vi "WVDIAL+HSRL_v3.0.vi"() -> ()   [LabVIEW 2012]
uses:
  C:/Users/H2ODial/Desktop/Shared Telescope WV DIAL Code/Libraries and VIs/PowerMeterCommands.dll
  Shared Telescope WV DIAL Code/Libraries and VIs/PowerMeterCommands.dll
  <vilib>/DAQmx/write.llb/DAQmx Write (Digital 1D Bool NChan 1Samp 1Line).vi
  <vilib>/DAQmx/miscellaneous.llb/DAQmx Fill In Error Info.vi
  <vilib>/Analysis/baseanly.llb/Mean (DBL).vi
  NCAR_DIAL_Labview/AMCS_Data.vi
  Libraries and VIs/Scalar_Data.vi
  <vilib>/Analysis/NI_AALBase.lvlib
  Libraries and VIs/Scalar_Data_2.vi
  Libraries and VIs/Scalar_Data_4.vi
  Libraries and VIs/Scalar_Data_3.vi
  Shared Telescope WV DIAL Code/bristol/CLDevIFace.dll
panel:
  out "FileHour":i32=15
  out "L_Count":i32=27488
  out "background start":u32=534
  in  "Tab Control 2":enum32{"WV ND narrow", "WV ND wide"}(tab)
  out "CH3 RingBuffer long":dbl[][](array[numeric])
  out "CH3 RingBuffer short":dbl[][](array[numeric])
  in  "?":T1(tab)=enum."Raw Counts combined"
  out "NRB":dbl[][](graph) caption="Water Vapor Number Density"
  out "NRB 2":dbl[][](graph) caption="Water Vapor Number Density"
  out "CH 1 (WV off) counts display":dbl[][](graph) caption="Water Vapor Number Density"
  out "CH 3 (HSRL comb) counts display":dbl[][](graph)=[[164.8800000000001, 18.88000000000011, -33.11999999999989, 47.88000000000011, 38.88000000000011, 9.88000000000011, -16.11999999999989, 5.880000000000109, 22.88000000000011, 52.88000000000011, 66.88000000000011, -8.11999999999989, 61.88000000000011, 39.88000000000011, 9.88000000000011, 43.88000000000011, 140.8800000000001, 54.88000000000011, 74.88000000000011, 70.88000000000011, 124.88000000000011, 78.88000000000011, 153.8800000000001, 125.88000000000011, 85.88000000000011, 158.8800000000001, 111.88000000000011, 58.88000000000011, 147.8800000000001, 45.88000000000011, 165.8800000000001, 52.88000000000011, 53.88000000000011, 74.88000000000011, 82.88000000000011, 122.88000000000011, 140.8800000000001, 99.88000000000011, 56.88000000000011, 185.8800000000001, 145.8800000000001, 78.88000000000011, 202.8800000000001, 100.88000000000011, 82.88000000000011, 137.8800000000001, 111.88000000000011, 148.8800000000001, 115.88000000000011, 68.88000000000011, 97.88000000000011, 143.8800000000001, 78.88000000000011, 196.8800000000001, 128.8800000000001, 253.8800000000001, 223.8800000000001, 537.8800000000001, 1045.88, 1637.88, 2013.88, 2171.88, 2511.88, 3252.88, 4089.88, 4490.88, 4802.88, 5302.88, 6838.88, 8530.880000000001, 9591.880000000001, 9526.880000000001, 8480.880000000001, 7901.88, 7867.88, 8171.88, 7794.88, 6264.88, 4513.88, 3105.88, 2225.88, 1878.88, 1881.88, 2124.88, 3090.88, 6012.88, 9343.880000000001, 11636.880000000001, 12784.880000000001, 11600.880000000001, 9980.880000000001, 8400.880000000001, 7022.88, 5983.88, 4614.88, 3348.88, 2472.88, 1514.88, 1053.88, 613.8800000000001, 658.8800000000001, 640.8800000000001, 586.8800000000001, 476.8800000000001, 200.8800000000001, 138.8800000000001, 158.8800000000001, -26.11999999999989, 129.8800000000001, 51.88000000000011, -45.11999999999989, -3.119999999999891, -4.119999999999891, 18.88000000000011, 23.88000000000011, -48.11999999999989, -32.11999999999989, -37.11999999999989, -7.119999999999891, -42.11999999999989, 74.88000000000011, 24.88000000000011, -21.11999999999989, -24.11999999999989, -4.119999999999891, -10.11999999999989, -22.11999999999989, -51.11999999999989, 79.88000000000011, -10.11999999999989, -82.11999999999989, -30.11999999999989, -1.1199999999998909, -31.11999999999989, -17.11999999999989, -7.119999999999891, -33.11999999999989, -10.11999999999989, -11.11999999999989, -35.11999999999989, -5.119999999999891, 75.88000000000011, -21.11999999999989, 31.88000000000011, -31.11999999999989, -16.11999999999989, -7.119999999999891, 43.88000000000011, -49.11999999999989, -72.11999999999989, 30.88000000000011, -12.11999999999989, 8.88000000000011, -15.11999999999989, -35.11999999999989, 53.88000000000011, 10.88000000000011, -39.11999999999989, 5.880000000000109, 16.88000000000011, -30.11999999999989, 25.88000000000011, -57.11999999999989, -54.11999999999989, 16.88000000000011, -50.11999999999989, 1.8800000000001091, -20.11999999999989, 19.88000000000011, -79.11999999999989, 50.88000000000011, -84.11999999999989, 8.88000000000011, -31.11999999999989, -27.11999999999989, 57.88000000000011, -45.11999999999989, 65.88000000000011, -45.11999999999989, -100.11999999999989, -2.119999999999891, -23.11999999999989, 60.88000000000011, -19.11999999999989, 12.88000000000011, -66.11999999999989, -76.11999999999989, -29.11999999999989, -31.11999999999989, -67.11999999999989, -3.119999999999891, -28.11999999999989, -46.11999999999989, -18.11999999999989, -21.11999999999989, 4.880000000000109, 14.88000000000011, -29.11999999999989, 54.88000000000011, 12.88000000000011, -38.11999999999989, -62.11999999999989, -35.11999999999989, 28.88000000000011, 8.88000000000011, -28.11999999999989, -14.11999999999989, 7.880000000000109, 32.88000000000011, 7.880000000000109, 3.880000000000109, 6.880000000000109, -56.11999999999989, -59.11999999999989, -18.11999999999989, -35.11999999999989, 22.88000000000011, -25.11999999999989, -2.119999999999891, -27.11999999999989, -4.119999999999891, 8.88000000000011, -82.11999999999989, -19.11999999999989, -58.11999999999989, -2.119999999999891, 6.880000000000109, -28.11999999999989, 35.88000000000011, -7.119999999999891, -45.11999999999989, -44.11999999999989, 4.880000000000109, -100.11999999999989, 40.88000000000011, -42.11999999999989, -72.11999999999989, -63.11999999999989, 52.88000000000011, -73.11999999999989, -35.11999999999989, -102.11999999999989, -22.11999999999989, -74.11999999999989, 64.88000000000011, 6.880000000000109, -37.11999999999989, -56.11999999999989, 16.88000000000011, 48.88000000000011, -28.11999999999989, 38.88000000000011, 69.88000000000011, -15.11999999999989, -41.11999999999989, 10.88000000000011, 39.88000000000011, 64.88000000000011, -67.11999999999989, 35.88000000000011, -25.11999999999989, 16.88000000000011, -58.11999999999989, -24.11999999999989, -35.11999999999989, 22.88000000000011, -25.11999999999989, -60.11999999999989, 18.88000000000011, 27.88000000000011, -31.11999999999989, 0.8800000000001091, -11.11999999999989, 5.880000000000109, 35.88000000000011, -13.11999999999989, -115.11999999999989, 55.88000000000011, -63.11999999999989, 45.88000000000011, -25.11999999999989, -46.11999999999989, -14.11999999999989, 18.88000000000011, -37.11999999999989, 40.88000000000011, -56.11999999999989, 71.88000000000011, -34.11999999999989, -11.11999999999989, 2.880000000000109, -77.11999999999989, -44.11999999999989, -44.11999999999989, -26.11999999999989, -111.11999999999989, 41.88000000000011, -64.11999999999989, 41.88000000000011, 47.88000000000011, -21.11999999999989, 43.88000000000011, -0.11999999999989086, -140.1199999999999, -27.11999999999989, -16.11999999999989, -24.11999999999989, -15.11999999999989, 25.88000000000011, -36.11999999999989, -3.119999999999891, -47.11999999999989, -33.11999999999989, -5.119999999999891, 41.88000000000011, -27.11999999999989, 19.88000000000011, -82.11999999999989, -63.11999999999989, 15.88000000000011, 19.88000000000011, 80.88000000000011, -15.11999999999989, 25.88000000000011, -48.11999999999989, -100.11999999999989, 13.88000000000011, 69.88000000000011, -75.11999999999989, 48.88000000000011, 59.88000000000011, -42.11999999999989, -2.119999999999891, 21.88000000000011, 11.88000000000011, -29.11999999999989, -28.11999999999989, 43.88000000000011, -61.11999999999989, -23.11999999999989, -21.11999999999989, -21.11999999999989, -57.11999999999989, -61.11999999999989, 1.8800000000001091, -91.11999999999989, -22.11999999999989, -48.11999999999989, 3.880000000000109, -39.11999999999989, -52.11999999999989, 9.88000000000011, 62.88000000000011, 14.88000000000011, -57.11999999999989, 15.88000000000011, -7.119999999999891, -53.11999999999989, 14.88000000000011, -3.119999999999891, -61.11999999999989, 34.88000000000011, 3.880000000000109, -46.11999999999989, -21.11999999999989, 57.88000000000011, -51.11999999999989, 15.88000000000011, -71.11999999999989, -92.11999999999989, 15.88000000000011, -13.11999999999989, -30.11999999999989, -24.11999999999989, -6.119999999999891, 59.88000000000011, 12.88000000000011, -41.11999999999989, -5.119999999999891, 43.88000000000011, 32.88000000000011, -21.11999999999989, -65.11999999999989, -18.11999999999989, -27.11999999999989, 43.88000000000011, 14.88000000000011, -83.11999999999989, 11.88000000000011, -30.11999999999989, -34.11999999999989, -5.119999999999891, -30.11999999999989, -13.11999999999989, -15.11999999999989, -36.11999999999989, 23.88000000000011, 65.88000000000011, -37.11999999999989, -54.11999999999989, -31.11999999999989, -66.11999999999989, -96.11999999999989, -1.1199999999998909, -2.119999999999891, -7.119999999999891, -5.119999999999891, 46.88000000000011, -8.11999999999989, -23.11999999999989, 29.88000000000011, -14.11999999999989, 20.88000000000011, -14.11999999999989, 3.880000000000109, 13.88000000000011, 38.88000000000011, -45.11999999999989, -16.11999999999989, 8.88000000000011, 19.88000000000011, 27.88000000000011, -57.11999999999989, -9.11999999999989, 35.88000000000011, -37.11999999999989, -22.11999999999989, -12.11999999999989, -1.1199999999998909, -27.11999999999989, 74.88000000000011, 9.88000000000011, 30.88000000000011, -72.11999999999989, 36.88000000000011, 9.88000000000011, -43.11999999999989, -65.11999999999989, -78.11999999999989, -50.11999999999989, -29.11999999999989, -51.11999999999989, -43.11999999999989, -4.119999999999891, -42.11999999999989, 6.880000000000109, -26.11999999999989, -56.11999999999989, -4.119999999999891, 5.880000000000109, -58.11999999999989, 14.88000000000011, 65.88000000000011, 32.88000000000011, 13.88000000000011, 7.880000000000109, 4.880000000000109, 85.88000000000011, 16.88000000000011, -23.11999999999989, -71.11999999999989, -98.11999999999989, -26.11999999999989, -25.11999999999989, 34.88000000000011, 80.88000000000011, 49.88000000000011, -32.11999999999989, -17.11999999999989, -15.11999999999989, -9.11999999999989, -53.11999999999989, 36.88000000000011, 13.88000000000011, -31.11999999999989, 26.88000000000011, 2.880000000000109, 14.88000000000011, -12.11999999999989, 14.88000000000011, -28.11999999999989, -35.11999999999989, 25.88000000000011, 33.88000000000011, -47.11999999999989, -32.11999999999989, -45.11999999999989, 66.88000000000011, -43.11999999999989, 58.88000000000011, -68.11999999999989, -39.11999999999989, -20.11999999999989, 64.88000000000011, 54.88000000000011, 35.88000000000011, -53.11999999999989, -29.11999999999989, -53.11999999999989, 43.88000000000011, 24.88000000000011, -3.119999999999891, 6.880000000000109, 17.88000000000011, 25.88000000000011, -79.11999999999989, 8.88000000000011, -16.11999999999989, -47.11999999999989, -15.11999999999989, 23.88000000000011, -21.11999999999989, -26.11999999999989, -59.11999999999989, -15.11999999999989, 3.880000000000109, -11.11999999999989, -26.11999999999989, -30.11999999999989, -44.11999999999989, 80.88000000000011, -18.11999999999989, -5.119999999999891, 89.88000000000011, -36.11999999999989, -31.11999999999989, -30.11999999999989, 64.88000000000011, -26.11999999999989, -60.11999999999989, -55.11999999999989, -18.11999999999989, -49.11999999999989, -16.11999999999989, 20.88000000000011, -40.11999999999989, 13.88000000000011, -25.11999999999989, -34.11999999999989, -56.11999999999989, 67.88000000000011, 92.88000000000011, 18.88000000000011, 40.88000000000011, 25.88000000000011, -7.119999999999891, -38.11999999999989, 15.88000000000011, -5.119999999999891, -12.11999999999989, -11.11999999999989, 9.88000000000011, -31.11999999999989, 14.88000000000011, -20.11999999999989, 12.88000000000011, -45.11999999999989, 1.8800000000001091, -11.11999999999989, 0.0]] caption="Water Vapor Number Density"
  out "CH3 (HSRL combined) smooth S":dbl[](array[numeric])=[62.141379310344824, 31.529310344827586, 26.45172413793103, 26.020689655172408, 24.39999999999999, 25.809482758620682, 28.13275862068965, 30.72327586206896, 35.654310344827586, 40.106896551724134, 42.68448275862069, 45.83965517241379, 50.41293103448277, 53.92155172413794, 58.7448275862069, 63.206034482758625, 64.82672413793105, 70.36551724137932, 75.06810344827588, 79.69310344827588, 90.12844827586208, 89.98189655172415, 95.59396551724139, 98.72758620689656, 96.86982758620692, 104.16293103448277, 104.7189655172414, 108.15862068965518, 110.34827586206896, 110.03793103448278, 112.66293103448277, 113.2448275862069, 118.46465517241379, 120.49913793103448, 121.40431034482759, 122.76206896551723, 118.72327586206896, 119.26206896551724, 118.48620689655172, 115.50344827586207, 113.28362068965518, 109.46034482758621, 107.28793103448277, 108.00775862068966, 109.01206896551724, 110.56379310344826, 112.92586206896551, 111.15431034482758, 112.26206896551724, 110.39137931034482, 108.54655172413794, 107.52068965517242, 107.51206896551724, 108.56379310344828, 113.12844827586206, 132.2232758620689, 168.06379310344818, 227.73189655172405, 313.503448275862, 420.3051724137932, 557.5077586206897, 733.4172413793104, 957.8784482758622, 1222.7706896551722, 1531.6155172413792, 1906.124137931034, 2328.4689655172415, 2784.990517241379, 3250.253448275862, 3651.374137931034, 3951.3525862068964, 4160.1586206896545, 4293.706034482759, 4410.766379310345, 4497.8396551724145, 4535.326724137931, 4491.2146551724145, 4321.055172413793, 4089.9905172413796, 3843.3568965517243, 3603.6499999999996, 3435.6844827586206, 3356.533620689655, 3340.813793103448, 3401.6025862068964, 3410.710344827586, 3283.3913793103447, 3033.921551724138, 2651.697413793103, 2298.0767241379303, 2079.374137931034, 2052.356896551724, 2349.675862068965, 3259.007758620689, 4998.356896551724, 7120.921551724138, 9052.218965517242, 9987.766379310346, 9388.059482758621, 7746.292241379311, 5710.9043103448275, 3920.503448275862, 2805.1025862068964, 2455.3439655172415, 2695.826724137931, 3198.8396551724136, 3763.0379310344824, 4047.585344827586, 3857.25775862069, 3344.3525862068964, 2535.1844827586206, 1635.1758620689657, 914.5422413793103, 406.45603448275864, 132.35689655172413, 36.546551724137935, 10.374137931034486, -1.1129310344827599, -2.367241379310346, -4.225000000000001, -5.255172413793105, -4.341379310344829, -6.931896551724138, -8.68189655172414, -7.582758620689656, -9.660344827586208, -8.634482758620692, -7.255172413793105, -7.281034482758622, -5.319827586206898, -4.880172413793105, -4.02241379310345, -7.750862068965519, -10.212068965517242, -9.966379310344829, -9.518103448275863, -6.77241379310345, -2.466379310344829, -1.5698275862068978, -3.6689655172413804, -4.341379310344829, -4.056896551724138, -6.505172413793105, -6.3931034482758635, -6.522413793103449, -10.569827586206898, -7.444827586206897, -5.548275862068968, -6.229310344827588, -1.8543103448275875, -2.8284482758620704, -4.031034482758622, -1.6431034482758633, -6.837068965517242, -3.630172413793104, 0.6801724137931027, 3.1974137931034474, 8.839655172413792, 6.753448275862067, 5.003448275862068, 2.3439655172413785, 0.2405172413793091, -0.06982758620689772, -0.535344827586208, -0.0568965517241391, -1.699137931034484, -3.4362068965517256, -3.2767241379310357, -4.255172413793105, -3.656034482758622, -2.1301724137931046, -3.4620689655172425, -4.492241379310346, -2.7853448275862083, -2.8198275862068978, -1.2465517241379322, 0.7534482758620678, -0.2939655172413805, -0.8198275862068978, -1.1215517241379322, -2.7767241379310357, -0.7896551724137941, 0.964655172413792, 3.7706896551724127, 4.550862068965516, 2.503448275862068, 1.0206896551724127, -2.1732758620689667, -3.3672413793103457, -5.160344827586208, -6.591379310344829, -7.074137931034484, -5.410344827586208, -5.095689655172416, -4.457758620689656, -2.565517241379312, -2.4706896551724147, -1.4189655172413804, -1.031034482758622, -3.3112068965517256, -3.6387931034482768, -4.64741379310345, -2.983620689655173, -2.5482758620689667, -4.802586206896553, -2.9060344827586215, -4.410344827586208, -5.156034482758622, -3.7681034482758635, -4.156034482758622, -4.186206896551726, -2.134482758620691, -2.781034482758622, -2.4362068965517256, -2.89741379310345, -5.160344827586208, -5.54396551724138, -5.048275862068967, -9.156034482758622, -8.436206896551726, -6.975000000000001, -8.065517241379311, -3.276724137931036, -4.1991379310344845, -5.660344827586208, -6.703448275862071, -6.651724137931036, -5.949137931034484, -6.138793103448277, -6.686206896551726, -9.289655172413795, -10.57844827586207, -9.018103448275863, -8.48793103448276, -7.358620689655174, -5.64741379310345, -5.427586206896553, -3.3974137931034494, -1.8284482758620701, -2.7336206896551736, -1.9879310344827597, -4.0310344827586215, -3.3198275862068978, -3.7939655172413804, -5.319827586206898, -3.367241379310346, -3.6258620689655183, -2.970689655172415, -3.513793103448277, -5.009482758620691, -5.660344827586208, -6.151724137931035, -7.5181034482758635, -7.776724137931036, -8.186206896551726, -6.802586206896554, -3.9577586206896562, -2.8974137931034494, -1.1129310344827599, -1.552586206896553, -3.0181034482758635, -4.160344827586209, -4.888793103448277, -3.867241379310346, -2.3974137931034494, -1.2681034482758633, -1.927586206896553, -3.3198275862068978, -5.138793103448277, -5.4620689655172425, -5.108620689655174, -3.018103448275863, -3.0051724137931046, -3.996551724137932, -5.285344827586209, -8.457758620689656, -7.975000000000001, -7.1991379310344845, -5.177586206896553, -3.3112068965517256, -2.841379310344829, -3.466379310344829, -5.64741379310345, -6.742241379310347, -6.854310344827588, -5.483620689655174, -2.427586206896553, -0.25948275862069076, 0.18017241379310245, -1.1043103448275873, -4.9060344827586215, -6.121551724137932, -7.621551724137932, -5.660344827586208, -5.005172413793105, -5.561206896551725, -2.6991379310344836, -5.54396551724138, -4.048275862068967, -3.7379310344827594, -4.699137931034484, -2.4017241379310357, -2.6603448275862083, -4.246551724137932, -4.742241379310346, -4.272413793103449, -2.8241379310344836, 0.007758620689653939, -0.6301724137931046, -1.7250000000000012, -3.4491379310344836, -4.138793103448277, -1.6603448275862078, -4.035344827586208, -4.608620689655174, -6.125862068965518, -9.811206896551726, -8.93189655172414, -8.457758620689656, -6.845689655172415, -3.720689655172415, -1.4405172413793117, -1.3586206896551736, -1.7637931034482772, -3.565517241379312, -4.479310344827588, -1.6732758620689665, -0.3025862068965528, 2.6931034482758607, 4.83103448275862, 2.5982758620689648, 3.5120689655172397, 1.0379310344827573, 0.45603448275861946, 1.4344827586206885, -2.3974137931034494, -4.574137931034484, -4.686206896551725, -5.617241379310345, -4.000862068965518, -3.302586206896553, -3.86293103448276, -4.888793103448277, -7.207758620689656, -6.190517241379311, -6.00948275862069, -3.45344827586207, -1.8758620689655183, -2.720689655172415, -0.6474137931034494, -0.9620689655172425, -1.7551724137931046, 0.9215517241379299, -2.61293103448276, -3.9405172413793115, -2.45344827586207, -4.910344827586208, -4.160344827586208, -4.513793103448276, -4.479310344827587, -0.5008620689655185, -1.3241379310344839, -0.13017241379310468, -1.3025862068965528, -3.9706896551724147, -1.7724137931034492, -2.3801724137931046, -1.8758620689655183, -0.7508620689655184, -3.013793103448277, -2.5439655172413804, -1.2336206896551736, -1.0612068965517254, -2.539655172413794, -1.3974137931034498, -1.901724137931036, -2.2465517241379325, 0.9344827586206884, -1.746551724137932, -2.1948275862068973, -2.2939655172413804, -5.018103448275863, -4.888793103448277, -4.789655172413794, -5.388793103448277, -2.393103448275863, -0.7551724137931046, 2.1284482758620675, 1.6887931034482746, 0.30086206896551615, 0.8870689655172401, -0.4577586206896561, -1.3370689655172425, -0.1775862068965529, 0.701724137931033, -1.5956896551724151, -0.7206896551724149, 1.0551724137931022, -2.3068965517241393, -0.28534482758620805, -1.4793103448275875, -4.595689655172415, -3.970689655172415, -4.77241379310345, -3.5827586206896562, -4.341379310344829, -2.8068965517241393, -4.746551724137932, -3.2336206896551736, -1.4232758620689667, -1.0698275862068976, 0.3051724137931022, 0.19741379310344698, -0.6000000000000012, -4.074137931034484, -5.2120689655172425, -3.565517241379311, -3.341379310344829, -2.789655172413794, -1.720689655172415, -4.9060344827586215, -3.3801724137931046, -0.7508620689655183, -0.6344827586206908, -0.7508620689655184, -1.7637931034482772, -3.345689655172415, -1.20344827586207, 0.257758620689654, -2.1732758620689667, -3.7422413793103457, -3.7594827586206905, -4.518103448275863, -1.8801724137931046, -0.263793103448277, -2.32844827586207, -2.281034482758622, -1.6431034482758633, -0.6948275862068977, 0.24482758620689538, 1.4517241379310333, -1.4060344827586218, -3.8586206896551736, -5.66896551724138, -9.436206896551726, -8.535344827586208, -8.143103448275864, -5.957758620689656, -3.7336206896551736, -2.5310344827586215, -2.0267241379310357, -3.8758620689655183, -4.341379310344829, -4.664655172413794, -2.2939655172413804, -0.7551724137931045, -1.5482758620689665, -0.9362068965517253, -3.871551724137932, -3.2724137931034494, -4.54396551724138, -4.160344827586208, -2.6215517241379316, -4.005172413793105, -4.841379310344829, -5.638793103448277, -4.880172413793105, -5.052586206896553, -1.6991379310344839, -2.931896551724139, -0.9146551724137946, -1.6732758620689667, 0.17586206896551593, 1.9043103448275849, -2.0224137931034494, -1.9275862068965528, -3.281034482758622, -2.6948275862068973, -1.4663793103448288, -1.931896551724139, -2.8112068965517256, -2.5655172413793115, -2.95344827586207, -2.39741379310345, -1.3284482758620701, -3.6129310344827603, -1.9577586206896562, -1.406034482758622, 0.6499999999999986, 1.8913793103448264, 1.5077586206896538, 2.6887931034482744, 1.3913793103448264, -0.6862068965517252, -1.0353448275862078, -1.5913793103448286, -3.2551724137931046, -0.867241379310346, -3.466379310344829, -3.4017241379310352, -2.6387931034482768, -3.41896551724138, 0.22327586206896433, 0.024999999999998856, 0.6112068965517229, 1.1198275862068952, -0.01810344827586323, 0.23620689655172294, -0.5396551724137942, -0.3844827586206908, -1.5008620689655183, -2.268103448275863, -1.470689655172415, -0.5051724137931046, -3.2982758620689667, -3.89741379310345, -5.207758620689657, -5.64741379310345, -4.216379310344829, -2.664655172413794, -1.8974137931034494, -3.733620689655173, 0.3008620689655159, 0.447413793103447, -0.4706896551724151, -0.3974137931034496, -1.5741379310344839, -1.462068965517243, -1.7034482758620704, -0.5784482758620703, -2.1732758620689667, -2.7508620689655188, -1.216379310344829, -1.6215517241379325, 0.14568965517241256, -2.4146551724137946, -3.2724137931034494, -4.574137931034484, -5.039655172413794, -1.7637931034482768, -1.302586206896553, -0.22931034482758744, 0.016379310344826425, 2.1413793103448264, 3.2879310344827575, 7.0379310344827575, 7.378448275862068, 4.124137931034483, 4.352586206896551, -1.9448275862068978, -2.621551724137932, -0.9836206896551738, -3.315517241379312, 0.3094827586206884, -0.13448275862069092]
  out "CH3 (HSRL combined) smooth L":dbl[](array[numeric])=[58.96740223463691, 30.528854748603358, 26.30259776536313, 25.398966480446923, 26.19924581005587, 28.14128491620113, 31.917821229050297, 35.773966480446944, 38.952039106145264, 43.03164804469274, 45.771871508379874, 49.793519553072606, 54.13290502793292, 58.55399441340778, 63.422011173184316, 66.78723463687146, 70.81656424581001, 75.89198324022342, 81.08751396648043, 87.51000000000002, 94.17550279329615, 96.72298882681572, 99.86963687150848, 102.128715083799, 102.95483240223473, 106.73346368715093, 109.06516759776547, 111.84729050279341, 113.71740223463698, 115.26628491620124, 116.84729050279341, 117.8682402234638, 120.69924581005597, 122.06446927374313, 121.85287709497219, 121.37173184357553, 120.16642458100571, 119.63569832402247, 120.57424581005598, 119.83053072625712, 118.6706145251398, 118.24393854748615, 117.05608938547499, 117.50441340782133, 117.44715083798894, 116.36614525139676, 115.9241061452515, 114.49114525139677, 113.32564245810067, 112.08891061452525, 110.22438547486043, 109.14268156424592, 108.67899441340792, 107.6636312849163, 107.48067039106155, 108.75092178770961, 113.20553072625711, 123.05748603351967, 138.2481284916202, 161.0498044692738, 195.15874301675976, 242.8947765363128, 307.6021787709496, 393.1147486033518, 510.0721508379887, 670.1713128491618, 886.0833240223462, 1157.165027932961, 1461.3277374301679, 1772.6559497206706, 2047.1084636871512, 2275.5742458100563, 2487.52466480447, 2717.0079050279337, 3005.227178770951, 3358.319357541901, 3782.7187988826836, 4288.426899441343, 4938.4653072625715, 5706.315167597768, 6396.585418994415, 6793.38150837989, 6685.923407821231, 6074.914329608941, 5150.7425418994435, 4146.376620111734, 3238.7278770949733, 2492.519078212291, 1941.3745251396651, 1591.3130726256984, 1403.3235474860332, 1331.2341620111729, 1334.692262569832, 1419.8410055865918, 1635.531648044692, 1933.3437988826804, 2246.5602793296075, 2466.9115363128476, 2500.166424581004, 2396.391983240222, 2204.0302513966467, 1983.4534357541888, 1790.1503631284907, 1649.0770391061444, 1564.5679608938538, 1492.7187988826809, 1414.2362569832394, 1292.0016201117312, 1113.9541340782118, 916.6587430167594, 700.9548324022344, 490.7655865921786, 310.70553072625694, 167.7208938547486, 75.49324022346364, 28.379413407821218, 9.123826815642452, 3.8605586592178742, 2.8221508379888243, 2.2250837988826784, 2.0972905027932933, 1.8787150837988795, 1.530949720670388, 0.16921787709497016, 0.8849999999999977, 0.4164245810055844, 0.5686592178770926, 1.1622346368715053, 0.6126536312849132, 0.7327653631284886, 0.559581005586589, 0.660837988826812, -0.4823184357541942, -0.9529888268156467, -1.351033519553077, -1.135949720670395, -0.23022346368715413, -0.09893854748603678, -0.01793296089385804, -0.4348324022346404, -0.7085754189944173, -0.33986033519553455, -0.1380446927374338, -0.7316201117318467, -0.1820391061452541, 0.5211731843575392, 1.4464525139664774, 4.6922625698323985, 8.21670391061452, 18.669217877094965, 40.91432960893853, 83.42829608938547, 154.14128491620113, 247.91363128491622, 355.9764804469274, 453.57005586592174, 521.1405865921787, 554.2865363128491, 557.3158659217877, 547.9485474860335, 538.4045530726257, 532.9282960893854, 531.5623743016758, 527.4764804469273, 519.1238268156424, 503.9632122905028, 478.56097765363126, 444.4164245810056, 403.6559497206704, 358.57354748603353, 310.4268994413408, 261.56377094972066, 212.2697765363129, 165.0700558659218, 121.86963687150842, 87.4946368715084, 61.542122905027924, 43.46391061452513, 34.2118156424581, 29.90175977653631, 27.326340782122905, 28.481368715083804, 34.119636871508376, 42.34798882681564, 51.39058659217876, 56.27885474860333, 54.19226256983239, 44.528156424581, 33.469497206703906, 21.27885474860335, 11.035139664804463, 4.852178770949717, 0.5030167597765325, -0.8838547486033554, -1.637346368715087, -1.8894413407821258, -2.0402793296089414, -1.2141620111731872, -2.103128491620116, -2.4941899441340825, -2.941117318435759, -4.0004748603352, -3.514441340782127, -3.8007541899441377, -3.942513966480451, -3.430642458100563, -3.0263128491620144, -2.916675977653635, -2.645027932960897, -3.1925139664804503, -3.1869273743016793, -2.8901396648044724, -3.1268715083798915, -3.0933519553072655, -3.1869273743016784, -3.2979608938547513, -4.374776536312853, -3.97533519553073, -3.894329608938551, -3.704385474860339, -2.1359497206703946, -2.020027932960897, -2.683435754189948, -2.6841340782122938, -2.5786871508379923, -3.0291061452514003, -2.5535474860335228, -2.59055865921788, -2.7679329608938574, -3.5703072625698358, -2.288184357541903, -2.0563407821229083, -1.3342737430167633, -1.1876256983240254, -2.2874860335195564, -1.8566201117318466, -2.2749162011173216, -1.4893016759776563, -0.9285474860335223, -1.6904189944134107, -0.9920949720670421, -1.1024301675977681, -1.1045251396648073, -0.4341340782122932, -2.0053631284916236, -2.0668156424581037, -2.637346368715087, -4.333575418994419, -4.084972067039112, -4.163184357541905, -4.462765363128497, -3.8000558659217916, -3.6478212290502827, -4.200195530726261, -4.091955307262574, -3.3217039106145294, -3.767234636871513, -3.218351955307266, -2.142932960893858, -1.722541899441344, -1.1408379888268183, -0.5926536312849189, -1.0367877094972096, -1.8461452513966505, -1.5954469273743042, -1.7916759776536337, -1.3538268156424607, -0.8761731843575447, -1.640139664804472, -1.8559217877095, -2.1939106145251426, -2.7483798882681594, -1.8698882681564275, -1.5067597765363157, -2.573798882681568, -1.8014525139664836, -1.9432122905027964, -2.209273743016763, -1.0884636871508406, -1.302849162011176, -1.2141620111731872, -1.6813407821229078, -1.876871508379891, -1.2846927374301702, -1.7036871508379916, -1.0172346368715113, -1.237905027932964, -1.4564804469273773, -0.7232402234636901, -0.6156983240223493, -0.5011731843575447, -0.5123463687150864, -0.29446927374301946, -0.462067039106148, -0.5409776536312876, -0.6031284916201144, -1.4913966480446954, -2.301452513966484, -2.2406983240223495, -2.5242178770949755, -2.45019553072626, -1.2351117318435783, -0.9020111731843603, -1.1506145251396676, -1.026312849162014, -1.2881843575419023, -1.5682122905027962, -1.5235195530726284, -0.6771508379888296, -0.6408379888268183, -0.6254748603351983, -0.6687709497206733, -0.5675139664804496, -1.0758938547486059, -1.1436312849162036, -0.8964245810055891, -2.6869273743016784, -3.1401396648044724, -3.064720670391065, -2.3098324022346404, -1.7958659217877129, -0.9879050279329638, -0.8021508379888297, -1.5912569832402264, -1.7616480446927407, -1.9858100558659249, -2.3314804469273778, -2.448100558659221, -0.8712849162011199, -0.2979608938547512, -0.15829608938547757, -0.39293296089385726, -0.9739385474860361, -1.3559217877094998, -1.0465642458100584, -0.5221229050279357, -1.4446089385474892, -0.8929329608938581, -0.9557821229050311, -1.601033519553076, -1.7448882681564277, -2.132458100558662, -2.536089385474863, -1.708575418994416, -0.7525698324022374, -1.3698882681564273, -0.9886033519553099, -0.99628491620112, -1.4536871508379914, -1.658994413407824, -1.7770111731843605, -1.6003351955307292, -1.1687709497206733, -0.20229050279329883, -0.6624860335195558, -0.29516759776536583, -0.46206703910614794, -0.3307821229050306, -0.34055865921788, -1.1764525139664834, -1.1450279329608968, -1.3705865921787737, -0.29796089385475133, 0.30329608938547215, 0.8102793296089359, 0.9457541899441313, 0.8570670391061425, -0.031201117318438443, -0.4669553072625725, -0.8489385474860361, -0.8936312849162038, -0.9257541899441368, -0.8971229050279358, -1.0877653631284945, -1.1254748603351983, -0.6883240223463716, -0.5416759776536341, 0.0037150837988799527, -0.9055027932960922, -1.0772905027932989, -1.2008938547486059, -1.626871508379891, -0.9138826815642486, -1.4278491620111762, -1.1771508379888296, -1.6136033519553103, -1.5423743016759806, -0.6841340782122936, -1.21555865921788, -1.3985195530726289, -1.7686312849162045, -1.5905586592178804, -1.6701675977653663, -0.6359497206703938, 0.07843575418994136, -0.6548044692737458, -0.4208659217877122, -0.3943296089385502, -0.9257541899441368, -0.462067039106148, -0.8643016759776563, -1.4292458100558685, -1.5835754189944158, -2.0996368715083826, -2.240698324022349, -2.198798882681567, -2.2490782122905055, -2.397821229050282, -1.3161173184357569, -0.6513128491620137, -0.7274301675977679, 0.18737430167597494, 0.21810055865921515, 0.6294134078212263, 0.4953351955307237, -0.4669553072625734, 0.155251396648041, -0.7406983240223501, -1.0249162011173223, -0.48511173184357875, -0.932737430167601, -0.05703910614525454, 0.31307262569832106, -0.23860335195531002, -1.0228212290502823, -1.5263128491620142, -0.8279888268156453, -0.12826815642458378, 1.060977653631282, -0.045167597765366274, -1.0339944134078247, -0.9976815642458136, -2.492793296089389, -1.8887430167597796, -1.3314804469273769, -1.626871508379891, -0.7358100558659244, -0.33287709497206974, -0.0039664804469300985, 0.26279329608938273, -0.12058659217877371, 0.33192737430167324, -0.4390223463687179, -0.9166759776536342, -1.388044692737433, -2.557737430167601, -3.277011173184361, -2.368491620111735, -2.0982402234636903, -1.675055865921791, -0.41877094972067314, -1.2895810055865948, -1.7204469273743044, -1.1464245810055893, -1.6638826815642487, -0.6841340782122931, -0.34125698324022613, -0.9201675977653657, -0.7574581005586618, -0.6541061452513992, -1.3810614525139697, 0.003715083798879082, -0.011648044692741, -0.6855307262569867, 0.038631284916197994, -1.23860335195531, -0.4969832402234664, 0.25441340782122623, 0.44156424581005305, 0.17340782122904752, 0.6992458100558631, 0.6189385474860307, 1.0630726256983212, 1.7900279329608912, 1.5651675977653605, 0.9443575418994384, 1.6768994413407792, 2.4792737430167566, 2.402458100558656, 1.0351396648044655, -0.02910614525140011, -0.9222625698324055, -1.5402793296089416, -0.2427932960893882, 0.023268156424578273, -0.16737430167598039, -0.06122905027933234, 0.3843016759776509, -0.08706703910614796, 0.3214525139664777, 0.45483240223463417, 0.5937988826815616, 1.5016201117318408, 0.5058100558659189, 0.9338826815642429, 0.6671229050279301, -0.26094972067039396, 0.31377094972066766, -0.028407821229053054, -0.2504748603351983, 0.7648882681564216, 2.146871508379885, 2.530949720670388, 3.4660055865921757, 2.765586592178768, 1.6901675977653603, 1.3766201117318406, 0.6035754189944106, -0.19879888268156753, -0.3985195530726289, -0.8133240223463719, -1.5109497206703946, -1.3566201117318468, -1.4006145251396678, -2.1939106145251435, -1.5968435754189976, -0.8950279329608972, -0.1694692737430209, 0.7998044692737394, 1.4192178770949686, 1.0218715083798846, 0.2243854748603325, 1.0861173184357515, 0.7111173184357517, 1.0728491620111706, 1.2579050279329582, 0.571452513966478, 0.3514804469273715, 0.7704748603351927, 0.74603351955307, 0.1824860335195504, -0.4425139664804497, -1.0367877094972096, -1.0968435754189971, -0.869189944134081, -0.9851117318435784, -0.7777094972067068, -1.4697486033519582, -1.1694692737430197, -0.7832960893854776, -0.5675139664804496, 0.46391061452513693, -0.031201117318438498, 0.7732681564245782, 1.4171229050279304, 1.4513407821229025, 2.463212290502791, 1.8319273743016735, 1.0574860335195506, 0.5518994413407796, 0.16502793296089113, 0.5044134078212263, -0.34614525139665087, -0.08357541899441631, -0.5032681564245839]
  out "CH3 Bin Readings":dbl[](array[numeric])=[2030.0, 1884.0, 1832.0, 1913.0, 1904.0, 1875.0, 1849.0, 1871.0, 1888.0, 1918.0, 1932.0, 1857.0, 1927.0, 1905.0, 1875.0, 1909.0, 2006.0, 1920.0, 1940.0, 1936.0, 1990.0, 1944.0, 2019.0, 1991.0, 1951.0, 2024.0, 1977.0, 1924.0, 2013.0, 1911.0, 2031.0, 1918.0, 1919.0, 1940.0, 1948.0, 1988.0, 2006.0, 1965.0, 1922.0, 2051.0, 2011.0, 1944.0, 2068.0, 1966.0, 1948.0, 2003.0, 1977.0, 2014.0, 1981.0, 1934.0, 1963.0, 2009.0, 1944.0, 2062.0, 1994.0, 2119.0, 2089.0, 2403.0, 2911.0, 3503.0, 3879.0, 4037.0, 4377.0, 5118.0, 5955.0, 6356.0, 6668.0, 7168.0, 8704.0, 10396.0, 11457.0, 11392.0, 10346.0, 9767.0, 9733.0, 10037.0, 9660.0, 8130.0, 6379.0, 4971.0, 4091.0, 3744.0, 3747.0, 3990.0, 4956.0, 7878.0, 11209.0, 13502.0, 14650.0, 13466.0, 11846.0, 10266.0, 8888.0, 7849.0, 6480.0, 5214.0, 4338.0, 3380.0, 2919.0, 2479.0, 2524.0, 2506.0, 2452.0, 2342.0, 2066.0, 2004.0, 2024.0, 1839.0, 1995.0, 1917.0, 1820.0, 1862.0, 1861.0, 1884.0, 1889.0, 1817.0, 1833.0, 1828.0, 1858.0, 1823.0, 1940.0, 1890.0, 1844.0, 1841.0, 1861.0, 1855.0, 1843.0, 1814.0, 1945.0, 1855.0, 1783.0, 1835.0, 1864.0, 1834.0, 1848.0, 1858.0, 1832.0, 1855.0, 1854.0, 1830.0, 1860.0, 1941.0, 1844.0, 1897.0, 1834.0, 1849.0, 1858.0, 1909.0, 1816.0, 1793.0, 1896.0, 1853.0, 1874.0, 1850.0, 1830.0, 1919.0, 1876.0, 1826.0, 1871.0, 1882.0, 1835.0, 1891.0, 1808.0, 1811.0, 1882.0, 1815.0, 1867.0, 1845.0, 1885.0, 1786.0, 1916.0, 1781.0, 1874.0, 1834.0, 1838.0, 1923.0, 1820.0, 1931.0, 1820.0, 1765.0, 1863.0, 1842.0, 1926.0, 1846.0, 1878.0, 1799.0, 1789.0, 1836.0, 1834.0, 1798.0, 1862.0, 1837.0, 1819.0, 1847.0, 1844.0, 1870.0, 1880.0, 1836.0, 1920.0, 1878.0, 1827.0, 1803.0, 1830.0, 1894.0, 1874.0, 1837.0, 1851.0, 1873.0, 1898.0, 1873.0, 1869.0, 1872.0, 1809.0, 1806.0, 1847.0, 1830.0, 1888.0, 1840.0, 1863.0, 1838.0, 1861.0, 1874.0, 1783.0, 1846.0, 1807.0, 1863.0, 1872.0, 1837.0, 1901.0, 1858.0, 1820.0, 1821.0, 1870.0, 1765.0, 1906.0, 1823.0, 1793.0, 1802.0, 1918.0, 1792.0, 1830.0, 1763.0, 1843.0, 1791.0, 1930.0, 1872.0, 1828.0, 1809.0, 1882.0, 1914.0, 1837.0, 1904.0, 1935.0, 1850.0, 1824.0, 1876.0, 1905.0, 1930.0, 1798.0, 1901.0, 1840.0, 1882.0, 1807.0, 1841.0, 1830.0, 1888.0, 1840.0, 1805.0, 1884.0, 1893.0, 1834.0, 1866.0, 1854.0, 1871.0, 1901.0, 1852.0, 1750.0, 1921.0, 1802.0, 1911.0, 1840.0, 1819.0, 1851.0, 1884.0, 1828.0, 1906.0, 1809.0, 1937.0, 1831.0, 1854.0, 1868.0, 1788.0, 1821.0, 1821.0, 1839.0, 1754.0, 1907.0, 1801.0, 1907.0, 1913.0, 1844.0, 1909.0, 1865.0, 1725.0, 1838.0, 1849.0, 1841.0, 1850.0, 1891.0, 1829.0, 1862.0, 1818.0, 1832.0, 1860.0, 1907.0, 1838.0, 1885.0, 1783.0, 1802.0, 1881.0, 1885.0, 1946.0, 1850.0, 1891.0, 1817.0, 1765.0, 1879.0, 1935.0, 1790.0, 1914.0, 1925.0, 1823.0, 1863.0, 1887.0, 1877.0, 1836.0, 1837.0, 1909.0, 1804.0, 1842.0, 1844.0, 1844.0, 1808.0, 1804.0, 1867.0, 1774.0, 1843.0, 1817.0, 1869.0, 1826.0, 1813.0, 1875.0, 1928.0, 1880.0, 1808.0, 1881.0, 1858.0, 1812.0, 1880.0, 1862.0, 1804.0, 1900.0, 1869.0, 1819.0, 1844.0, 1923.0, 1814.0, 1881.0, 1794.0, 1773.0, 1881.0, 1852.0, 1835.0, 1841.0, 1859.0, 1925.0, 1878.0, 1824.0, 1860.0, 1909.0, 1898.0, 1844.0, 1800.0, 1847.0, 1838.0, 1909.0, 1880.0, 1782.0, 1877.0, 1835.0, 1831.0, 1860.0, 1835.0, 1852.0, 1850.0, 1829.0, 1889.0, 1931.0, 1828.0, 1811.0, 1834.0, 1799.0, 1769.0, 1864.0, 1863.0, 1858.0, 1860.0, 1912.0, 1857.0, 1842.0, 1895.0, 1851.0, 1886.0, 1851.0, 1869.0, 1879.0, 1904.0, 1820.0, 1849.0, 1874.0, 1885.0, 1893.0, 1808.0, 1856.0, 1901.0, 1828.0, 1843.0, 1853.0, 1864.0, 1838.0, 1940.0, 1875.0, 1896.0, 1793.0, 1902.0, 1875.0, 1822.0, 1800.0, 1787.0, 1815.0, 1836.0, 1814.0, 1822.0, 1861.0, 1823.0, 1872.0, 1839.0, 1809.0, 1861.0, 1871.0, 1807.0, 1880.0, 1931.0, 1898.0, 1879.0, 1873.0, 1870.0, 1951.0, 1882.0, 1842.0, 1794.0, 1767.0, 1839.0, 1840.0, 1900.0, 1946.0, 1915.0, 1833.0, 1848.0, 1850.0, 1856.0, 1812.0, 1902.0, 1879.0, 1834.0, 1892.0, 1868.0, 1880.0, 1853.0, 1880.0, 1837.0, 1830.0, 1891.0, 1899.0, 1818.0, 1833.0, 1820.0, 1932.0, 1822.0, 1924.0, 1797.0, 1826.0, 1845.0, 1930.0, 1920.0, 1901.0, 1812.0, 1836.0, 1812.0, 1909.0, 1890.0, 1862.0, 1872.0, 1883.0, 1891.0, 1786.0, 1874.0, 1849.0, 1818.0, 1850.0, 1889.0, 1844.0, 1839.0, 1806.0, 1850.0, 1869.0, 1854.0, 1839.0, 1835.0, 1821.0, 1946.0, 1847.0, 1860.0, 1955.0, 1829.0, 1834.0, 1835.0, 1930.0, 1839.0, 1805.0, 1810.0, 1847.0, 1816.0, 1849.0, 1886.0, 1825.0, 1879.0, 1840.0, 1831.0, 1809.0, 1933.0, 1958.0, 1884.0, 1906.0, 1891.0, 1858.0, 1827.0, 1881.0, 1860.0, 1853.0, 1854.0, 1875.0, 1834.0, 1880.0, 1845.0, 1878.0, 1820.0, 1867.0, 1854.0]
  out "CH2 (molecular) smoothed":dbl[](array[numeric])=[7.959767441860434, -0.34643410852716383, 1.2349612403100454, 2.0004651162790377, -2.3193023255814276, -0.15844961240313304, -0.36387596899228014, -0.43170542635662146, 4.03534883720927, 4.942325581395316, 7.733023255813921, 6.4830232558139205, 7.05472868217051, 8.40550387596896, 9.287286821705393, 13.316356589147254, 15.479147286821672, 21.091550387596868, 24.225271317829428, 28.459767441860436, 34.8841860465116, 37.20589147286819, 42.33767441860463, 49.87449612403099, 54.79891472868216, 58.36480620155038, 57.944263565891475, 57.00046511627907, 55.21170542635659, 54.924883720930225, 58.93457364341084, 57.61868217054263, 59.86286821705426, 62.04310077519379, 59.6884496124031, 63.67682170542634, 61.143875968992226, 63.508217054263525, 63.37449612403097, 61.40162790697672, 61.277596899224775, 58.775658914728666, 59.65937984496123, 58.11480620155037, 60.07217054263565, 60.26790697674417, 58.67488372093021, 59.19813953488371, 58.19813953488371, 55.494651162790696, 55.37255813953488, 56.771782945736426, 55.47914728682169, 54.24852713178293, 53.63806201550386, 51.012093023255794, 50.7950387596899, 49.03728682170541, 51.88031007751937, 54.56441860465115, 60.58767441860464, 72.16713178294572, 79.50046511627903, 92.11674418604646, 108.56829457364333, 130.47139534883715, 162.59155038759684, 202.34155038759678, 250.81829457364336, 300.453953488372, 345.1128682170542, 383.97720930232555, 408.5896124031008, 426.54310077519375, 449.8105426356589, 473.3609302325582, 504.32798449612403, 553.2272093023255, 626.2117054263565, 733.031472868217, 844.4055038759691, 908.4849612403102, 882.6806976744186, 760.9074418604652, 592.5004651162791, 442.92100775193796, 340.59542635658914, 286.4927131782946, 262.71558139534875, 245.7872868217053, 239.9268217054262, 237.23108527131768, 231.15937984496108, 213.61093023255796, 189.3221705426355, 161.92875968992234, 134.20395348837195, 107.43651162790687, 77.39387596899216, 46.87062015503871, 23.037286821705404, 7.008217054263534, -2.1080620155039083, -1.4220155038760016, -4.222403100775226, -1.8464341085271636, -2.5634883720930555, -6.7010852713178615, -5.662325581395382, -4.303798449612435, -1.4472093023256134, 0.5818604651162469, -0.673953488372125, -5.377441860465149, -7.865813953488405, -8.96465116279073, -8.94139534883724, -9.610000000000031, -10.42589147286825, -9.228217054263597, -7.5925581395349155, -3.5344186046511945, -3.95496124031011, -3.97434108527135, -4.910387596899257, -8.332868217054296, -7.080930232558172, -10.288294573643444, -10.338682170542668, -8.203023255813985, -5.976279069767474, -4.098372093023288, -4.786356589147319, -6.230155038759722, -8.803798449612435, -7.852248062015535, -6.722403100775225, -6.735968992248094, -6.011162790697706, -7.555736434108559, -8.695271317829489, -7.024728682170574, -8.047984496124062, -6.2592248062015825, -5.538294573643443, -4.7592248062015825, -4.187519379844993, -6.03248062015507, -6.538294573643443, -6.261162790697707, -4.3464341085271645, -3.931705426356621, -5.547984496124063, -5.960775193798482, -5.040232558139568, -4.201085271317862, 1.0566666666666347, 0.7775968992247739, -2.2689147286822022, -1.5867441860465434, -6.098372093023288, -5.0596124031008065, -4.848372093023288, -5.282480620155072, -3.807674418604683, -4.850310077519412, -2.980155038759722, -3.288294573643443, -1.2107751937984816, -1.3793798449612724, -4.639069767441892, -4.354186046511661, -5.906511627907009, -7.036356589147319, -5.590620155038792, -4.394883720930265, -4.666201550387629, -3.8134883720930555, -3.9568992248062336, -5.697209302325613, -4.834806201550419, -4.48403100775197, -6.168139534883753, -4.371627906976776, -5.222403100775226, -6.807674418604684, -5.282480620155071, -9.042170542635692, -11.315426356589178, -9.827054263565923, -9.770852713178327, -8.571240310077552, -8.020852713178327, -10.25341085271321, -9.232093023255846, -8.33480620155042, -5.68558139534887, -4.183643410852745, -4.995658914728715, -2.8503100775194117, -4.346434108527164, -1.162325581395381, -0.4103875968992571, -2.1720155038760014, 0.9113178294573323, -2.338682170542668, -3.920077519379877, -6.1758914728682495, -7.598372093023287, -6.03248062015507, -5.588682170542668, -3.1061240310077842, -4.367751937984528, -5.937519379844993, -4.499534883720962, -4.0925581395349155, -4.414263565891505, -3.117751937984528, -1.658449612403133, -2.534418604651195, -1.6410077519380168, -3.4685271317829782, -5.24372093023259, -4.313488372093056, -6.100310077519412, -2.6603875968992567, -1.3037984496124353, -2.185581395348869, 0.6787596899224484, -1.6758914728682495, -2.900697674418637, -3.679767441860497, -4.274728682170575, -5.406511627907008, -4.456899224806233, -3.982093023255846, -3.416201550387629, -0.4975968992248383, -2.2766666666666993, -1.3134883720930557, -3.0460465116279396, -3.078992248062048, -0.9258914728682491, -2.0092248062015825, -3.9375193798449937, -7.8173643410853035, -7.999534883720962, -8.520852713178327, -6.3425581395349155, -4.191395348837242, -4.7340310077519705, -0.20689922480623357, 0.7543410852712856, 0.9113178294573321, -0.08286821705429581, -5.057674418604684, -8.385193798449645, -9.098372093023288, -6.077054263565923, -2.2224031007752254, 0.35317829457361116, 0.9539534883720608, -1.284418604651195, -3.7669767441860786, -2.5111627906977065, -0.23209302325584624, -2.402635658914761, -2.710775193798482, -4.055736434108559, -4.52279069767445, -0.8696899224806521, -0.10806201550390804, 2.2834108527131463, 1.207829457364309, 0.3725581395348516, 1.6710077519379523, -0.3037984496124353, -1.1371317829457686, 0.07410852713175076, 0.07798449612399888, -0.282480620155071, -1.3774418604651486, -2.72434108527135, -1.338682170542668, -1.4607751937984819, 0.6729457364340764, 0.7233333333333014, -3.1332558139535207, -2.5751162790697997, -4.2882945736434435, -2.3251162790698006, -0.220465116279102, 0.6438759689922159, 2.2427131782945415, -0.43170542635662124, -2.1448837209302645, -2.598372093023288, -3.8386821705426684, -3.350310077519412, -1.1584496124031332, -1.6061240310077842, -1.3289922480620477, 0.008217054263533807, -1.5712403100775514, 0.023720930232526083, 0.8512403100774873, 0.22914728682167337, -2.9665891472868537, -3.466589147286854, -3.1506976744186366, -2.9413953488372417, 0.025658914728649895, 1.267906976744154, 1.459767441860433, 1.632248062015472, 3.6710077519379523, 0.23883720930229324, -1.0828682170542958, -1.3755038759690246, -2.84449612403104, -3.9258914728682495, -3.3173643410853035, -4.697209302325613, -5.747596899224838, -3.1100000000000323, -4.947209302325614, -5.158449612403133, -3.904573643410885, -3.9937209302325902, -3.2921705426356906, -2.2824806201550714, -0.5460465116279392, 1.8551162790697353, 2.8008527131782626, 3.3144186046511304, -0.5441085271318151, -4.947209302325613, -4.827054263565923, -5.055736434108558, -1.3289922480620477, -0.4006976744186368, 0.05860465116275851, 2.2892248062015184, -1.9762790697674741, -3.237906976744218, -5.3716279069767765, -6.985968992248094, -4.032480620155071, -1.476279069767474, 0.13224806201547173, -0.49178294573646625, -2.5499224806201872, -2.08480620155042, -4.009224806201583, -6.125503875969025, -6.538294573643443, -6.896821705426389, -6.6235658914729, -4.778604651162823, -1.782480620155071, -0.6313178294573967, 0.31248062015500655, 0.43651162790694464, -1.6196899224806522, -4.4762790697674735, -3.4762790697674744, -5.20496124031011, -4.654573643410885, -2.6855813953488696, -4.265038759689954, -0.8638759689922804, 0.03534883720927029, -1.340620155038792, 0.6613178294573321, -2.5693023255814276, -1.2689147286822027, 1.6962015503875647, 0.6729457364340763, 0.589612403100743, -1.4162015503876288, -4.111937984496157, -4.2049612403101095, -1.0014728682170866, 0.5566666666666344, 1.6089922480619834, 1.085736434108495, -2.0576744186046834, -1.9297674418604973, -1.561550387596931, -0.18945736434111754, 0.6690697674418283, 0.7601550387596578, -1.4123255813953808, -0.06155038759693121, -4.780542635658946, -3.598372093023287, 0.7097674418604338, -0.11968992248065169, 6.5741085271317505, 4.203953488372061, 1.878372093023224, 0.8977519379844642, 0.9132558139534561, 1.2950387596898902, 1.5159689922480297, 1.6303100775193475, 0.36286821705423145, -1.8851937984496447, -1.6158139534884044, -0.8328682170542958, -1.7669767441860789, 0.9151937984495802, -3.21465116279073, -6.131317829457396, -5.850310077519412, -6.885193798449644, -5.046046511627939, -5.8251162790698, -5.466589147286854, -3.644883720930265, -3.7844186046511945, -3.6623255813953812, -3.947209302325614, -4.598372093023288, -4.423953488372126, -2.6119379844961563, -0.3890697674418928, -0.04604651162793927, 0.008217054263533585, -0.22046511627910204, -2.852248062015536, -3.476279069767474, -2.0131007751938306, -1.805736434108559, 0.9035658914728362, -1.1448837209302645, -1.1642635658915048, 1.3744961240309757, -3.2960465116279387, -2.179767441860497, -3.36387596899228, -4.931705426356621, -2.1390697674418924, -0.12356589147290031, 2.9849612403100454, 2.9500775193798123, 3.3493023255813634, 1.8919379844960915, -2.040232558139567, -1.8348062015504198, 0.48883720930229346, 0.7465891472867897, 3.7058914728681853, 3.0334108527131463, 0.20782945736430886, -0.8968217054263887, -4.673953488372126, -4.772790697674451, -5.3968217054263885, -5.945271317829489, -3.226279069767474, -2.524728682170575, -3.487906976744218, -4.4510852713178615, -4.115813953488404, -4.5964341085271645, -3.3212403100775516, -0.5266666666666988, -2.3832558139535207, -2.034418604651195, 0.5469767441860145, 0.4171317829457044, 1.576046511627875, 1.566356589147255, 1.5043410852712857, -1.1933333333333658, -3.1836434108527456, -2.5499224806201872, -6.443333333333365, -4.555736434108559, -3.0227906976744503, -1.3037984496124349, -0.9917829457364662, -1.0964341085271636, -0.25147286821708636, -3.1468217054263885, -2.790232558139567, -2.1177519379845284, -2.1642635658915053, -3.040232558139567, -2.5615503875969314, 0.4655813953488046, -0.9840310077519705, 0.20007751937981255, 0.5760465116278746, -3.206899224806234, -0.6836434108527454, -0.6526356589147609, -1.4937209302325902, -0.4394573643411175, -0.9530232558139858, -1.6235658914729005, 0.17294573643407635, -1.912325581395381, -4.927829457364373, -3.7204651162791023, -7.092558139534916, -5.974341085271351, -4.080930232558172, -3.817364341085304, -0.2824806201550709, -3.710775193798482, -3.0441085271318156, -1.761162790697707, -3.2320930232558465, 1.967519379844929, 1.3124806201550065, -0.10418604651166005, 2.2562790697674098, 0.6283720930232237, 4.03534883720927, 1.159379844961208, 0.4365116279069442, -0.2282170542635984, -3.809612403100808, 1.1748837209302, 0.36286821705423106, -1.2049612403101102, -0.15457364341088498, -4.137131782945769, -3.1623255813953812, -1.6972093023256138, -1.4975968992248387, 2.8163565891472544, -1.036356589147319, 0.6380620155038437, 0.058604651162758564, -0.5014728682170864, 0.36674418604647974, 1.5508527131782626, 1.4888372093022935, -0.8910077519380166, 1.8899999999999677, 0.6128682170542313, 2.583798449612371, 2.409379844961208, 2.1438759689922158, 0.056666666666634447, -1.3580620155039083, -0.17007751937987714, -2.526666666666699, -0.8890697674418926, -0.3716279069767763, -1.4975968992248385, -0.06542635658917956]
  out "CH 2 Bin Readings":dbl[](array[numeric])=[4534.0, 4468.0, 4463.0, 4418.0, 4437.0, 4640.0, 4605.0, 4432.0, 4509.0, 4491.0, 4549.0, 4583.0, 4499.0, 4529.0, 4444.0, 4490.0, 4495.0, 4551.0, 4556.0, 4422.0, 4457.0, 4536.0, 4508.0, 4472.0, 4722.0, 4501.0, 4568.0, 4488.0, 4527.0, 4643.0, 4539.0, 4545.0, 4488.0, 4571.0, 4640.0, 4556.0, 4523.0, 4591.0, 4509.0, 4558.0, 4495.0, 4531.0, 4614.0, 4493.0, 4569.0, 4603.0, 4572.0, 4515.0, 4552.0, 4469.0, 4601.0, 4547.0, 4618.0, 4527.0, 4517.0, 4610.0, 4580.0, 4555.0, 4588.0, 4632.0, 4658.0, 4661.0, 4718.0, 4829.0, 4668.0, 4785.0, 4866.0, 4888.0, 5018.0, 4908.0, 5068.0, 5223.0, 5077.0, 4999.0, 4907.0, 5061.0, 5025.0, 4982.0, 4677.0, 4738.0, 4653.0, 4599.0, 4576.0, 4615.0, 4616.0, 4776.0, 4933.0, 5167.0, 5263.0, 5323.0, 5030.0, 5019.0, 4996.0, 4959.0, 4849.0, 4699.0, 4628.0, 4655.0, 4547.0, 4473.0, 4488.0, 4559.0, 4621.0, 4423.0, 4421.0, 4442.0, 4466.0, 4520.0, 4399.0, 4378.0, 4592.0, 4525.0, 4547.0, 4476.0, 4519.0, 4411.0, 4502.0, 4536.0, 4527.0, 4464.0, 4493.0, 4402.0, 4598.0, 4538.0, 4490.0, 4449.0, 4371.0, 4479.0, 4471.0, 4443.0, 4615.0, 4578.0, 4545.0, 4461.0, 4371.0, 4481.0, 4487.0, 4476.0, 4525.0, 4582.0, 4463.0, 4599.0, 4458.0, 4641.0, 4444.0, 4613.0, 4469.0, 4545.0, 4386.0, 4430.0, 4359.0, 4551.0, 4559.0, 4415.0, 4520.0, 4467.0, 4417.0, 4452.0, 4546.0, 4531.0, 4559.0, 4378.0, 4528.0, 4457.0, 4584.0, 4538.0, 4445.0, 4464.0, 4441.0, 4401.0, 4519.0, 4567.0, 4570.0, 4497.0, 4448.0, 4537.0, 4341.0, 4542.0, 4469.0, 4549.0, 4386.0, 4552.0, 4507.0, 4489.0, 4490.0, 4478.0, 4442.0, 4400.0, 4622.0, 4461.0, 4530.0, 4437.0, 4452.0, 4473.0, 4502.0, 4614.0, 4606.0, 4493.0, 4528.0, 4538.0, 4560.0, 4399.0, 4434.0, 4527.0, 4458.0, 4410.0, 4384.0, 4524.0, 4350.0, 4645.0, 4487.0, 4492.0, 4439.0, 4471.0, 4598.0, 4587.0, 4622.0, 4459.0, 4528.0, 4465.0, 4448.0, 4447.0, 4450.0, 4401.0, 4449.0, 4522.0, 4380.0, 4541.0, 4515.0, 4479.0, 4509.0, 4531.0, 4468.0, 4459.0, 4464.0, 4574.0, 4548.0, 4584.0, 4504.0, 4454.0, 4465.0, 4486.0, 4448.0, 4457.0, 4539.0, 4416.0, 4533.0, 4496.0, 4527.0, 4457.0, 4543.0, 4469.0, 4560.0, 4525.0, 4509.0, 4495.0, 4525.0, 4384.0, 4470.0, 4560.0, 4504.0, 4461.0, 4608.0, 4464.0, 4486.0, 4539.0, 4519.0, 4400.0, 4434.0, 4429.0, 4656.0, 4434.0, 4481.0, 4515.0, 4577.0, 4450.0, 4470.0, 4355.0, 4453.0, 4361.0, 4434.0, 4517.0, 4566.0, 4395.0, 4572.0, 4556.0, 4418.0, 4426.0, 4487.0, 4476.0, 4412.0, 4588.0, 4334.0, 4421.0, 4492.0, 4609.0, 4520.0, 4400.0, 4489.0, 4478.0, 4432.0, 4407.0, 4381.0, 4528.0, 4564.0, 4416.0, 4438.0, 4481.0, 4436.0, 4381.0, 4361.0, 4411.0, 4492.0, 4473.0, 4535.0, 4411.0, 4516.0, 4505.0, 4433.0, 4483.0, 4436.0, 4494.0, 4442.0, 4496.0, 4432.0, 4417.0, 4420.0, 4459.0, 4423.0, 4574.0, 4498.0, 4502.0, 4379.0, 4514.0, 4597.0, 4447.0, 4411.0, 4538.0, 4545.0, 4528.0, 4513.0, 4434.0, 4559.0, 4513.0, 4389.0, 4527.0, 4496.0, 4410.0, 4513.0, 4532.0, 4405.0, 4466.0, 4439.0, 4349.0, 4528.0, 4463.0, 4454.0, 4401.0, 4523.0, 4612.0, 4488.0, 4468.0, 4612.0, 4537.0, 4427.0, 4518.0, 4496.0, 4376.0, 4481.0, 4546.0, 4373.0, 4362.0, 4474.0, 4451.0, 4429.0, 4452.0, 4591.0, 4510.0, 4526.0, 4471.0, 4513.0, 4489.0, 4450.0, 4424.0, 4513.0, 4523.0, 4372.0, 4550.0, 4528.0, 4562.0, 4480.0, 4382.0, 4523.0, 4542.0, 4553.0, 4515.0, 4521.0, 4625.0, 4517.0, 4462.0, 4623.0, 4514.0, 4597.0, 4464.0, 4493.0, 4431.0, 4529.0, 4447.0, 4437.0, 4661.0, 4493.0, 4497.0, 4521.0, 4456.0, 4500.0, 4398.0, 4566.0, 4396.0, 4488.0, 4528.0, 4575.0, 4560.0, 4434.0, 4398.0, 4522.0, 4453.0, 4519.0, 4427.0, 4447.0, 4542.0, 4528.0, 4423.0, 4557.0, 4535.0, 4560.0, 4497.0, 4441.0, 4454.0, 4526.0, 4482.0, 4454.0, 4438.0, 4537.0, 4532.0, 4497.0, 4508.0, 4552.0, 4560.0, 4591.0, 4351.0, 4491.0, 4477.0, 4567.0, 4464.0, 4478.0, 4473.0, 4480.0, 4462.0, 4524.0, 4556.0, 4431.0, 4532.0, 4361.0, 4494.0, 4535.0, 4388.0, 4531.0, 4445.0, 4381.0, 4544.0, 4475.0, 4663.0, 4497.0, 4502.0, 4472.0, 4528.0, 4569.0, 4575.0, 4519.0, 4443.0, 4531.0, 4615.0, 4434.0, 4479.0, 4556.0, 4436.0, 4536.0, 4541.0, 4552.0, 4351.0, 4600.0, 4539.0, 4483.0, 4632.0, 4519.0, 4559.0, 4372.0, 4519.0, 4465.0, 4534.0, 4478.0, 4467.0, 4394.0, 4453.0, 4488.0, 4569.0, 4482.0, 4478.0, 4580.0, 4484.0, 4473.0, 4381.0, 4439.0, 4444.0, 4437.0, 4485.0, 4471.0, 4473.0, 4456.0, 4628.0, 4449.0, 4400.0, 4437.0, 4519.0, 4489.0, 4606.0, 4396.0, 4596.0, 4500.0, 4518.0, 4472.0, 4571.0, 4569.0, 4391.0, 4549.0, 4353.0, 4490.0, 4520.0, 4569.0, 4495.0, 4547.0, 4533.0, 4514.0, 4557.0, 4482.0, 4533.0, 4421.0, 4478.0, 4610.0, 4430.0, 4522.0, 4415.0, 4474.0, 4396.0, 4366.0, 4578.0, 4494.0, 4463.0, 4519.0]
  in  "stop":bool
  in  "Reset Average":bool=TRUE
  in  "Save Data?":bool=TRUE
  in  "Collect Data?":bool=TRUE
  in  "ILX Address":i32=6 min=0 step=1
  in  "Lambda On DBR Current":dbl=171.13999999999868
  in  "Lambda Off DBR Current":dbl=172.9499999999997
  in  "Tab Control":T2(tab)=enum."NRB"
  out "NRB plot":cluster{"Y":dbl[], "Y":dbl[]}[](graph)=[{"Y"=[], "Y"=[0.0375, 0.075, 0.11249999999999999, 0.15, 0.1875, 0.225, 0.26249999999999996, 0.3, 0.33749999999999997, 0.37499999999999994, 0.4125, 0.44999999999999996, 0.48749999999999993, 0.525, 0.5625, 0.6, 0.6375, 0.6749999999999999, 0.7124999999999999, 0.75, 0.7875, 0.825, 0.8624999999999999, 0.8999999999999999, 0.9374999999999999, 0.975, 1.0125, 1.05, 1.0875000000000001, 1.125, 1.1625, 1.2, 1.2375, 1.2750000000000001, 1.3125, 1.35, 1.3875, 1.425, 1.4625000000000001, 1.5, 1.5375, 1.575, 1.6125, 1.6500000000000001, 1.6875, 1.725, 1.7625, 1.8, 1.8375, 1.875, 1.9125, 1.95, 1.9875, 2.025, 2.0625, 2.1, 2.1375, 2.175, 2.2125, 2.25, 2.2875, 2.325, 2.3625, 2.4, 2.4375, 2.475, 2.5125, 2.55, 2.5875, 2.625, 2.6625, 2.7, 2.7375, 2.775, 2.8125, 2.85, 2.8875, 2.925, 2.9625, 3.0, 3.0375, 3.075, 3.1125, 3.15, 3.1875, 3.225, 3.2625, 3.3, 3.3375, 3.375, 3.4125, 3.45, 3.4875, 3.525, 3.5625, 3.6, 3.6374999999999997, 3.675, 3.7125, 3.75, 3.7875, 3.8249999999999997, 3.8625, 3.9, 3.9375, 3.975, 4.012499999999999, 4.05, 4.0874999999999995, 4.124999999999999, 4.1625, 4.199999999999999, 4.2375, 4.2749999999999995, 4.312499999999999, 4.35, 4.387499999999999, 4.425, 4.4624999999999995, 4.499999999999999, 4.5375, 4.574999999999999, 4.6125, 4.6499999999999995, 4.687499999999999, 4.725, 4.762499999999999, 4.8, 4.8374999999999995, 4.874999999999999, 4.9125, 4.949999999999999, 4.9875, 5.0249999999999995, 5.062499999999999, 5.1, 5.137499999999999, 5.175, 5.2124999999999995, 5.249999999999999, 5.2875, 5.324999999999999, 5.3625, 5.3999999999999995, 5.437499999999999, 5.475, 5.512499999999999, 5.55, 5.5874999999999995, 5.624999999999999, 5.6625, 5.699999999999999, 5.7375, 5.7749999999999995, 5.812499999999999, 5.85, 5.887499999999999, 5.925, 5.9624999999999995, 5.999999999999999, 6.0375, 6.074999999999999, 6.1125, 6.1499999999999995, 6.187499999999999, 6.225, 6.262499999999999, 6.3, 6.3374999999999995, 6.374999999999999, 6.4125, 6.449999999999999, 6.4875, 6.5249999999999995, 6.562499999999999, 6.6, 6.637499999999999, 6.675, 6.7124999999999995, 6.749999999999999, 6.7875, 6.824999999999999, 6.8625, 6.8999999999999995, 6.937499999999999, 6.975, 7.012499999999999, 7.05, 7.0874999999999995, 7.124999999999999, 7.1625, 7.199999999999999, 7.237499999999999, 7.2749999999999995, 7.312499999999999, 7.35, 7.387499999999999, 7.424999999999999, 7.4624999999999995, 7.499999999999999, 7.5375, 7.574999999999999, 7.612499999999999, 7.6499999999999995, 7.687499999999999, 7.725, 7.762499999999999, 7.799999999999999, 7.8374999999999995, 7.874999999999999, 7.9125, 7.949999999999999, 7.987499999999999, 8.025, 8.0625, 8.1, 8.1375, 8.174999999999999, 8.212499999999999, 8.25, 8.2875, 8.325, 8.362499999999999, 8.399999999999999, 8.4375, 8.475, 8.5125, 8.549999999999999, 8.587499999999999, 8.625, 8.6625, 8.7, 8.737499999999999, 8.774999999999999, 8.8125, 8.85, 8.8875, 8.924999999999999, 8.962499999999999, 9.0, 9.0375, 9.075, 9.112499999999999, 9.149999999999999, 9.1875, 9.225, 9.2625, 9.299999999999999, 9.337499999999999, 9.375, 9.4125, 9.45, 9.487499999999999, 9.524999999999999, 9.5625, 9.6, 9.6375, 9.674999999999999, 9.712499999999999, 9.75, 9.7875, 9.825, 9.862499999999999, 9.899999999999999, 9.9375, 9.975, 10.0125, 10.049999999999999, 10.087499999999999, 10.125, 10.1625, 10.2, 10.237499999999999, 10.274999999999999, 10.3125, 10.35, 10.3875, 10.424999999999999, 10.462499999999999, 10.5, 10.5375, 10.575, 10.612499999999999, 10.649999999999999, 10.6875, 10.725, 10.7625, 10.799999999999999, 10.837499999999999, 10.875, 10.9125, 10.95, 10.987499999999999, 11.024999999999999, 11.0625, 11.1, 11.1375, 11.174999999999999, 11.212499999999999, 11.25, 11.2875, 11.325, 11.362499999999999, 11.399999999999999, 11.4375, 11.475, 11.5125, 11.549999999999999, 11.587499999999999, 11.625, 11.6625, 11.7, 11.737499999999999, 11.774999999999999, 11.8125, 11.85, 11.8875, 11.924999999999999, 11.962499999999999, 12.0, 12.0375, 12.075, 12.112499999999999, 12.149999999999999, 12.1875, 12.225, 12.2625, 12.299999999999999, 12.337499999999999, 12.375, 12.4125, 12.45, 12.487499999999999, 12.524999999999999, 12.5625, 12.6, 12.6375, 12.674999999999999, 12.712499999999999, 12.75, 12.7875, 12.825, 12.862499999999999, 12.899999999999999, 12.9375, 12.975, 13.0125, 13.049999999999999, 13.087499999999999, 13.125, 13.1625, 13.2, 13.237499999999999, 13.274999999999999, 13.3125, 13.35, 13.3875, 13.424999999999999, 13.462499999999999, 13.5, 13.5375, 13.575, 13.612499999999999, 13.649999999999999, 13.6875, 13.725, 13.7625, 13.799999999999999, 13.837499999999999, 13.875, 13.9125, 13.95, 13.987499999999999, 14.024999999999999, 14.0625, 14.1, 14.1375, 14.174999999999999, 14.212499999999999, 14.25, 14.2875, 14.325, 14.362499999999999, 14.399999999999999, 14.437499999999998, 14.475, 14.5125, 14.549999999999999, 14.587499999999999, 14.624999999999998, 14.6625, 14.7, 14.737499999999999, 14.774999999999999, 14.812499999999998, 14.85, 14.8875, 14.924999999999999, 14.962499999999999, 14.999999999999998, 15.0375, 15.075, 15.112499999999999, 15.149999999999999, 15.187499999999998, 15.225, 15.2625, 15.299999999999999, 15.337499999999999, 15.374999999999998, 15.4125, 15.45, 15.487499999999999, 15.524999999999999, 15.562499999999998, 15.6, 15.6375, 15.674999999999999, 15.712499999999999, 15.749999999999998, 15.7875, 15.825, 15.862499999999999, 15.899999999999999, 15.937499999999998, 15.975, 16.0125, 16.05, 16.087500000000002, 16.125, 16.1625, 16.2, 16.2375, 16.275000000000002, 16.3125, 16.35, 16.3875, 16.425, 16.462500000000002, 16.5, 16.5375, 16.575, 16.6125, 16.650000000000002, 16.6875, 16.725, 16.7625, 16.8, 16.837500000000002, 16.875, 16.9125, 16.95, 16.9875, 17.025000000000002, 17.0625, 17.1, 17.1375, 17.175, 17.212500000000002, 17.25, 17.2875, 17.325, 17.3625, 17.400000000000002, 17.4375, 17.475, 17.5125, 17.55, 17.587500000000002, 17.625, 17.6625, 17.7, 17.7375, 17.775000000000002, 17.8125, 17.85, 17.8875, 17.925, 17.962500000000002, 18.0, 18.0375, 18.075, 18.1125, 18.150000000000002, 18.1875, 18.225, 18.2625, 18.3, 18.337500000000002, 18.375, 18.4125, 18.45, 18.4875, 18.525000000000002, 18.5625, 18.6, 18.6375, 18.675, 18.712500000000002, 18.75, 18.7875, 18.825, 18.8625, 18.900000000000002, 18.9375, 18.975, 19.0125, 19.05, 19.087500000000002, 19.125, 19.1625, 19.2, 19.2375, 19.275000000000002, 19.3125, 19.35, 19.3875, 19.425, 19.462500000000002, 19.5, 19.5375, 19.575, 19.6125, 19.650000000000002, 19.6875, 19.725, 19.7625, 19.8, 19.837500000000002, 19.875, 19.9125, 19.95, 19.9875, 20.025000000000002, 20.0625, 20.1, 20.1375, 20.175, 20.212500000000002, 20.25, 20.2875, 20.325, 20.3625, 20.400000000000002, 20.4375, 20.475, 20.5125, 20.55, 20.587500000000002, 20.625, 20.6625, 20.7, 20.7375, 20.775000000000002, 20.8125, 20.85, 20.8875, 20.925, 20.962500000000002, 21.0]}, ...(2 in all)]
  in  "background length":i32=25
  out "Correction":cluster{"Y":dbl[], "Y":dbl[]}[](graph)=[{"Y"=[], "Y"=[0.0375, 0.075, 0.11249999999999999, 0.15, 0.1875, 0.225, 0.26249999999999996, 0.3, 0.33749999999999997, 0.37499999999999994, 0.4125, 0.44999999999999996, 0.48749999999999993, 0.525, 0.5625, 0.6, 0.6375, 0.6749999999999999, 0.7124999999999999, 0.75, 0.7875, 0.825, 0.8624999999999999, 0.8999999999999999, 0.9374999999999999, 0.975, 1.0125, 1.05, 1.0875000000000001, 1.125, 1.1625, 1.2, 1.2375, 1.2750000000000001, 1.3125, 1.35, 1.3875, 1.425, 1.4625000000000001, 1.5, 1.5375, 1.575, 1.6125, 1.6500000000000001, 1.6875, 1.725, 1.7625, 1.8, 1.8375, 1.875, 1.9125, 1.95, 1.9875, 2.025, 2.0625, 2.1, 2.1375, 2.175, 2.2125, 2.25, 2.2875, 2.325, 2.3625, 2.4, 2.4375, 2.475, 2.5125, 2.55, 2.5875, 2.625, 2.6625, 2.7, 2.7375, 2.775, 2.8125, 2.85, 2.8875, 2.925, 2.9625, 3.0, 3.0375, 3.075, 3.1125, 3.15, 3.1875, 3.225, 3.2625, 3.3, 3.3375, 3.375, 3.4125, 3.45, 3.4875, 3.525, 3.5625, 3.6, 3.6374999999999997, 3.675, 3.7125, 3.75, 3.7875, 3.8249999999999997, 3.8625, 3.9, 3.9375, 3.975, 4.012499999999999, 4.05, 4.0874999999999995, 4.124999999999999, 4.1625, 4.199999999999999, 4.2375, 4.2749999999999995, 4.312499999999999, 4.35, 4.387499999999999, 4.425, 4.4624999999999995, 4.499999999999999, 4.5375, 4.574999999999999, 4.6125, 4.6499999999999995, 4.687499999999999, 4.725, 4.762499999999999, 4.8, 4.8374999999999995, 4.874999999999999, 4.9125, 4.949999999999999, 4.9875, 5.0249999999999995, 5.062499999999999, 5.1, 5.137499999999999, 5.175, 5.2124999999999995, 5.249999999999999, 5.2875, 5.324999999999999, 5.3625, 5.3999999999999995, 5.437499999999999, 5.475, 5.512499999999999, 5.55, 5.5874999999999995, 5.624999999999999, 5.6625, 5.699999999999999, 5.7375, 5.7749999999999995, 5.812499999999999, 5.85, 5.887499999999999, 5.925, 5.9624999999999995, 5.999999999999999, 6.0375, 6.074999999999999, 6.1125, 6.1499999999999995, 6.187499999999999, 6.225, 6.262499999999999, 6.3, 6.3374999999999995, 6.374999999999999, 6.4125, 6.449999999999999, 6.4875, 6.5249999999999995, 6.562499999999999, 6.6, 6.637499999999999, 6.675, 6.7124999999999995, 6.749999999999999, 6.7875, 6.824999999999999, 6.8625, 6.8999999999999995, 6.937499999999999, 6.975, 7.012499999999999, 7.05, 7.0874999999999995, 7.124999999999999, 7.1625, 7.199999999999999, 7.237499999999999, 7.2749999999999995, 7.312499999999999, 7.35, 7.387499999999999, 7.424999999999999, 7.4624999999999995, 7.499999999999999, 7.5375, 7.574999999999999, 7.612499999999999, 7.6499999999999995, 7.687499999999999, 7.725, 7.762499999999999, 7.799999999999999, 7.8374999999999995, 7.874999999999999, 7.9125, 7.949999999999999, 7.987499999999999, 8.025, 8.0625, 8.1, 8.1375, 8.174999999999999, 8.212499999999999, 8.25, 8.2875, 8.325, 8.362499999999999, 8.399999999999999, 8.4375, 8.475, 8.5125, 8.549999999999999, 8.587499999999999, 8.625, 8.6625, 8.7, 8.737499999999999, 8.774999999999999, 8.8125, 8.85, 8.8875, 8.924999999999999, 8.962499999999999, 9.0, 9.0375, 9.075, 9.112499999999999, 9.149999999999999, 9.1875, 9.225, 9.2625, 9.299999999999999, 9.337499999999999, 9.375, 9.4125, 9.45, 9.487499999999999, 9.524999999999999, 9.5625, 9.6, 9.6375, 9.674999999999999, 9.712499999999999, 9.75, 9.7875, 9.825, 9.862499999999999, 9.899999999999999, 9.9375, 9.975, 10.0125, 10.049999999999999, 10.087499999999999, 10.125, 10.1625, 10.2, 10.237499999999999, 10.274999999999999, 10.3125, 10.35, 10.3875, 10.424999999999999, 10.462499999999999, 10.5, 10.5375, 10.575, 10.612499999999999, 10.649999999999999, 10.6875, 10.725, 10.7625, 10.799999999999999, 10.837499999999999, 10.875, 10.9125, 10.95, 10.987499999999999, 11.024999999999999, 11.0625, 11.1, 11.1375, 11.174999999999999, 11.212499999999999, 11.25, 11.2875, 11.325, 11.362499999999999, 11.399999999999999, 11.4375, 11.475, 11.5125, 11.549999999999999, 11.587499999999999, 11.625, 11.6625, 11.7, 11.737499999999999, 11.774999999999999, 11.8125, 11.85, 11.8875, 11.924999999999999, 11.962499999999999, 12.0, 12.0375, 12.075, 12.112499999999999, 12.149999999999999, 12.1875, 12.225, 12.2625, 12.299999999999999, 12.337499999999999, 12.375, 12.4125, 12.45, 12.487499999999999, 12.524999999999999, 12.5625, 12.6, 12.6375, 12.674999999999999, 12.712499999999999, 12.75, 12.7875, 12.825, 12.862499999999999, 12.899999999999999, 12.9375, 12.975, 13.0125, 13.049999999999999, 13.087499999999999, 13.125, 13.1625, 13.2, 13.237499999999999, 13.274999999999999, 13.3125, 13.35, 13.3875, 13.424999999999999, 13.462499999999999, 13.5, 13.5375, 13.575, 13.612499999999999, 13.649999999999999, 13.6875, 13.725, 13.7625, 13.799999999999999, 13.837499999999999, 13.875, 13.9125, 13.95, 13.987499999999999, 14.024999999999999, 14.0625, 14.1, 14.1375, 14.174999999999999, 14.212499999999999, 14.25, 14.2875, 14.325, 14.362499999999999, 14.399999999999999, 14.437499999999998, 14.475, 14.5125, 14.549999999999999, 14.587499999999999, 14.624999999999998, 14.6625, 14.7, 14.737499999999999, 14.774999999999999, 14.812499999999998, 14.85, 14.8875, 14.924999999999999, 14.962499999999999, 14.999999999999998, 15.0375, 15.075, 15.112499999999999, 15.149999999999999, 15.187499999999998, 15.225, 15.2625, 15.299999999999999, 15.337499999999999, 15.374999999999998, 15.4125, 15.45, 15.487499999999999, 15.524999999999999, 15.562499999999998, 15.6, 15.6375, 15.674999999999999, 15.712499999999999, 15.749999999999998, 15.7875, 15.825, 15.862499999999999, 15.899999999999999, 15.937499999999998, 15.975, 16.0125, 16.05, 16.087500000000002, 16.125, 16.1625, 16.2, 16.2375, 16.275000000000002, 16.3125, 16.35, 16.3875, 16.425, 16.462500000000002, 16.5, 16.5375, 16.575, 16.6125, 16.650000000000002, 16.6875, 16.725, 16.7625, 16.8, 16.837500000000002, 16.875, 16.9125, 16.95, 16.9875, 17.025000000000002, 17.0625, 17.1, 17.1375, 17.175, 17.212500000000002, 17.25, 17.2875, 17.325, 17.3625, 17.400000000000002, 17.4375, 17.475, 17.5125, 17.55, 17.587500000000002, 17.625, 17.6625, 17.7, 17.7375, 17.775000000000002, 17.8125, 17.85, 17.8875, 17.925, 17.962500000000002, 18.0, 18.0375, 18.075, 18.1125, 18.150000000000002, 18.1875, 18.225, 18.2625, 18.3, 18.337500000000002, 18.375, 18.4125, 18.45, 18.4875, 18.525000000000002, 18.5625, 18.6, 18.6375, 18.675, 18.712500000000002, 18.75, 18.7875, 18.825, 18.8625, 18.900000000000002, 18.9375, 18.975, 19.0125, 19.05, 19.087500000000002, 19.125, 19.1625, 19.2, 19.2375, 19.275000000000002, 19.3125, 19.35, 19.3875, 19.425, 19.462500000000002, 19.5, 19.5375, 19.575, 19.6125, 19.650000000000002, 19.6875, 19.725, 19.7625, 19.8, 19.837500000000002, 19.875, 19.9125, 19.95, 19.9875, 20.025000000000002, 20.0625, 20.1, 20.1375, 20.175, 20.212500000000002, 20.25, 20.2875, 20.325, 20.3625, 20.400000000000002, 20.4375, 20.475, 20.5125, 20.55, 20.587500000000002, 20.625, 20.6625, 20.7, 20.7375, 20.775000000000002, 20.8125, 20.85, 20.8875, 20.925, 20.962500000000002, 21.0]}, ...(2 in all)]
  in  "dead time":dbl=3.7e-08
  out "CH1 RingBuffer long":dbl[][](array[numeric])
  out "CH1 RingBuffer short":dbl[][](array[numeric])
  in  "Weather":T3(tab)=enum."Background (Mc/s)"
  out "Temperature (C)":dbl(graph)=7.387362637362642
  out "Pressure (mb)":dbl(graph)=842.0054945054944
  out "Relative Humdity (%)":dbl(graph)=61.460622710622715
  out "Pulse Energy (Micro Joule)":T4(graph)
  out "?":cluster{"mean":dbl, "mean":dbl}(graph)={"mean"=0.0, "mean"=522259.7129856493}
  out "Index":i32=27489
  out "CH1 (WV off) smooth L":dbl[](array[numeric])
  out "CH1  Bin Readings":dbl[](array[numeric])
  out "CH1 (WV off) smooth S":dbl[](array[numeric])
  out "CH0 (WV on) smoothed":dbl[](array[numeric])
  out "CH 0 Bin Readings":dbl[](array[numeric])
  out "Range Corrected Altitude Array":dbl[](array[numeric])=[1406.25, 5625.0, 12656.25, 22500.0, 35156.25, 50625.0, 68906.25, 90000.0, 113906.25, 140625.0, 170156.25, 202500.0, 237656.25, 275625.0, 316406.25, 360000.0, 406406.25, 455625.0, 507656.25, 562500.0, 620156.25, 680625.0, 743906.25, 810000.0, 878906.25, 950625.0, 1025156.25, 1102500.0, 1182656.25, 1265625.0, 1351406.25, 1440000.0, 1531406.25, 1625625.0, 1722656.25, 1822500.0, 1925156.25, 2030625.0, 2138906.25, 2250000.0, 2363906.25, 2480625.0, 2600156.25, 2722500.0, 2847656.25, 2975625.0, 3106406.25, 3240000.0, 3376406.25, 3515625.0, 3657656.25, 3802500.0, 3950156.25, 4100625.0, 4253906.25, 4410000.0, 4568906.25, 4730625.0, 4895156.25, 5062500.0, 5232656.25, 5405625.0, 5581406.25, 5760000.0, 5941406.25, 6125625.0, 6312656.25, 6502500.0, 6695156.25, 6890625.0, 7088906.25, 7290000.0, 7493906.25, 7700625.0, 7910156.25, 8122500.0, 8337656.25, 8555625.0, 8776406.25, 9000000.0, 9226406.25, 9455625.0, 9687656.25, 9922500.0, 10160156.25, 10400625.0, 10643906.25, 10890000.0, 11138906.25, 11390625.0, 11645156.25, 11902500.0, 12162656.25, 12425625.0, 12691406.25, 12960000.0, 13231406.25, 13505625.0, 13782656.25, 14062500.0, 14345156.25, 14630625.0, 14918906.25, 15210000.0, 15503906.25, 15800625.0, 16100156.25, 16402500.0, 16707656.25, 17015625.0, 17326406.25, 17640000.0, 17956406.25, 18275625.0, 18597656.25, 18922500.0, 19250156.25, 19580625.0, 19913906.25, 20250000.0, 20588906.25, 20930625.0, 21275156.25, 21622500.0, 21972656.25, 22325625.0, 22681406.25, 23040000.0, 23401406.25, 23765625.0, 24132656.25, 24502500.0, 24875156.25, 25250625.0, 25628906.25, 26010000.0, 26393906.25, 26780625.0, 27170156.25, 27562500.0, 27957656.25, 28355625.0, 28756406.25, 29160000.0, 29566406.25, 29975625.0, 30387656.25, 30802500.0, 31220156.25, 31640625.0, 32063906.25, 32490000.0, 32918906.25, 33350625.0, 33785156.25, 34222500.0, 34662656.25, 35105625.0, 35551406.25, 36000000.0, 36451406.25, 36905625.0, 37362656.25, 37822500.0, 38285156.25, 38750625.0, 39218906.25, 39690000.0, 40163906.25, 40640625.0, 41120156.25, 41602500.0, 42087656.25, 42575625.0, 43066406.25, 43560000.0, 44056406.25, 44555625.0, 45057656.25, 45562500.0, 46070156.25, 46580625.0, 47093906.25, 47610000.0, 48128906.25, 48650625.0, 49175156.25, 49702500.0, 50232656.25, 50765625.0, 51301406.25, 51840000.0, 52381406.25, 52925625.0, 53472656.25, 54022500.0, 54575156.25, 55130625.0, 55688906.25, 56250000.0, 56813906.25, 57380625.0, 57950156.25, 58522500.0, 59097656.25, 59675625.0, 60256406.25, 60840000.0, 61426406.25, 62015625.0, 62607656.25, 63202500.0, 63800156.25, 64400625.0, 65003906.25, 65610000.0, 66218906.25, 66830625.0, 67445156.25, 68062500.0, 68682656.25, 69305625.0, 69931406.25, 70560000.0, 71191406.25, 71825625.0, 72462656.25, 73102500.0, 73745156.25, 74390625.0, 75038906.25, 75690000.0, 76343906.25, 77000625.0, 77660156.25, 78322500.0, 78987656.25, 79655625.0, 80326406.25, 81000000.0, 81676406.25, 82355625.0, 83037656.25, 83722500.0, 84410156.25, 85100625.0, 85793906.25, 86490000.0, 87188906.25, 87890625.0, 88595156.25, 89302500.0, 90012656.25, 90725625.0, 91441406.25, 92160000.0, 92881406.25, 93605625.0, 94332656.25, 95062500.0, 95795156.25, 96530625.0, 97268906.25, 98010000.0, 98753906.25, 99500625.0, 100250156.25, 101002500.0, 101757656.25, 102515625.0, 103276406.25, 104040000.0, 104806406.25, 105575625.0, 106347656.25, 107122500.0, 107900156.25, 108680625.0, 109463906.25, 110250000.0, 111038906.25, 111830625.0, 112625156.25, 113422500.0, 114222656.25, 115025625.0, 115831406.25, 116640000.0, 117451406.25, 118265625.0, 119082656.25, 119902500.0, 120725156.25, 121550625.0, 122378906.25, 123210000.0, 124043906.25, 124880625.0, 125720156.25, 126562500.0, 127407656.25, 128255625.0, 129106406.25, 129960000.0, 130816406.25, 131675625.0, 132537656.25, 133402500.0, 134270156.25, 135140625.0, 136013906.25, 136890000.0, 137768906.25, 138650625.0, 139535156.25, 140422500.0, 141312656.25, 142205625.0, 143101406.25, 144000000.0, 144901406.25, 145805625.0, 146712656.25, 147622500.0, 148535156.25, 149450625.0, 150368906.25, 151290000.0, 152213906.25, 153140625.0, 154070156.25, 155002500.0, 155937656.25, 156875625.0, 157816406.25, 158760000.0, 159706406.25, 160655625.0, 161607656.25, 162562500.0, 163520156.25, 164480625.0, 165443906.25, 166410000.0, 167378906.25, 168350625.0, 169325156.25, 170302500.0, 171282656.25, 172265625.0, 173251406.25, 174240000.0, 175231406.25, 176225625.0, 177222656.25, 178222500.0, 179225156.25, 180230625.0, 181238906.25, 182250000.0, 183263906.25, 184280625.0, 185300156.25, 186322500.0, 187347656.25, 188375625.0, 189406406.25, 190440000.0, 191476406.25, 192515625.0, 193557656.25, 194602500.0, 195650156.25, 196700625.0, 197753906.25, 198810000.0, 199868906.25, 200930625.0, 201995156.25, 203062500.0, 204132656.25, 205205625.0, 206281406.25, 207360000.0, 208441406.25, 209525625.0, 210612656.25, 211702500.0, 212795156.25, 213890625.0, 214988906.25, 216090000.0, 217193906.25, 218300625.0, 219410156.25, 220522500.0, 221637656.25, 222755625.0, 223876406.25, 225000000.0, 226126406.25, 227255625.0, 228387656.25, 229522500.0, 230660156.25, 231800625.0, 232943906.25, 234090000.0, 235238906.25, 236390625.0, 237545156.25, 238702500.0, 239862656.25, 241025625.0, 242191406.25, 243360000.0, 244531406.25, 245705625.0, 246882656.25, 248062500.0, 249245156.25, 250430625.0, 251618906.25, 252810000.0, 254003906.25, 255200625.0, 256400156.25, 257602500.0, 258807656.25, 260015625.0, 261226406.25, 262440000.0, 263656406.25, 264875625.0, 266097656.25, 267322500.0, 268550156.25, 269780625.0, 271013906.25, 272250000.0, 273488906.25, 274730625.0, 275975156.25, 277222500.0, 278472656.25, 279725625.0, 280981406.25, 282240000.0, 283501406.25, 284765625.0, 286032656.25, 287302500.0, 288575156.25, 289850625.0, 291128906.25, 292410000.0, 293693906.25, 294980625.0, 296270156.25, 297562500.0, 298857656.25, 300155625.0, 301456406.25, 302760000.0, 304066406.25, 305375625.0, 306687656.25, 308002500.0, 309320156.25, 310640625.0, 311963906.25, 313290000.0, 314618906.25, 315950625.0, 317285156.25, 318622500.0, 319962656.25, 321305625.0, 322651406.25, 324000000.0, 325351406.25, 326705625.0, 328062656.25, 329422500.0, 330785156.25, 332150625.0, 333518906.25, 334890000.0, 336263906.25, 337640625.0, 339020156.25, 340402500.0, 341787656.25, 343175625.0, 344566406.25, 345960000.0, 347356406.25, 348755625.0, 350157656.25, 351562500.0, 352970156.25, 354380625.0, 355793906.25, 357210000.0, 358628906.25, 360050625.0, 361475156.25, 362902500.0, 364332656.25, 365765625.0, 367201406.25, 368640000.0, 370081406.25, 371525625.0, 372972656.25, 374422500.0, 375875156.25, 377330625.0, 378788906.25, 380250000.0, 381713906.25, 383180625.0, 384650156.25, 386122500.0, 387597656.25, 389075625.0, 390556406.25, 392040000.0, 393526406.25, 395015625.0, 396507656.25, 398002500.0, 399500156.25, 401000625.0, 402503906.25, 404010000.0, 405518906.25, 407030625.0, 408545156.25, 410062500.0, 411582656.25, 413105625.0, 414631406.25, 416160000.0, 417691406.25, 419225625.0, 420762656.25, 422302500.0, 423845156.25, 425390625.0, 426938906.25, 428490000.0, 430043906.25, 431600625.0, 433160156.25, 434722500.0, 436287656.25, 437855625.0, 439426406.25, 441000000.0]
  out "Altitude Array (km)":dbl[](array[numeric])=[0.0375, 0.075, 0.11249999999999999, 0.15, 0.1875, 0.225, 0.26249999999999996, 0.3, 0.33749999999999997, 0.37499999999999994, 0.4125, 0.44999999999999996, 0.48749999999999993, 0.525, 0.5625, 0.6, 0.6375, 0.6749999999999999, 0.7124999999999999, 0.75, 0.7875, 0.825, 0.8624999999999999, 0.8999999999999999, 0.9374999999999999, 0.975, 1.0125, 1.05, 1.0875000000000001, 1.125, 1.1625, 1.2, 1.2375, 1.2750000000000001, 1.3125, 1.35, 1.3875, 1.425, 1.4625000000000001, 1.5, 1.5375, 1.575, 1.6125, 1.6500000000000001, 1.6875, 1.725, 1.7625, 1.8, 1.8375, 1.875, 1.9125, 1.95, 1.9875, 2.025, 2.0625, 2.1, 2.1375, 2.175, 2.2125, 2.25, 2.2875, 2.325, 2.3625, 2.4, 2.4375, 2.475, 2.5125, 2.55, 2.5875, 2.625, 2.6625, 2.7, 2.7375, 2.775, 2.8125, 2.85, 2.8875, 2.925, 2.9625, 3.0, 3.0375, 3.075, 3.1125, 3.15, 3.1875, 3.225, 3.2625, 3.3, 3.3375, 3.375, 3.4125, 3.45, 3.4875, 3.525, 3.5625, 3.6, 3.6374999999999997, 3.675, 3.7125, 3.75, 3.7875, 3.8249999999999997, 3.8625, 3.9, 3.9375, 3.975, 4.012499999999999, 4.05, 4.0874999999999995, 4.124999999999999, 4.1625, 4.199999999999999, 4.2375, 4.2749999999999995, 4.312499999999999, 4.35, 4.387499999999999, 4.425, 4.4624999999999995, 4.499999999999999, 4.5375, 4.574999999999999, 4.6125, 4.6499999999999995, 4.687499999999999, 4.725, 4.762499999999999, 4.8, 4.8374999999999995, 4.874999999999999, 4.9125, 4.949999999999999, 4.9875, 5.0249999999999995, 5.062499999999999, 5.1, 5.137499999999999, 5.175, 5.2124999999999995, 5.249999999999999, 5.2875, 5.324999999999999, 5.3625, 5.3999999999999995, 5.437499999999999, 5.475, 5.512499999999999, 5.55, 5.5874999999999995, 5.624999999999999, 5.6625, 5.699999999999999, 5.7375, 5.7749999999999995, 5.812499999999999, 5.85, 5.887499999999999, 5.925, 5.9624999999999995, 5.999999999999999, 6.0375, 6.074999999999999, 6.1125, 6.1499999999999995, 6.187499999999999, 6.225, 6.262499999999999, 6.3, 6.3374999999999995, 6.374999999999999, 6.4125, 6.449999999999999, 6.4875, 6.5249999999999995, 6.562499999999999, 6.6, 6.637499999999999, 6.675, 6.7124999999999995, 6.749999999999999, 6.7875, 6.824999999999999, 6.8625, 6.8999999999999995, 6.937499999999999, 6.975, 7.012499999999999, 7.05, 7.0874999999999995, 7.124999999999999, 7.1625, 7.199999999999999, 7.237499999999999, 7.2749999999999995, 7.312499999999999, 7.35, 7.387499999999999, 7.424999999999999, 7.4624999999999995, 7.499999999999999, 7.5375, 7.574999999999999, 7.612499999999999, 7.6499999999999995, 7.687499999999999, 7.725, 7.762499999999999, 7.799999999999999, 7.8374999999999995, 7.874999999999999, 7.9125, 7.949999999999999, 7.987499999999999, 8.025, 8.0625, 8.1, 8.1375, 8.174999999999999, 8.212499999999999, 8.25, 8.2875, 8.325, 8.362499999999999, 8.399999999999999, 8.4375, 8.475, 8.5125, 8.549999999999999, 8.587499999999999, 8.625, 8.6625, 8.7, 8.737499999999999, 8.774999999999999, 8.8125, 8.85, 8.8875, 8.924999999999999, 8.962499999999999, 9.0, 9.0375, 9.075, 9.112499999999999, 9.149999999999999, 9.1875, 9.225, 9.2625, 9.299999999999999, 9.337499999999999, 9.375, 9.4125, 9.45, 9.487499999999999, 9.524999999999999, 9.5625, 9.6, 9.6375, 9.674999999999999, 9.712499999999999, 9.75, 9.7875, 9.825, 9.862499999999999, 9.899999999999999, 9.9375, 9.975, 10.0125, 10.049999999999999, 10.087499999999999, 10.125, 10.1625, 10.2, 10.237499999999999, 10.274999999999999, 10.3125, 10.35, 10.3875, 10.424999999999999, 10.462499999999999, 10.5, 10.5375, 10.575, 10.612499999999999, 10.649999999999999, 10.6875, 10.725, 10.7625, 10.799999999999999, 10.837499999999999, 10.875, 10.9125, 10.95, 10.987499999999999, 11.024999999999999, 11.0625, 11.1, 11.1375, 11.174999999999999, 11.212499999999999, 11.25, 11.2875, 11.325, 11.362499999999999, 11.399999999999999, 11.4375, 11.475, 11.5125, 11.549999999999999, 11.587499999999999, 11.625, 11.6625, 11.7, 11.737499999999999, 11.774999999999999, 11.8125, 11.85, 11.8875, 11.924999999999999, 11.962499999999999, 12.0, 12.0375, 12.075, 12.112499999999999, 12.149999999999999, 12.1875, 12.225, 12.2625, 12.299999999999999, 12.337499999999999, 12.375, 12.4125, 12.45, 12.487499999999999, 12.524999999999999, 12.5625, 12.6, 12.6375, 12.674999999999999, 12.712499999999999, 12.75, 12.7875, 12.825, 12.862499999999999, 12.899999999999999, 12.9375, 12.975, 13.0125, 13.049999999999999, 13.087499999999999, 13.125, 13.1625, 13.2, 13.237499999999999, 13.274999999999999, 13.3125, 13.35, 13.3875, 13.424999999999999, 13.462499999999999, 13.5, 13.5375, 13.575, 13.612499999999999, 13.649999999999999, 13.6875, 13.725, 13.7625, 13.799999999999999, 13.837499999999999, 13.875, 13.9125, 13.95, 13.987499999999999, 14.024999999999999, 14.0625, 14.1, 14.1375, 14.174999999999999, 14.212499999999999, 14.25, 14.2875, 14.325, 14.362499999999999, 14.399999999999999, 14.437499999999998, 14.475, 14.5125, 14.549999999999999, 14.587499999999999, 14.624999999999998, 14.6625, 14.7, 14.737499999999999, 14.774999999999999, 14.812499999999998, 14.85, 14.8875, 14.924999999999999, 14.962499999999999, 14.999999999999998, 15.0375, 15.075, 15.112499999999999, 15.149999999999999, 15.187499999999998, 15.225, 15.2625, 15.299999999999999, 15.337499999999999, 15.374999999999998, 15.4125, 15.45, 15.487499999999999, 15.524999999999999, 15.562499999999998, 15.6, 15.6375, 15.674999999999999, 15.712499999999999, 15.749999999999998, 15.7875, 15.825, 15.862499999999999, 15.899999999999999, 15.937499999999998, 15.975, 16.0125, 16.05, 16.087500000000002, 16.125, 16.1625, 16.2, 16.2375, 16.275000000000002, 16.3125, 16.35, 16.3875, 16.425, 16.462500000000002, 16.5, 16.5375, 16.575, 16.6125, 16.650000000000002, 16.6875, 16.725, 16.7625, 16.8, 16.837500000000002, 16.875, 16.9125, 16.95, 16.9875, 17.025000000000002, 17.0625, 17.1, 17.1375, 17.175, 17.212500000000002, 17.25, 17.2875, 17.325, 17.3625, 17.400000000000002, 17.4375, 17.475, 17.5125, 17.55, 17.587500000000002, 17.625, 17.6625, 17.7, 17.7375, 17.775000000000002, 17.8125, 17.85, 17.8875, 17.925, 17.962500000000002, 18.0, 18.0375, 18.075, 18.1125, 18.150000000000002, 18.1875, 18.225, 18.2625, 18.3, 18.337500000000002, 18.375, 18.4125, 18.45, 18.4875, 18.525000000000002, 18.5625, 18.6, 18.6375, 18.675, 18.712500000000002, 18.75, 18.7875, 18.825, 18.8625, 18.900000000000002, 18.9375, 18.975, 19.0125, 19.05, 19.087500000000002, 19.125, 19.1625, 19.2, 19.2375, 19.275000000000002, 19.3125, 19.35, 19.3875, 19.425, 19.462500000000002, 19.5, 19.5375, 19.575, 19.6125, 19.650000000000002, 19.6875, 19.725, 19.7625, 19.8, 19.837500000000002, 19.875, 19.9125, 19.95, 19.9875, 20.025000000000002, 20.0625, 20.1, 20.1375, 20.175, 20.212500000000002, 20.25, 20.2875, 20.325, 20.3625, 20.400000000000002, 20.4375, 20.475, 20.5125, 20.55, 20.587500000000002, 20.625, 20.6625, 20.7, 20.7375, 20.775000000000002, 20.8125, 20.85, 20.8875, 20.925, 20.962500000000002, 21.0]
  out "Offline Pulse Energy":dbl
  out "Online Pulse Energy":dbl
  in  "Instrument Control":T5(tab)
  in  "Device In":refnum<visa-resource-name>="Pro8000"
  in  "Settings":T6={"Module"=enum."HSRL TEC", "WV Online TEC"=23.280249999999846, "WV Online LD"=0.17, "WV Offline TEC"=29.638450000000176, "WV Offline LD"=0.17, "WV Etalon TEC"=25.95, "HSRL Etalon TEC"=18.9999638, "HSRL TEC"=14.216749999999896, "HSRL LD"=0.16} {"HSRL LD" min=0.0 max=0.18 step=0.001 format="%.3p"; "HSRL TEC" min=14.0 max=28.0 step=0.1 format="%.3g"; "WV Offline LD" min=0.0 max=0.18 step=0.001 format="%.3p"; "WV Online LD" min=0.0 max=0.18 step=0.001 format="%.3p"; "HSRL Etalon TEC" format="%.2g"; "WV Etalon TEC" format="%.2g"; "WV Offline TEC" min=16.0 max=30.0 step=0.1 format="%.3g"; "WV Online TEC" min=14.0 max=28.0 step=0.1 format="%.3g"}
  out "Readings":T7={"Pro8000"=TRUE, "WV OnLine TEC"=23.2860966, "WV Online TEC"=TRUE, "WV Online LD"=0.17006056, "WV Online LD"=TRUE, "WV Offline TEC"=29.6523991, "WV Offline TEC"=TRUE, "WV Offline LD"=0.170357436, "WV Offline LD"=TRUE, "WV EtalonTEC"=25.9764748, "WV Etalon TEC"=TRUE, "HSRL Etalon TEC"=9.51464272, "HSRL Etalon TEC"=FALSE, "HSRL TEC"=14.2263737, "HSRL TEC "=TRUE, "HSRL LD"=0.1602754, "HSRL LD"=TRUE} {"HSRL LD" format="%.3p"; "HSRL TEC" format="%.3g"; "WV Offline LD" format="%.3p"; "WV Online LD" format="%.3p"; "HSRL Etalon TEC" format="%.3g"; "WV EtalonTEC" format="%.3g"; "WV Offline TEC" format="%.3g"; "WV OnLine TEC" format="%.3g"}
  in  "Pulse B Polarity":enum32{"Low", "High"}(ring)=enum."High"
  in  "Pulse A Delay(ns)":u32=1040 min=80 max=327600
  in  "Pulse B Delay(ns)":u32=170000 min=80 max=327600 step=1
  in  "Accumulation Delay(ns)":u32=10 min=10 max=1270 step=1
  in  "Sync Pulse Polarity":enum32{"Low", "High"}(ring)=enum."High"
  in  "Pulse A Polarity":enum32{"Low", "High"}(ring)=enum."High"
  in  "Number of Bins":u32=560 min=2 max=4095 step=1
  in  "Number of Accumulates":u32=14285 min=1 max=32767 step=1
  in  "Time Resolution Per Bin(ns)":u32=250 min=5 max=1063 step=1
  out "AMCS_Profile":i32=29429
  in  "WV Online Set (nm)":dbl=828.197 format="%.5f"
  out "WV Online Read (nm)":dbl=828.1970083204906 format="%.5f"
  out "WV Offline Read (nm)":dbl=828.2964850723449 format="%.5f"
  in  "WV Offline Set (nm)":dbl=828.29645 format="%.5f"
  in  "Bristol In":i32=5
  out "Bristol Out":i32
  out "Online_Diff":dbl=8.32049056498363e-06 format="%#_3e"
  out "Oflline_Diff":dbl=3.507234487187816e-05 format="%#_3e"
  out "WV Online Locked":bool=TRUE
  out "WV Oflline Locked":bool=TRUE
  in  "calculate absorption cross sections":bool
  in  "Online_Tol":dbl=5e-05 format="%#_15g"
  in  "Cancel online":bool
  in  "Offline_Tol":dbl=0.001 format="%#_15g"
  in  "Cancel Offline":bool
  in  "temp step size":dbl=0.00025 format="%#_6p"
  in  "HSRL_Tol":dbl=0.001 format="%#_15g"
  out "HSRL_Diff":dbl=-6.908048760578822e-05 format="%#_3e"
  in  "Cancel HSRL":bool
  out "HSRL Locked":bool=TRUE
  out "HSRL Read (nm)":dbl=780.2460509195124 format="%.5f"
  in  "HSRL Set (nm)":dbl=780.24612 format="%#.5f"
  in  "Smoothing Range":dbl=150.0
  in  "Total DIAL Integration Time (Minutes)":i32=3
  in  "Data Reads (number of loops)":i32=1
  in  "Total Aerosol Integration Time (Minutes)":dbl=0.5
  in  "Scalar Wait Time":u32
  out "Smoothed Bins":dbl=4.0
  in  "NewportIn":string
  in  "logging":bool
  out "Newport Device Key":string
  in  "SampleSize":i32=2
  out "NewportRef":refnum<k24>
  in  "Switch Comm Port":refnum<visa-resource-name>="COM3"
  out "FF_On_Ref":refnum<file>
  out "FF_On_Ptr":i64=4835904 format="%.2p"
  out "FF_Off_Ref":refnum<file>
  out "FF_Off_Ptr":i64=4835904 format="%.2p"
  out "NF_On_Ref":refnum<file>
  out "NF_On_Ptr":i64=4835904 format="%.2p"
  out "NF_Off_Ref":refnum<file>
  out "NF_Off_Ptr":i64=4835904 format="%.2p"
  out "DataOpen":bool=TRUE
  out "File Path_Far Field (out)":string="C:\\Users\\H2ODial\\Desktop\\SharedTeleWVData\\170321FF\\15"
  out "File Path_Near Field (out)":string="C:\\Users\\H2ODial\\Desktop\\SharedTeleWVData\\170321NF\\15"
  in  "Data File DIR (in)":string="C:\\Users\\H2ODial\\Desktop\\SharedTeleWVData\\"
  out "TRHP":T8={"Temp C"=7.387362637362642, "RelH %"=61.460622710622715, "Press hPa"=842.0054945054944, "AbH g/m^3"=4.63980463980464}
  in  "WS visa":refnum<visa-resource-name>="LuftWS"
  in  "WS_On/Off":bool=TRUE
  in  "bins":u32=560 min=2 max=4095 step=1
  out "y offset":u32=10
  in  "ns scale":u32=250
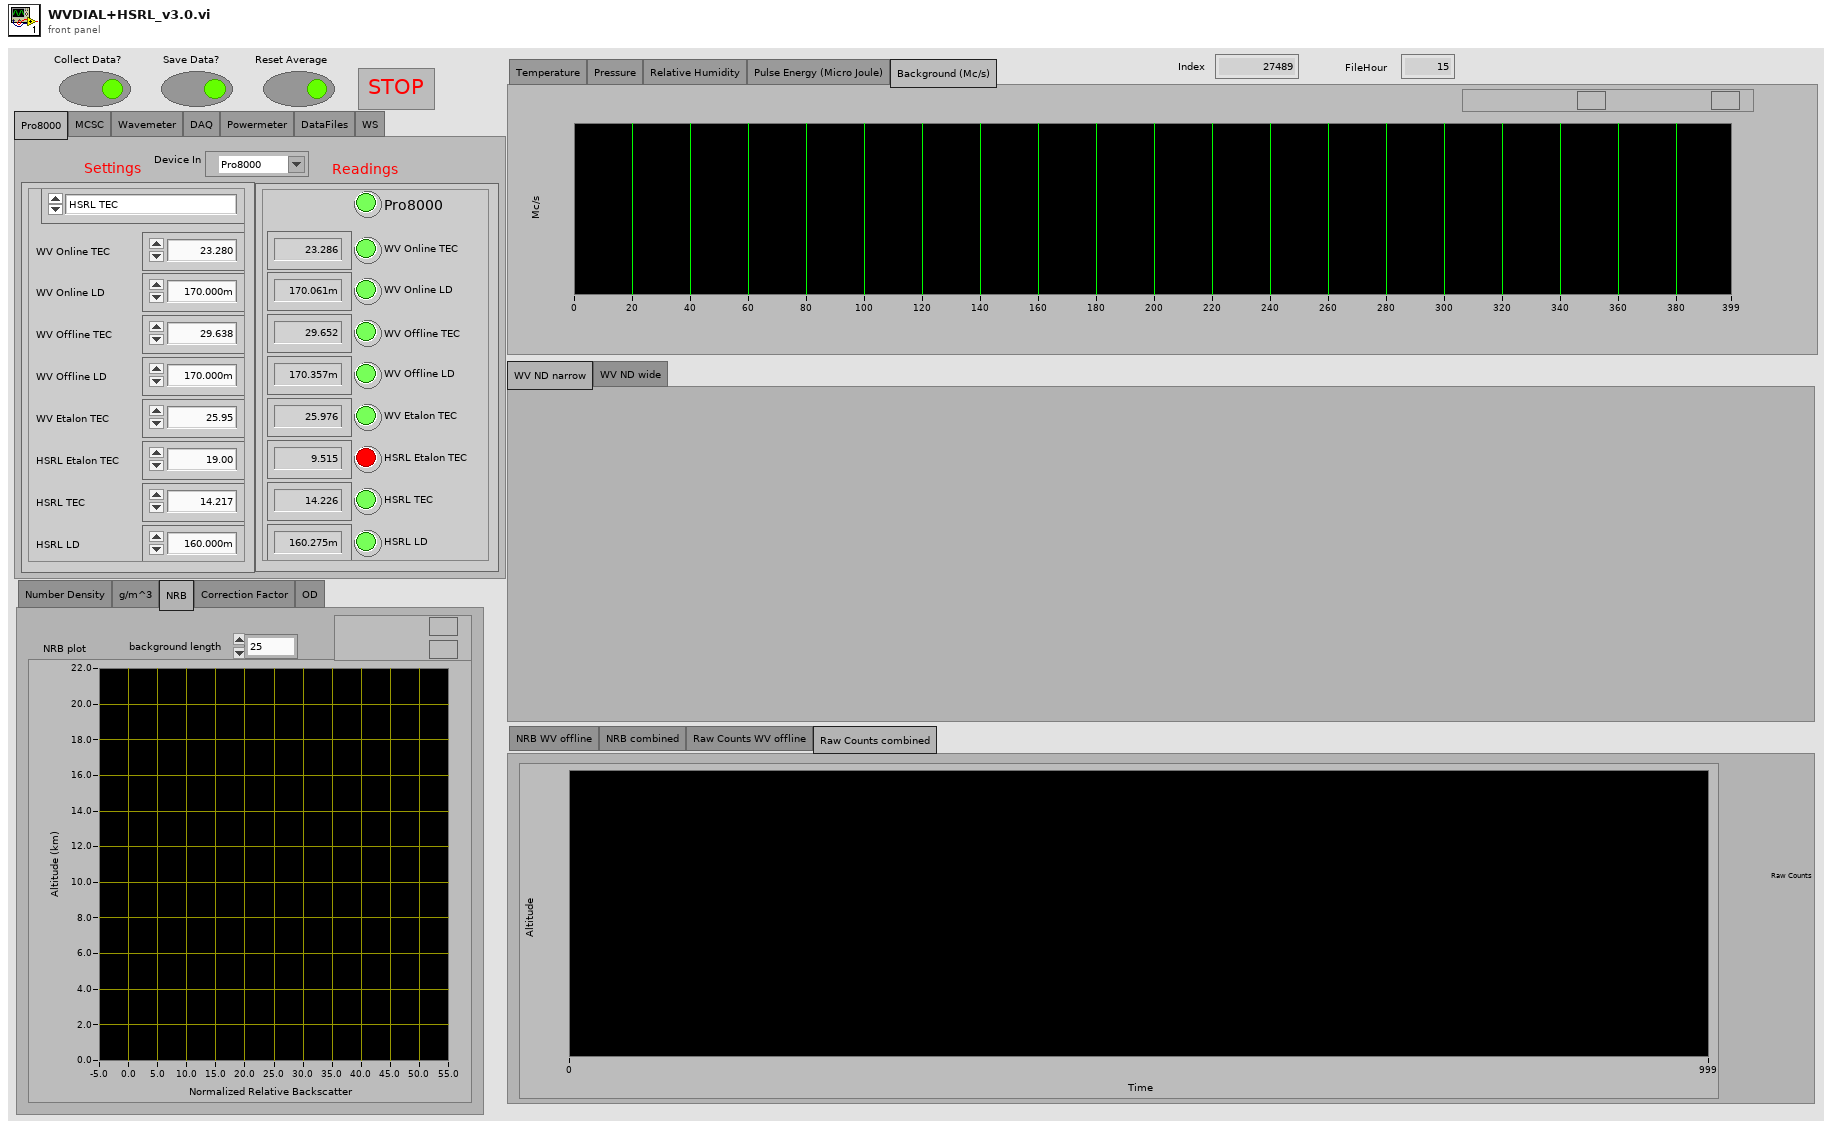
[diagram p1: front panel]
types:
  T1 = enum32{"NRB WV offline", "NRB combined", "Raw Counts WV offline", "Raw Counts combined"}
  T2 = enum32{"Number Density", "g/m^3", "NRB", "Correction Factor", "OD"}
  T3 = enum32{"Temperature", "Pressure", "Relative Humidity", "Pulse Energy (Micro Joule)", "Background (Mc/s)"}
  T4 = cluster{"Online Pulse Energy":dbl, "Pulse Energy Offline":dbl}
  T5 = enum32{"Pro8000", "MCSC", "Wavemeter", "DAQ", "Powermeter", "DataFiles", "WS"}
  T6 = cluster{"Module":enum16{"WV Online TEC", "WV Online LD", "WV Offline TEC", "WV Offline LD", "WV Etalon TEC", "HSRL Etalon TEC", "HSRL TEC", "HSRL LD"}, "WV Online TEC":dbl, "WV Online LD":dbl, "WV Offline TEC":dbl, "WV Offline LD":dbl, "WV Etalon TEC":dbl, "HSRL Etalon TEC":dbl, "HSRL TEC":dbl, "HSRL LD":dbl}
  T7 = cluster{"Pro8000":bool, "WV OnLine TEC":dbl, "WV Online TEC":bool, "WV Online LD":dbl, "WV Online LD":bool, "WV Offline TEC":dbl, "WV Offline TEC":bool, "WV Offline LD":dbl, "WV Offline LD":bool, "WV EtalonTEC":dbl, "WV Etalon TEC":bool, "HSRL Etalon TEC":dbl, "HSRL Etalon TEC":bool, "HSRL TEC":dbl, "HSRL TEC ":bool, "HSRL LD":dbl, "HSRL LD":bool}
  T8 = cluster{"Temp C":dbl, "RelH %":dbl, "Press hPa":dbl, "AbH g/m^3":dbl}
  T9 = enum16{"Open_TL", "Close_TL", "Verify_ID", "TEC_Sensor", "SET", "READ", "ON", "OFF", "Set_Limits", "Read_Limits", "Enable_Status", "Read_Status"}
  T10 = enum16{"Initialize ILX", "Set ON T", "Set Off T", "Set ON I", "Set Off I", "Set On Lim", "Set Off Lim", "Read ILX", "TEC ON/OFF", "LASER ON/OFF", "Status?", "ILX OFF"}
  T11 = enum16{"open", "replace", "create", "open or create", "replace or create", "replace or create with confirmation"}
  T12 = enum16{"WV Online TEC", "WV Online LD", "WV Offline TEC", "WV Offline LD", "WV Etalon TEC", "HSRL Etalon TEC", "HSRL TEC", "HSRL LD"}
  T13 = cluster{"Temp":dbl, "RelH":dbl, "Press":dbl, "AbH":dbl}
  T14 = typedef "LVDateTimeRec.ctl" = cluster{"fractional second":dbl, "second":i32, "minute":i32, "hour":i32, "day of month":i32, "month":i32, "year":i32, "day of week":i32, "day of year":i32, "DST":i32}
  T15 = cluster{"Online Pulse Energy":dbl, "Offline Pulse Energy":dbl}
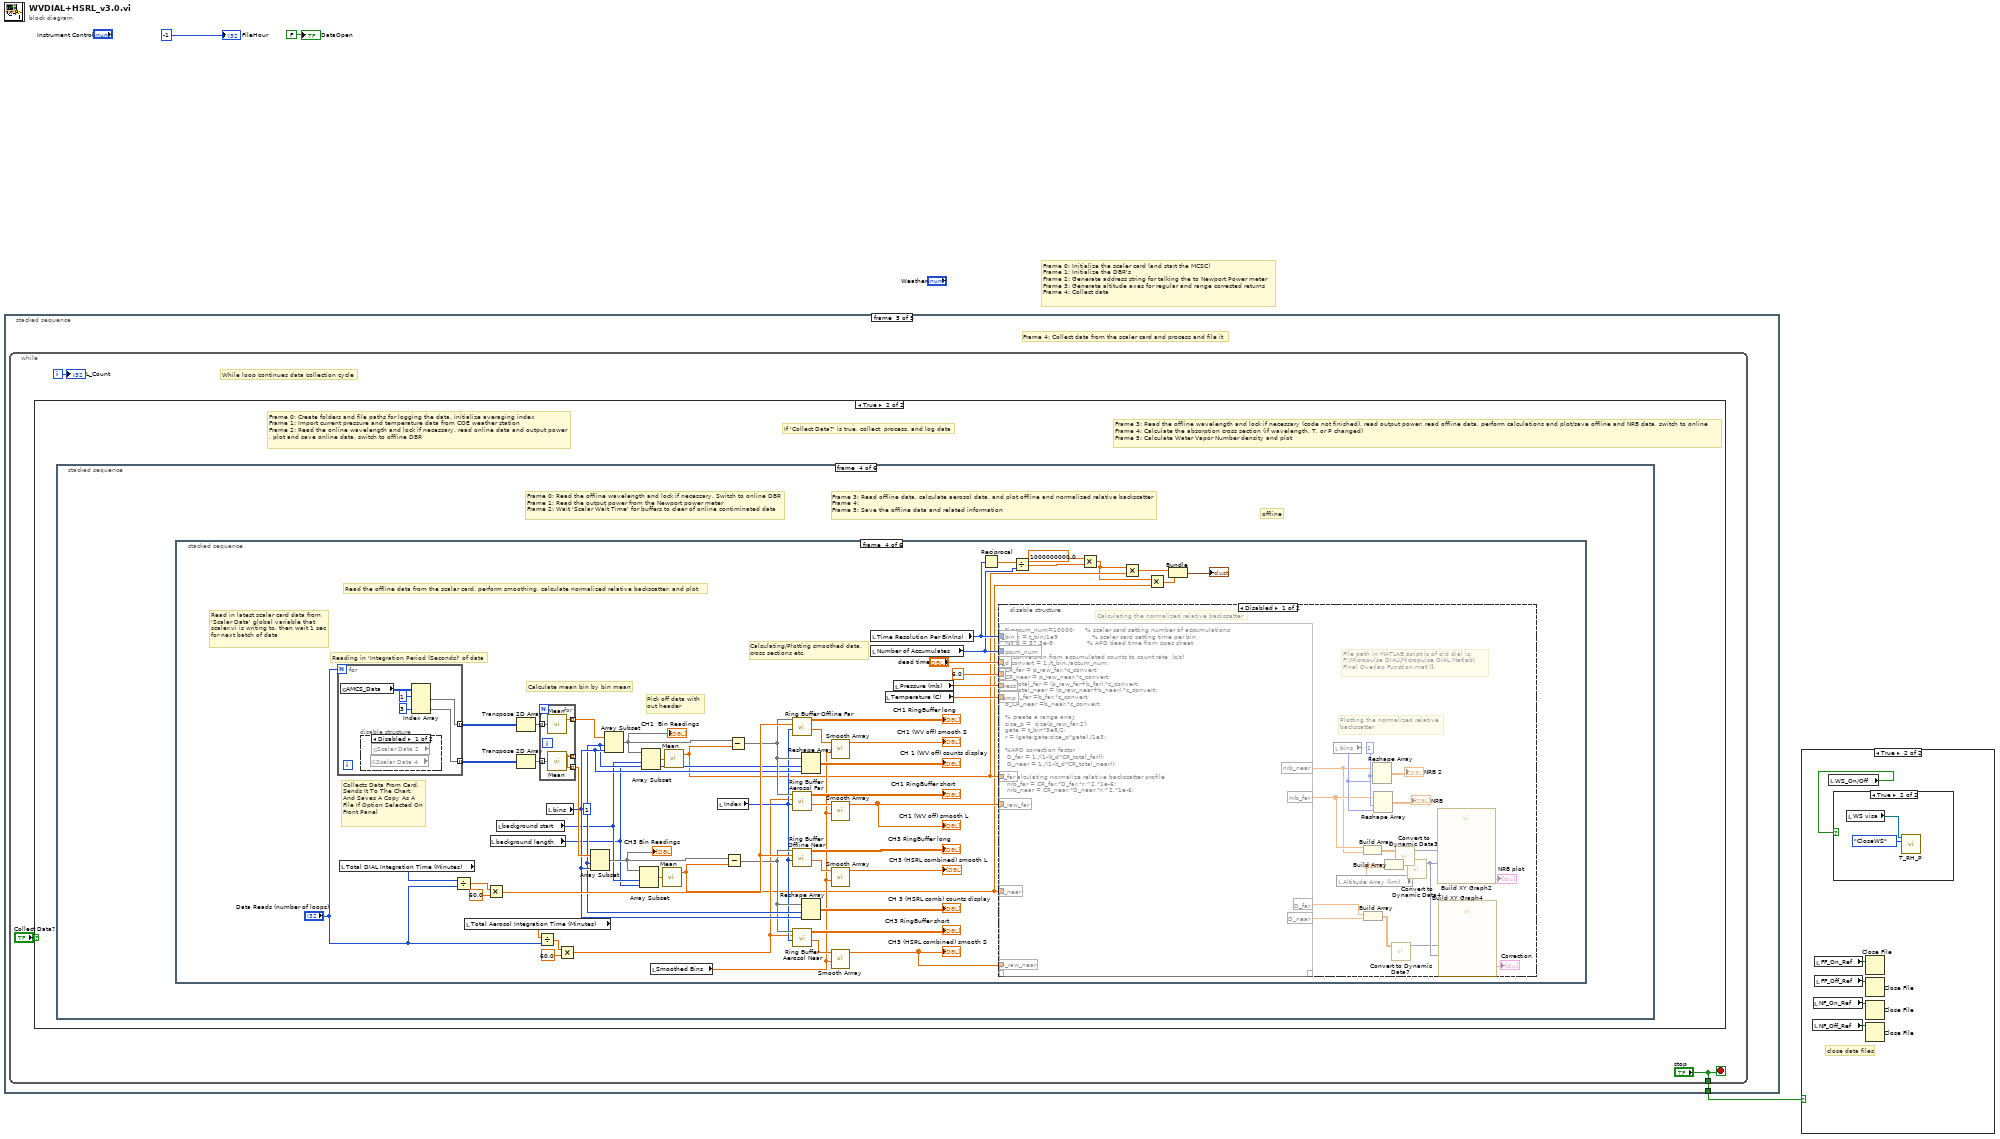
[diagram p0: block diagram]
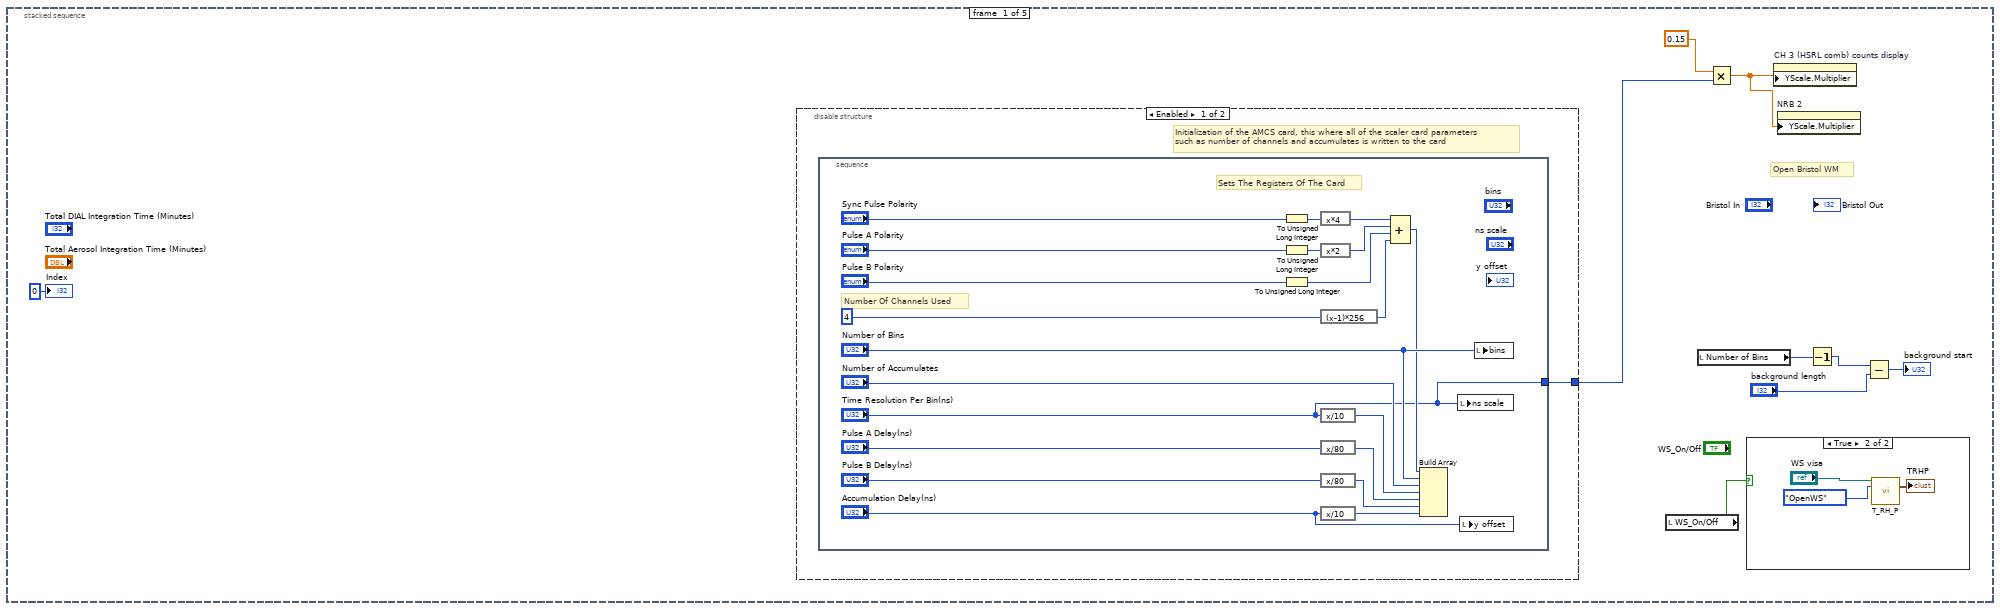
[diagram p4: hidden frame]
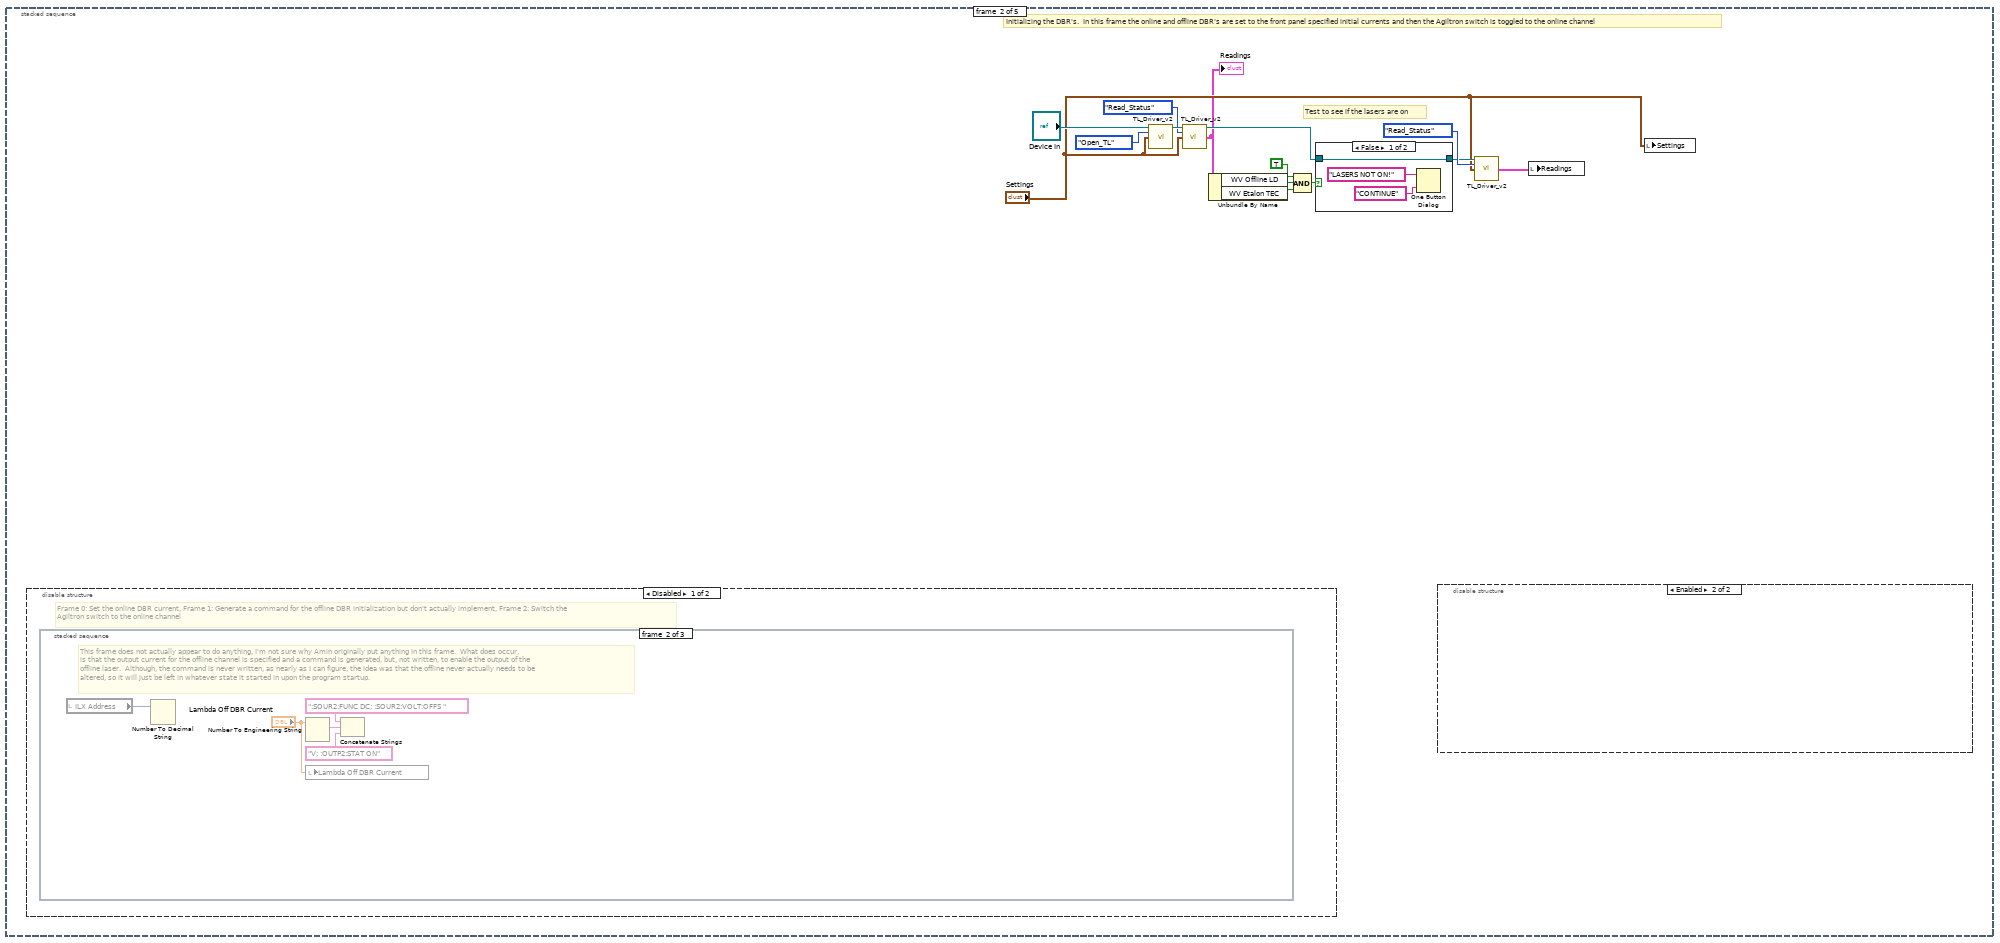
[diagram p7: hidden frame]
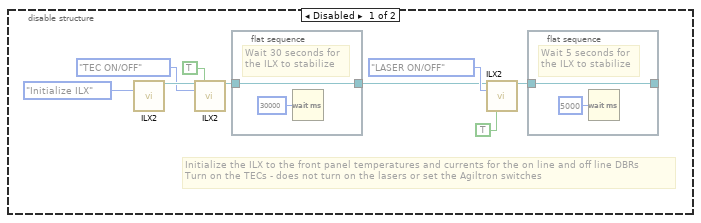
[diagram p9: hidden frame]
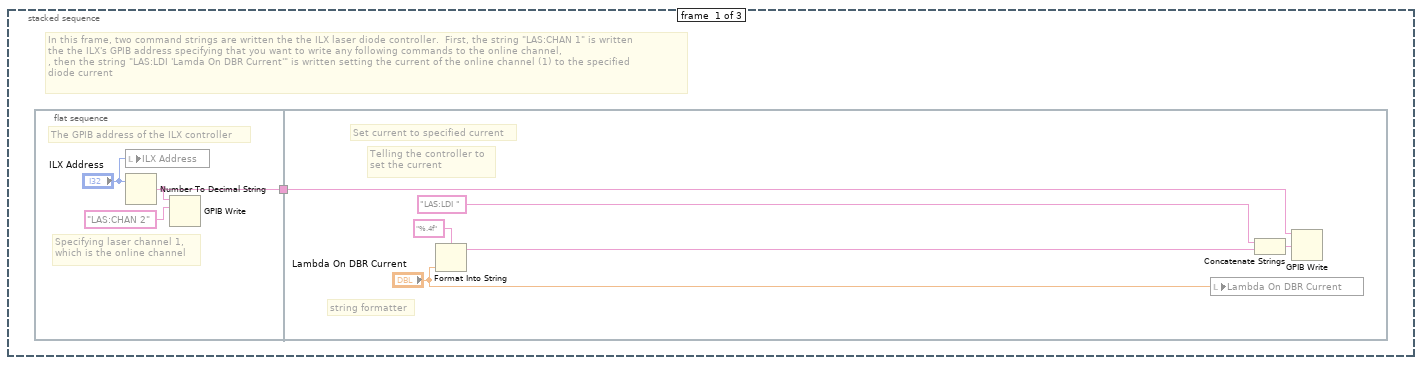
[diagram p10: hidden frame]
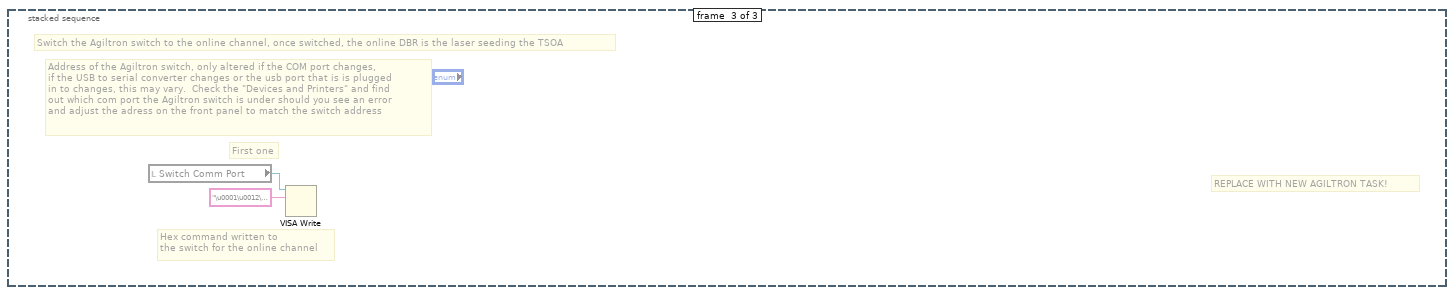
[diagram p11: hidden frame]
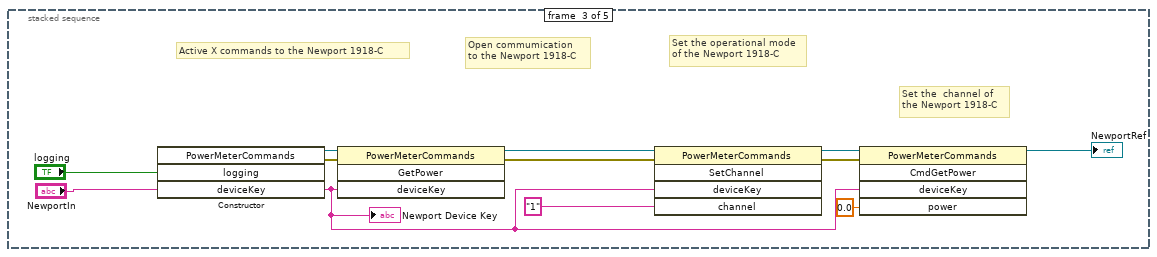
[diagram p13: hidden frame]
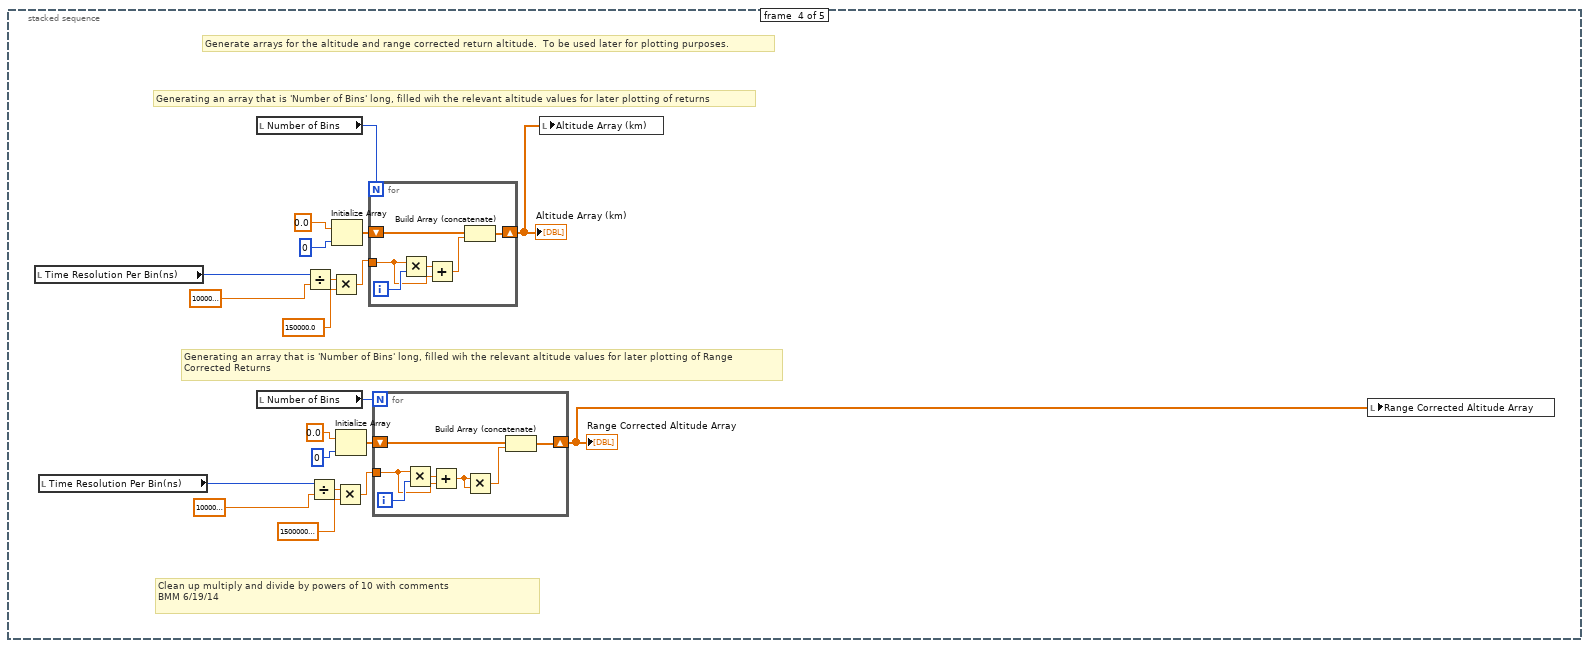
[diagram p14: hidden frame]
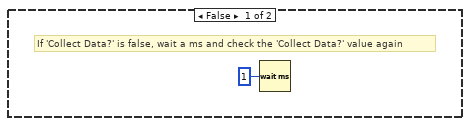
[diagram p15: hidden frame]
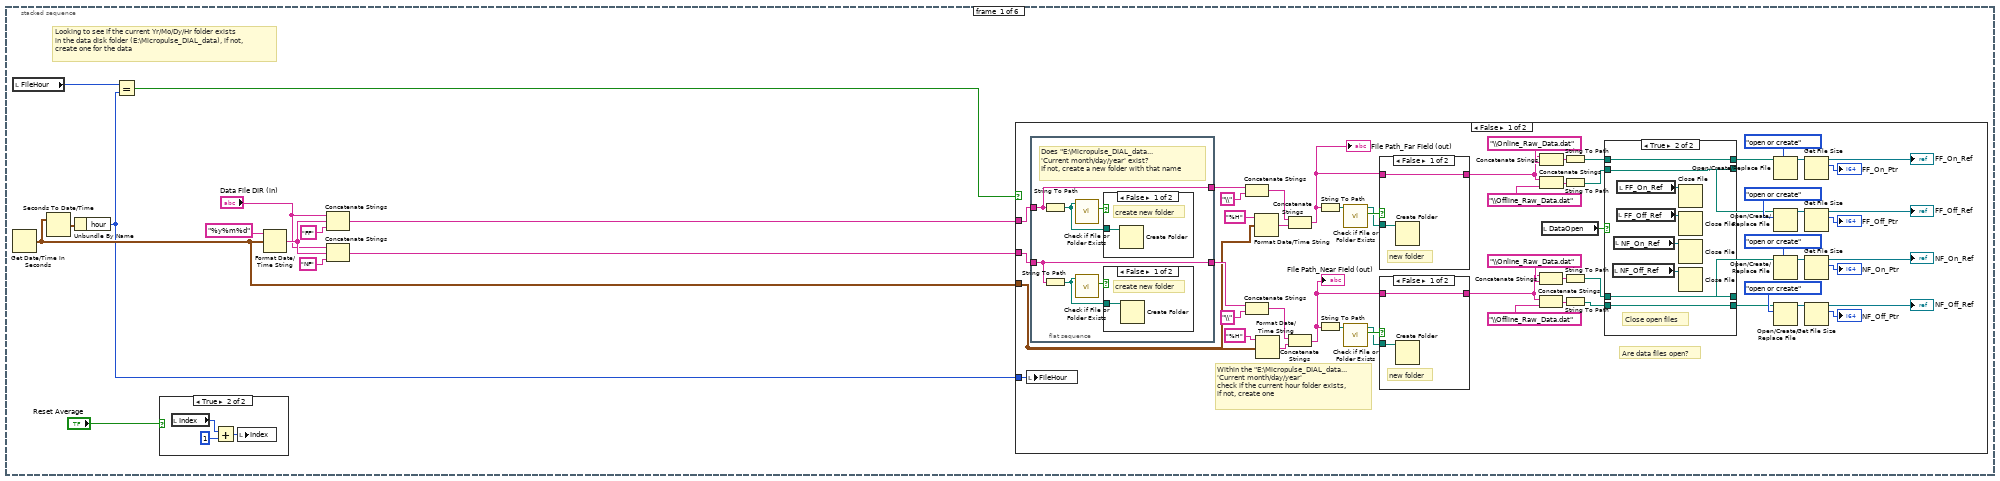
[diagram p16: hidden frame]
diagram:
  # "Frame 0: Initialize the scaler card (and start the MCSC)\nFrame 1: Initialize the DBR's\nFrame 2: Generate address string for talking the to Newport Power meter\nFrame 3: Generate altitude axes for regular and range corrected returns\nFrame 4: Collect data"
  n1 = stacked-sequence {
    tunnel: [_ _ _ _ w131] -> w3
    frame #0 {
      # "Open Bristol WM"
      n2 = disable-structure shown="Enabled" {
        disable-tunnel: [w16 _] -> w5
        frame Enabled {
          # "Initialization of the AMCS card, this where all of the scaler card parameters\nsuch as number of channels and accumulates is written to the card"
          n3 = stacked-sequence {
            tunnel: ["Time Resolution Per Bin(ns)"] -> w16
            frame #0 {
              # "Sets The Registers Of The Card"
              # "Number Of Channels Used"
              n4 = To Unsigned Long Integer(number="Sync Pulse Polarity") -> (unsigned 32bit integer=w18:u32)
              n5 = To Unsigned Long Integer(number="Pulse A Polarity") -> (unsigned 32bit integer=w22:u32)
              n6 = To Unsigned Long Integer(number="Pulse B Polarity") -> (unsigned 32bit integer=w20:u32)
              n7 = expression code="x*4"(w18) -> (w27:u32)
              n8 = expression code="x*2"(w22) -> (w26:u32)
              n9 = expression code="(x-1)*256"(u32 4 ("Number of Channels Used")) -> (w25:u32)
              n10 = expression code="x/10"("Time Resolution Per Bin(ns)") -> (w28:u32)
              n11 = expression code="x/80"("Pulse A Delay(ns)") -> (w35:u32)
              n12 = expression code="x/80"("Pulse B Delay(ns)") -> (w37:u32)
              n13 = expression code="x/10"("Accumulation Delay(ns)") -> (w36:u32)
              n14 = Compound Arithmetic op=ADD(w27, w26, w20, w25) -> (w24:u32)
              n15 = Build Array(w24, "Number of Bins", "Number of Accumulates", w28, w35, w37, w36) -> ()  [unwired: 1 out]
              n16 = local write "ns scale"("Time Resolution Per Bin(ns)") -> ()
              n17 = local write "y offset"("Accumulation Delay(ns)") -> ()
              n18 = local write "bins"("Number of Bins") -> ()
            }
          }
        }
        frame Disabled {
        }
      }
      n19 = local read "WS_On/Off"() -> (w7:bool)
      n20 = local read "Number of Bins"() -> (w11:u32)
      n21 = Multiply(x=0.15, y=w5) -> (x*y=w4:dbl)
      n22 = case shown="True" w7 {
        frame False {
        }
        frame True {
          n23 = call "T_RH_P.vi"("VISA in"="WS visa", "WS_Commands"=enum16{"OpenWS", "ReadTRHP", "CloseWS"}."OpenWS") -> ("TRHP"=→"TRHP":T13)  [unwired: 11 in, 2 out]
        }
      }
      n24 = property on="CH 3 (HSRL comb) counts display" class="IntChart (strict)"("YScale.Multiplier"=w4) -> ()  [unwired: 2 in, 2 out]
      n25 = property on="NRB 2" class="IntChart (strict)"("YScale.Multiplier"=w4) -> ()  [unwired: 2 in, 2 out]
      n26 = Decrement(x=w11) -> (x-1=w10:u32)
      n27 = Subtract(x=w10, y="background length") -> (x-y=→"background start":u32)
      "Index" <- 0 ("Index")
    }
    frame #1 {
      # "Test to see if the lasers are on"
      # "Initializing the DBR's.  In this frame the online and offline DBR's are set to the front panel specified initial currents and then the Agiltron switch is toggled to the online channel"
      n28 = disable-structure shown="Disabled" {
        frame Disabled {
          # "Frame 0: Set the online DBR current, Frame 1: Generate a command for the offline DBR initialization but don't actually implement, Frame 2: Switch the \nAgiltron switch to the online channel"
          n29 = stacked-sequence {
            frame #0 {
              # "In this frame, two command strings are written the the ILX laser diode controller.  First, the string \"LAS:CHAN 1\" is written\nthe the ILX's GPIB address specifying that you want to write any following commands to the online channel,\n, then the string \"LAS:LDI 'Lamda On DBR Current'\" is written setting the current of the online channel (1) to the specified \ndiode current"
              n30 = flat-sequence {
                tunnel: [w71] -> w69
                tunnel: w69 -> [w73]
                frame #0 {
                  # "The GPIB address of the ILX controller"
                  # "Specifying laser channel 1,\nwhich is the online channel"
                  n31 = local write "ILX Address"("ILX Address") -> ()
                  n32 = Number To Decimal String(number="ILX Address") -> (decimal integer string=w71:string)  [unwired: 1 in]
                  n33 = GPIB Write(0:w71, 1:"LAS:CHAN 2") -> ()  [unwired: 3 in, 2 out]
                }
                frame #1 {
                  # "Telling the controller to\nset the current"
                  # "string formatter"
                  # "Set current to specified current"
                  n34 = Format Into String(format string="%.4f" ("Format String"), "Lambda On DBR Current") -> (resulting string=w76:string)  [unwired: 2 in, 1 out]
                  n35 = local write "Lambda On DBR Current"("Lambda On DBR Current") -> ()
                  n36 = Concatenate Strings("LAS:LDI ", w76) -> (w77:string)
                  n37 = GPIB Write(0:w73, 1:w77) -> ()  [unwired: 3 in, 2 out]
                }
              }
            }
            frame #1 {
              # "This frame does not actually appear to do anything, I'm not sure why Amin originally put anything in this frame.  What does occur, \nis that the output current for the offline channel is specified and a command is generated, but, not written, to enable the output of the\noffline laser.  Although, the command is never written, as nearly as I can figure, the idea was that the offline never actually needs to be \naltered, so it will just be left in whatever state it started in upon the program startup."
              n38 = local read "ILX Address"() -> (w79:i32)
              n39 = Number To Decimal String(number=w79) -> ()  [unwired: 1 in, 1 out]
              n40 = Number To Engineering String(4:"Lambda Off DBR Current") -> (0:w83:string)  [unwired: 3 in]
              n41 = local write "Lambda Off DBR Current"("Lambda Off DBR Current") -> ()
              n42 = Concatenate Strings(":SOUR2:FUNC DC; :SOUR2:VOLT:OFFS ", w83, "V; :OUTP2:STAT ON") -> ()  [unwired: 1 out]
            }
            frame #2 {
              # "REPLACE WITH NEW AGILTRON TASK!"
              # "First one"
              # "Address of the Agiltron switch, only altered if the COM port changes,\nif the USB to serial converter changes or the usb port that is is plugged\nin to changes, this may vary.  Check the \"Devices and Printers\" and find \nout which com port the Agiltron switch is under should you see an error \nand adjust the adress on the front panel to match the switch address"
              # "Hex command written to \nthe switch for the online channel"
              # "Switch the Agiltron switch to the online channel, once switched, the online DBR is the laser seeding the TSOA"
              n43 = local read "Switch Comm Port"() -> (w84:refnum<visa-resource-name>)
              n44 = VISA Write(VISA resource name=w84, write buffer="\u0001\u0012\u0000\u0002") -> ()  [unwired: 1 in, 3 out]
            }
          }
        }
        frame Enabled {
        }
      }
      n45 = call "TL_Driver_v2.vi"("Device In"="Device In", "Commands"=T9."Open_TL", "Settings"="Settings") -> ("Device Out"=w49:refnum<visa-resource-name>)  [unwired: 9 in, 3 out]
      n46 = call "TL_Driver_v2.vi"("Device In"=w49, "Commands"=T9."Read_Status", "Settings"="Settings") -> ("Device Out"=w47:refnum<visa-resource-name>, "Readings"=w38:T7)  [unwired: 9 in, 2 out]
      "Readings" <- w38
      n47 = Unbundle By Name(w38) -> ("WV Offline LD"=w42:bool, "WV Etalon TEC"=w43:bool)
      n48 = Compound Arithmetic op=AND(TRUE, w42, w43) -> (w41:bool)
      n49 = case shown="False" w41 {
        tunnel: w47 -> [w52 w55]
        tunnel: [w52 w55] -> w45
        frame False {
          n50 = One Button Dialog(message="LASERS NOT ON!", button name ("OK")="CONTINUE") -> ()  [unwired: 1 out]
        }
        frame True {
        }
      }
      n51 = disable-structure shown="Enabled" {
        frame Disabled {
          # "Initialize the ILX to the front panel temperatures and currents for the on line and off line DBRs\nTurn on the TECs - does not turn on the lasers or set the Agiltron switches"
          n52 = call "ILX2.vi"("ILX Command"=T10."Initialize ILX") -> ("Device Out"=w63:refnum<visa-resource-name>)  [unwired: 10 in, 4 out]
          n53 = call "ILX2.vi"("Device In"=w63, "TEC Control"=TRUE, "ILX Command"=T10."TEC ON/OFF") -> ("Device Out"=w60:refnum<visa-resource-name>)  [unwired: 8 in, 4 out]
          n54 = flat-sequence {
            tunnel: w60 -> [w67]
            tunnel: [w67] -> w57
            frame #0 {
              # "Wait 30 seconds for\nthe ILX to stabilize"
              n55 = Wait (ms)(milliseconds to wait=u32 30000) -> ()  [unwired: 1 out]
            }
          }
          n56 = call "ILX2.vi"("Device In"=w57, "ILX Command"=T10."LASER ON/OFF", "Laser Control"=TRUE ("TEC Control")) -> ("Device Out"=w56:refnum<visa-resource-name>)  [unwired: 8 in, 4 out]
          n57 = flat-sequence {
            tunnel: w56 -> [w65]
            tunnel: [w65] -> _
            frame #0 {
              # "Wait 5 seconds for\nthe ILX to stabilize"
              n58 = Wait (ms)(milliseconds to wait=u32 5000) -> ()  [unwired: 1 out]
            }
          }
        }
        frame Enabled {
        }
      }
      n59 = call "TL_Driver_v2.vi"("Device In"=w45, "Commands"=T9."Read_Status", "Settings"="Settings") -> ("Readings"=w40:T7)  [unwired: 9 in, 3 out]
      n60 = local write "Readings"(w40) -> ()
      n61 = local write "Settings"("Settings") -> ()
    }
    frame #2 {
      # "Active X commands to the Newport 1918-C"
      # "Set the  channel of\nthe Newport 1918-C"
      # "Set the operational mode\nof the Newport 1918-C"
      # "Open commumication\nto the Newport 1918-C"
      n62 = constructor class="PowerMeterCommands"("logging"="logging", "deviceKey"="NewportIn") -> (reference out=w97:refnum<k24>, error out=w94:errorcluster, "deviceKey"=w89:string)  [unwired: 3 in, 2 out]
      "Newport Device Key" <- w89
      n63 = invoke class="PowerMeterCommands" method="GetPower"(reference=w97, error in=w94, "deviceKey"=w89) -> (reference out=w96:refnum<k24>, error out=w93:errorcluster)  [unwired: 1 in, 2 out]
      n64 = invoke class="PowerMeterCommands" method="SetChannel"(reference=w96, error in=w93, "deviceKey"=w89, "channel"="1") -> (reference out=w90:refnum<k24>, error out=w92:errorcluster)  [unwired: 1 in, 3 out]
      n65 = invoke class="PowerMeterCommands" method="CmdGetPower"(reference=w90, error in=w92, "deviceKey"=w89, "power"=sgl 0.0) -> (reference out=→"NewportRef":refnum<k24>)  [unwired: 1 in, 4 out]
    }
    frame #3 {
      # "Clean up multiply and divide by powers of 10 with comments\nBMM 6/19/14"
      # "Generating an array that is 'Number of Bins' long, filled wih the relevant altitude values for later plotting of Range \nCorrected Returns"
      # "Generating an array that is 'Number of Bins' long, filled wih the relevant altitude values for later plotting of returns"
      # "Generate arrays for the altitude and range corrected return altitude.  To be used later for plotting purposes."
      n66 = local read "Time Resolution Per Bin(ns)"() -> (w110:u32)
      n67 = local read "Time Resolution Per Bin(ns)"() -> (w100:u32)
      n68 = local read "Number of Bins"() -> (w113:u32)
      n69 = local read "Number of Bins"() -> (w103:u32)
      n70 = Divide(x=w110, y=1000000000.0) -> (x/y=w108:dbl)
      n71 = Divide(x=w100, y=1000000000.0) -> (x/y=w98:dbl)
      n72 = Multiply(x=w108, y=150000.0) -> (x*y=w111:dbl)
      n73 = Initialize Array(0.0, 0) -> (w116:dbl[])
      n74 = Multiply(x=w98, y=150000000.0) -> (x*y=w101:dbl)
      n75 = Initialize Array(0.0, 0) -> (w106:dbl[])
      n76 = for {
        N: w113 -> [_]
        shift-right: [w129] -> w114
        shift-left: w116 -> [w130]
        tunnel: w111 -> [w126]
        i -> [w128]
        n77 = Multiply(x=w126, y=w128) -> (x*y=w127:dbl)
        n78 = Add(x=w127, y=w126) -> (x+y=w125:dbl)
        n79 = Build Array (concatenate)(w130, w125) -> (w129:dbl[])
      }
      "Altitude Array (km)" <- w114
      n80 = for {
        N: w103 -> [_]
        shift-right: [w123] -> w104
        shift-left: w106 -> [w124]
        tunnel: w101 -> [w119]
        i -> [w122]
        n81 = Multiply(x=w119, y=w122) -> (x*y=w120:dbl)
        n82 = Add(x=w120, y=w119) -> (x+y=w118:dbl)
        n83 = Multiply(x=w118, y=w118) -> (x*y=w121:dbl)
        n84 = Build Array (concatenate)(w124, w121) -> (w123:dbl[])
      }
      "Range Corrected Altitude Array" <- w104
      n85 = local write "Altitude Array (km)"(w114) -> ()
      n86 = local write "Range Corrected Altitude Array"(w104) -> ()
    }
    frame #4 {
      # "Frame 4: Collect data from the scaler card and process and file it"
      n87 = while {
        tunnel: ["stop"] -> w131
        i -> [w132]
        stop <- "stop" stop-if-true
        # "While loop continues data collection cycle"
        n88 = case shown="True" "Collect Data?" {
          frame False {
            # "If 'Collect Data?' is false, wait a ms and check the 'Collect Data?' value again"
            n89 = Wait (ms)(milliseconds to wait=u32 1) -> ()  [unwired: 1 out]
          }
          frame True {
            # "Frame 3: Read the offline wavelength and lock if necessary (code not finished), read output power, read offline data, perform calculations and plot/save offline and NRB data, switch to online\nFrame 4: Calculate the absorption cross section (if wavelength, T, or P changed)\nFrame 5: Calculate Water Vapor Number density and plot"
            # "Frame 0: Create folders and file paths for logging the data, initialize averaging index\nFrame 1: Import current pressure and temperature data from COE weather station\nFrame 2: Read the online wavelength and lock if necessary, read online data and output power\n, plot and save online data, switch to offline DBR"
            # "If 'Collect Data?' is true, collect, process, and log data"
            n90 = stacked-sequence {
              frame #0 {
                # "Looking to see if the current Yr/Mo/Dy/Hr folder exists\nin the data disk folder (E:\\Micropulse_DIAL_data), if not,\ncreate one for the data"
                n91 = local read "FileHour"() -> (w145:i32)
                n92 = Get Date/Time In Seconds() -> (seconds since 1Jan1904=w137:timestamp)
                n93 = Seconds To Date/Time(time stamp (now)=w137) -> (date time rec=w147:T14)  [unwired: 1 in]
                n94 = Unbundle By Name(w147) -> ("hour"=w136:i32)
                n95 = Equal?(x=w145, y=w136) -> (x = y?=w146:bool)
                n96 = case shown="True" "Reset Average" {
                  frame False {
                    n97 = local write "Index"(0 ("Index")) -> ()
                  }
                  frame True {
                    n98 = local read "Index"() -> (w235:i32)
                    n99 = Add(x=w235, y=1) -> (x+y=w234:i32)
                    n100 = local write "Index"(w234) -> ()
                  }
                }
                n101 = Format Date/Time String(time format string (%c)="%y%m%d", seconds (now)=w137) -> (date/time string=w141:string)  [unwired: 1 in]
                n102 = Concatenate Strings("Data File DIR (in)", w141, "FF" ("string")) -> (w143:string)
                n103 = Concatenate Strings("Data File DIR (in)", w141, "NF" ("string")) -> (w138:string)
                n104 = case shown="False" w146 {
                  tunnel: w143 -> [w205 _]
                  tunnel: w138 -> [w204 _]
                  tunnel: w137 -> [w191 _]
                  tunnel: w136 -> [w167 _]
                  frame False {
                    # "Are data files open?"
                    # "Within the \"E:\\Micropulse_DIAL_data...\n'Current month/day/year' \ncheck if the current hour folder exists,\nif not, create one"
                    n105 = local write "FileHour"(w167) -> ()
                    n106 = flat-sequence {
                      tunnel: [w225] -> w192
                      tunnel: w205 -> [w224]
                      tunnel: w204 -> [w225]
                      tunnel: [w224] -> w193
                      frame #0 {
                        # "Does \"E:\\Micropulse_DIAL_data...\n'Current month/day/year' exist?\nIf not, create a new folder with that name"
                        n107 = String To Path(string=w224) -> (path=w229:path)
                        n108 = String To Path(string=w225) -> (path=w227:path)
                        n109 = call <vilib>:"Check if File or Folder Exists.vi"("path"=w229) -> ("file or folder exists?"=w228:bool)  [unwired: 8 in, 2 out]
                        n110 = call <vilib>:"Check if File or Folder Exists.vi"("path"=w227) -> ("file or folder exists?"=w226:bool)  [unwired: 8 in, 2 out]
                        n111 = case shown="False" w228 {
                          tunnel: w229 -> [w231 _]
                          frame False {
                            # "create new folder"
                            n112 = Create Folder(path (use dialog)=w231) -> ()  [unwired: 2 in, 3 out]
                          }
                          frame True {
                            # "Folder exists\ndo nothing"
                          }
                        }
                        n113 = case shown="False" w226 {
                          tunnel: w227 -> [w230 _]
                          frame False {
                            # "create new folder"
                            n114 = Create Folder(path (use dialog)=w230) -> ()  [unwired: 2 in, 3 out]
                          }
                          frame True {
                            # "Folder exists\ndo nothing"
                          }
                        }
                      }
                    }
                    n115 = Concatenate Strings(w193, "\\" ("string")) -> (w200:string)
                    n116 = Concatenate Strings(w192, "\\" ("string")) -> (w195:string)
                    n117 = Format Date/Time String(time format string (%c)="%H", seconds (now)=w191) -> (date/time string=w203:string)  [unwired: 1 in]
                    n118 = Format Date/Time String(time format string (%c)="%H", seconds (now)=w191) -> (date/time string=w198:string)  [unwired: 1 in]
                    n119 = Concatenate Strings(w200, w203) -> (w163:string)
                    "File Path_Far Field (out)" <- w163
                    n120 = Concatenate Strings(w195, w198) -> (w164:string)
                    "File Path_Near Field (out)" <- w164
                    n121 = String To Path(string=w163) -> (path=w201:path)
                    n122 = String To Path(string=w164) -> (path=w196:path)
                    n123 = call <vilib>:"Check if File or Folder Exists.vi"("path"=w201) -> ("file or folder exists?"=w190:bool, "dup path"=w188:path)  [unwired: 8 in, 1 out]
                    n124 = call <vilib>:"Check if File or Folder Exists.vi"("path"=w196) -> ("file or folder exists?"=w189:bool, "dup path"=w187:path)  [unwired: 8 in, 1 out]
                    n125 = case shown="False" w190 {
                      tunnel: w188 -> [w222 _]
                      tunnel: w163 -> [w221 w223]
                      tunnel: [w221 w223] -> w161
                      frame False {
                        # "new folder"
                        n126 = Create Folder(path (use dialog)=w222) -> ()  [unwired: 2 in, 3 out]
                      }
                      frame True {
                        # "Folder exists\ndo nothing"
                      }
                    }
                    n127 = case shown="False" w189 {
                      tunnel: w187 -> [w219 _]
                      tunnel: w164 -> [w218 w220]
                      tunnel: [w218 w220] -> w162
                      frame False {
                        # "new folder"
                        n128 = Create Folder(path (use dialog)=w219) -> ()  [unwired: 2 in, 3 out]
                      }
                      frame True {
                        # "Folder exists\ndo nothing"
                      }
                    }
                    n129 = Concatenate Strings(w162, "\\Online_Raw_Data.dat" ("string")) -> (w181:string)
                    n130 = Concatenate Strings(w162, "\\Offline_Raw_Data.dat" ("string")) -> (w180:string)
                    n131 = Concatenate Strings(w161, "\\Online_Raw_Data.dat" ("string")) -> (w186:string)
                    n132 = Concatenate Strings(w161, "\\Offline_Raw_Data.dat" ("string")) -> (w185:string)
                    n133 = local read "DataOpen"() -> (w178:bool)
                    n134 = String To Path(string=w186) -> (path=w177:path)
                    n135 = String To Path(string=w185) -> (path=w176:path)
                    n136 = String To Path(string=w181) -> (path=w175:path)
                    n137 = String To Path(string=w180) -> (path=w174:path)
                    n138 = case shown="True" w178 {
                      tunnel: w177 -> [w209 w213]
                      tunnel: [w209 w213] -> w171
                      tunnel: w176 -> [w208 w212]
                      tunnel: [w208 w212] -> w170
                      tunnel: w175 -> [w207 w211]
                      tunnel: [w207 w211] -> w169
                      tunnel: [w206 w210] -> w168
                      tunnel: w174 -> [w206 w210]
                      frame False {
                        # "No files open\ndo nothing"
                      }
                      frame True {
                        # "Close open files"
                        n139 = local read "NF_Off_Ref"() -> (w215:refnum<file>)
                        n140 = local read "NF_On_Ref"() -> (w214:refnum<file>)
                        n141 = local read "FF_Off_Ref"() -> (w217:refnum<file>)
                        n142 = local read "FF_On_Ref"() -> (w216:refnum<file>)
                        n143 = Close File(refnum=w216) -> ()  [unwired: 1 in, 2 out]
                        n144 = Close File(refnum=w217) -> ()  [unwired: 1 in, 2 out]
                        n145 = Close File(refnum=w214) -> ()  [unwired: 1 in, 2 out]
                        n146 = Close File(refnum=w215) -> ()  [unwired: 1 in, 2 out]
                      }
                    }
                    n147 = Open/Create/Replace File(file path (use dialog)=w171, operation (0:open)=T11."open or create") -> (refnum out=w157:refnum<file>)  [unwired: 4 in, 2 out]
                    n148 = Open/Create/Replace File(file path (use dialog)=w170, operation (0:open)=T11."open or create") -> (refnum out=w158:refnum<file>)  [unwired: 4 in, 2 out]
                    n149 = Open/Create/Replace File(file path (use dialog)=w169, operation (0:open)=T11."open or create") -> (refnum out=w159:refnum<file>)  [unwired: 4 in, 2 out]
                    n150 = Open/Create/Replace File(file path (use dialog)=w168, operation (0:open)=T11."open or create") -> (refnum out=w160:refnum<file>)  [unwired: 4 in, 2 out]
                    n151 = Get File Size(file=w157) -> (refnum out=→"FF_On_Ref":refnum<file>, size (in bytes)=→"FF_On_Ptr":i64)  [unwired: 1 in, 1 out]
                    n152 = Get File Size(file=w158) -> (refnum out=→"FF_Off_Ref":refnum<file>, size (in bytes)=→"FF_Off_Ptr":i64)  [unwired: 1 in, 1 out]
                    n153 = Get File Size(file=w159) -> (refnum out=→"NF_On_Ref":refnum<file>, size (in bytes)=→"NF_On_Ptr":i64)  [unwired: 1 in, 1 out]
                    n154 = Get File Size(file=w160) -> (refnum out=→"NF_Off_Ref":refnum<file>, size (in bytes)=→"NF_Off_Ptr":i64)  [unwired: 1 in, 1 out]
                  }
                  frame True {
                    # "Don't need to do anything!"
                  }
                }
              }
              frame #1 {
                # "Writing and plotting retrieved\nweather parameters"
                # "Matlab script goes online and retrieves most recent press, temp, and relative humidity data \nfrom the weather station on the roof of Cobleigh"
                # "Importing the current weather conditions from the COE weather station"
                n155 = disable-structure shown="Disabled" {
                  frame Disabled {
                    n156 = script code="%try\n%s=urlread('http://www.coe.montana.edu/ee/weather/mostCurrentCSV.php');\n%amin=textscan(s,'%s %s %s %s %s %s %s %s %s %s %s %s %s');\n%data=amin{1}{2};\n%[test remain]=strtok(data,',');\n%remain=str2num(remain);\n%press=remain(3)./1000;\n%temp=remain(5);\n%RH=remain(7);\n%catch\npress=.850;\ntemp=20;\nRH=40;\n%end"() -> ()  [unwired: 1 in, 4 out]
                  }
                  frame Enabled {
                  }
                }
                n157 = local read "WS_On/Off"() -> (w236:bool)
                n158 = case shown="True" w236 {
                  frame False {
                  }
                  frame True {
                    n159 = local read "WS visa"() -> (w241:refnum<visa-resource-name>)
                    n160 = call "T_RH_P.vi"("VISA in"=w241, "WS_Commands"=enum16{"OpenWS", "ReadTRHP", "CloseWS"}."ReadTRHP") -> ("TRHP"=w237:T13)  [unwired: 11 in, 2 out]
                    n161 = local write "TRHP"(w237) -> ()
                    n162 = Unbundle By Name(w237) -> ("Temp"=→"Temperature (C)":dbl, "RelH"=→"Relative Humdity (%)":dbl, "Press"=→"Pressure (mb)":dbl)
                  }
                }
              }
              frame #2 {
                # "Frame 3: Read, process, and plot online data\nFrame 4:\nFrame 5: Write the data to the folders from Frame 0 of outter sequence"
                # "Frame 0: Read the online wavelength and adjust to locking tolerance if out of range, Switch to offline DBR\nFrame 1: Read the output power from the Newport meter, calculate and plot the output pulse energy\nFrame 2: Wait 'Scalar Wait Time' for buffer to clear other wavelength data"
                # "Online"
                n163 = stacked-sequence {
                  frame #0 {
                    # "Read the online wavelength and continue adjusting the online DBR if outside the wavelength tolerance\nuntil it is within tolerance"
                    n164 = while {
                      i -> [w246]
                      stop <- w243 stop-if-true
                      # "Frame 2: Decrement DBR current if above tolerance\nFrame 3: Increment DBR current if below tolerance"
                      # "Frame 0: Read the current wavelength from the wavemeter\nFrame 1: Calculate the difference between desired and actual wavelength"
                      # "Continue reading and adjusting online DBR current until within locking tolerance"
                      n165 = stacked-sequence {
                        tunnel: w246 -> [w248 _ _ _ _]
                        tunnel: [_ _ w265 _ _] -> w244
                        frame #0 {
                          n166 = Equal To 0?(x=w248) -> (x = 0?=w247:bool)
                          n167 = case shown="True" w247 {
                            frame False {
                            }
                            frame True {
                              # "Set the wavemeter switch to WV Online"
                              n168 = Build Array(FALSE ("Boolean")) -> (w249:bool[])
                              n169 = Build Array(FALSE ("Boolean")) -> (w252:bool[])
                              n170 = call-poly <vilib>:"DAQmx Write.vi"("task/channels in"=refnum<k21> "BristolWM", "data"=w252) -> ()  [unwired: 11 in, 3 out]
                              n171 = call-poly <vilib>:"DAQmx Write.vi"("task/channels in"=refnum<k21> "HSRL_WV_switch", "data"=w249) -> ()  [unwired: 11 in, 3 out]
                            }
                          }
                        }
                        frame #1 {
                          # "Reading the wavelength from the wavemeter"
                          n172 = flat-sequence {
                            tunnel: [w257] -> w256
                            tunnel: w256 -> [w260]
                            tunnel: [w259] -> w255
                            tunnel: w255 -> [w263]
                            frame #0 {
                              n173 = local read "Bristol In"() -> (w258:i32)
                              n174 = dll-call lib="C:/Users/H2ODial/Desktop/Shared Telescope WV DIAL Code/bristol/CLDevIface.dll" fn="CLOpenUSBSerialDevice"("commPort"=w258) -> ("return type"=w257:i32)  [unwired: 4 in, 2 out]
                            }
                            frame #1 {
                              n175 = dll-call lib="C:/Users/H2ODial/Desktop/Shared Telescope WV DIAL Code/bristol/CLDevIface.dll" fn="CLGetLambdaReading"("devHandle"=w260) -> ("return type"=→"WV Online Read (nm)":dbl, "devHandle"=w259:i32)  [unwired: 3 in, 2 out]
                            }
                            frame #2 {
                              n176 = dll-call lib="C:/Users/H2ODial/Desktop/Shared Telescope WV DIAL Code/bristol/CLDevIface.dll" fn="CLCloseDevice"("commPort"=w263) -> ("return type"=w262:i32)  [unwired: 4 in, 2 out]
                              n177 = local write "Bristol Out"(w262) -> ()
                            }
                          }
                        }
                        frame #2 {
                          # "If WL difference is within tolerance, stop looping, and illuminate 'Wavelength Lock Online' indicator"
                          # "Calculating the difference between the actual and desired online wavelength"
                          n178 = local read "WV Online Read (nm)"() -> (w264:dbl)
                          n179 = local read "Online_Tol"() -> (w270:dbl)
                          n180 = Multiply(x=-1.0, y=w270) -> (x*y=w271:dbl)
                          n181 = Subtract(x=w264, y="WV Online Set (nm)") -> (x-y=w266:dbl)
                          "Online_Diff" <- w266
                          n182 = Greater?(x=w266, y=w271) -> (0:w267:bool)
                          n183 = Less?(x=w266, y=w270) -> (x < y?=w268:bool)
                          n184 = And(x=w267, y=w268) -> (x .and. y?=w265:bool)
                          "WV Online Locked" <- w265
                        }
                        frame #3 {
                          # "If the wavelength difference is greater that 0.0002 nm, decrement the \nDBR current by 0.01 mA"
                          n185 = local read "Online_Diff"() -> (w275:dbl)
                          n186 = Greater Or Equal?(x=w275, y="Online_Tol") -> (x >= y?=w274:bool)
                          n187 = case shown="True" w274 {
                            frame False {
                              # "Wavelength difference is not greater than 0.0002 nm, do nothing"
                            }
                            frame True {
                              # "Generating a command string\nto decrement the current"
                              # "WL difference is greater than 0.0002 nm,\ndecrement the DBR current by 0.01 mA"
                              n188 = local read "Settings"() -> (w282:T6)
                              n189 = local read "temp step size"() -> (w277:dbl)
                              n190 = Unbundle By Name(w282) -> ("WV Online TEC"=w281:dbl)
                              n191 = local read "Device In"() -> (w278:refnum<visa-resource-name>)
                              n192 = Subtract(x=w281, y=w277) -> (x-y=w280:dbl)
                              n193 = Bundle By Name(cluster=w282, "WV Online TEC"=w280, "Module"=T12."WV Online TEC") -> (w284:T6)
                              n194 = call "TL_Driver_v2.vi"("Device In"=w278, "Commands"=T9."SET", "Settings"=w284) -> ("Readings"=w283:T7)  [unwired: 9 in, 3 out]
                              n195 = local write "Settings"(w284) -> ()
                              n196 = local write "Readings"(w283) -> ()
                            }
                          }
                        }
                        frame #4 {
                          # "If WL difference is < 0.0002 nm, increment the DBR current"
                          n197 = local read "Online_Tol"() -> (w286:dbl)
                          n198 = local read "Online_Diff"() -> (w289:dbl)
                          n199 = Multiply(x=-1.0, y=w286) -> (x*y=w285:dbl)
                          n200 = Less Or Equal?(x=w289, y=w285) -> (x <= y?=w288:bool)
                          n201 = case shown="True" w288 {
                            frame False {
                              # "WL difference is no <= to -0.0002 nm, do nothing"
                            }
                            frame True {
                              # "WL difference is < -0.0002,\nincrement the DBR current by 0.01 mA"
                              # "Generating a command string\nto decrement the current"
                              n202 = local read "Settings"() -> (w298:T6)
                              n203 = local read "temp step size"() -> (w291:dbl)
                              n204 = Unbundle By Name(w298) -> ("WV Online TEC"=w295:dbl)
                              n205 = local read "Device In"() -> (w292:refnum<visa-resource-name>)
                              n206 = Add(x=w295, y=w291) -> (x+y=w294:dbl)
                              n207 = Bundle By Name(cluster=w298, "WV Online TEC"=w294, "Module"=T12."WV Online TEC") -> (w297:T6)
                              n208 = call "TL_Driver_v2.vi"("Device In"=w292, "Commands"=T9."SET", "Settings"=w297) -> ("Readings"=w296:T7)  [unwired: 9 in, 3 out]
                              n209 = local write "Settings"(w297) -> ()
                              n210 = local write "Readings"(w296) -> ()
                            }
                          }
                        }
                      }
                      n211 = Or(x=w244, y="Cancel online") -> (x .or. y?=w243:bool)
                    }
                  }
                  frame #1 {
                    # "Converting to pulse energy, assumes 5 percent pickoff"
                    # "Reading the Newport Power meter"
                    # "Reading the output power of the laser transmitter from the Newport power meter, once read, convert to corresponding pulse energy and plot"
                    n212 = local read "Newport Device Key"() -> (w303:string)
                    n213 = local read "NewportRef"() -> (w299:refnum<k24>)
                    n214 = disable-structure shown="Disabled" {
                      frame Disabled {
                        # "Plotting the online and offling pulse energies"
                        n215 = local read "Online Pulse Energy"() -> (w314:dbl)
                        n216 = local read "Offline Pulse Energy"() -> (w313:dbl)
                        n217 = Bundle("Online Pulse Energy"=w314, "Offline Pulse Energy"=w313) -> (→"Pulse Energy (Micro Joule)":T15)  [unwired: 1 in]
                      }
                      frame Enabled {
                      }
                    }
                    n218 = Number To Decimal String(number="SampleSize") -> (decimal integer string=w301:string)  [unwired: 1 in]
                    n219 = invoke class="PowerMeterCommands" method="PerformDAQ"(reference=w299, "deviceKey"=w303, "interval"="1", "sampleSize"=w301) -> ("PerformDAQ"=w304:dbl[])  [unwired: 2 in, 5 out]
                    n220 = call-poly <vilib>:"Mean.vi"("X"=w304) -> ("mean"=w302:dbl)  [unwired: 1 out]
                    n221 = Multiply(x=w302, y=1000.0) -> (x*y=w310:dbl)
                    n222 = Divide(x=w310, y=0.05) -> (x/y=w308:dbl)
                    n223 = Divide(x=w308, y=7.0) -> (x/y=→"Online Pulse Energy":dbl)
                  }
                  frame #2 {
                    # "Wait 'Scalar Wait Time' for the next available batch of scalar card data"
                    n224 = local read "AMCS_Profile"() -> (w315:i32)
                    n225 = disable-structure shown="Disabled" {
                      frame Disabled {
                        # "Waiting 'Scalar Wait Time'"
                        n226 = Wait (ms)(milliseconds to wait="Scalar Wait Time") -> ()  [unwired: 1 out]
                      }
                      frame Enabled {
                      }
                    }
                    n227 = while {
                      tunnel: [w322] -> w316
                      tunnel: [w318] -> _
                      tunnel: w315 -> [w318]
                      stop <- w320 stop-if-true
                      n228 = global read "AMCS_Data.vi" "AMCS_Profile"() -> (w322:i32)
                      n229 = Wait (ms)(milliseconds to wait=u32 10) -> ()  [unwired: 1 out]
                      n230 = Equal?(x=w322, y=w318) -> (x = y?=w321:bool)
                      n231 = case shown="False" w321 {
                        tunnel: [TRUE FALSE] -> w320
                        frame False {
                        }
                        frame True {
                        }
                      }
                    }
                    "AMCS_Profile" <- w316
                  }
                  frame #3 {
                    # "convert time per range bin to meters\nand calculate smoothed bins using\nsmoothing range"
                    # "Plotting online cross section and smoothed online data"
                    # "Calculate the bin by bin mean of the data"
                    # "Collect 'Integration Period (Seconds)' number\nof scalar data"
                    # "Reading, processing, and plotting the online data"
                    n232 = local read "Data Reads (number of loops)"() -> (w350:i32)
                    n233 = for {
                      N: w350 -> [_]
                      tunnel: [w371] -> w362 mode=indexing
                      tunnel: [w370] -> w325 mode=indexing
                      # "Scalar Data is retrieved from Global \nVariable that scaler.vi is writing to,"
                      n234 = global read "AMCS_Data.vi" "AMCS_Data"() -> (w374:u16[][])
                      n235 = disable-structure shown="Disabled" {
                        frame Disabled {
                          n236 = global read "Scalar_Data_3.vi" "Scalar Data 3"() -> ()  [unwired: 1 out]
                          n237 = global read "Scalar_Data.vi" "Scalar Data"() -> ()  [unwired: 1 out]
                        }
                        frame Enabled {
                        }
                      }
                      n238 = Index Array(array=w374, index (row) #1=0 ("index (row)"), index (row) #2=2 ("index (row)")) -> (element #1=w371:u16[], element #2=w370:u16[])  [unwired: 2 in]
                    }
                    n239 = Transpose 2D Array(2D array=w362) -> (transposed array=w366:u16[][])
                    n240 = Transpose 2D Array(2D array=w325) -> (transposed array=w348:u16[][])
                    n241 = for {
                      tunnel: w366 -> [w376] mode=indexing
                      tunnel: [w375] -> w367 mode=indexing
                      n242 = call-poly <vilib>:"Mean.vi"("X"=w376) -> ("mean"=w375:dbl)  [unwired: 1 out]
                    }
                    n243 = for {
                      tunnel: w348 -> [w369] mode=indexing
                      tunnel: [w368] -> w349 mode=indexing
                      n244 = call-poly <vilib>:"Mean.vi"("X"=w369) -> ("mean"=w368:dbl)  [unwired: 1 out]
                    }
                    n245 = local read "bins"() -> (w342:u32)
                    n246 = Array Subset(array=w367, index=1 ("dimension size"), length=w342) -> (w354:dbl[])
                    n247 = Array Subset(array=w349, index=1 ("dimension size"), length=w342) -> (w346:dbl[])
                    n248 = local read "background length"() -> (w332:i32)
                    n249 = local read "background start"() -> (w333:u32)
                    n250 = Array Size(array=w354) -> (size(s)=w351:i32)
                    n251 = Array Size(array=w346) -> (size(s)=w343:i32)
                    n252 = Initialize Array(1.0 ("element"), w351) -> (w353:dbl[])
                    n253 = Initialize Array(1.0 ("element"), w343) -> (w345:dbl[])
                    n254 = Multiply(x=w354, y=w353) -> (x*y=w355:dbl[])
                    "CH 0 Bin Readings" <- w355
                    n255 = Multiply(x=w346, y=w345) -> (x*y=w336:dbl[])
                    "CH 2 Bin Readings" <- w336
                    n256 = local read "Total DIAL Integration Time (Minutes)"() -> (w358:i32)
                    n257 = local read "Time Resolution Per Bin(ns)"() -> (w328:u32)
                    n258 = Array Subset(array=w355, index=w333, length=w332) -> (w364:dbl[])
                    n259 = Array Subset(array=w336, index=w333, length=w332) -> (w338:dbl[])
                    n260 = call-poly <vilib>:"Mean.vi"("X"=w364) -> ("mean"=w363:dbl)  [unwired: 1 out]
                    n261 = call-poly <vilib>:"Mean.vi"("X"=w338) -> ("mean"=w339:dbl)  [unwired: 1 out]
                    n262 = Divide(x=w358, y=w350) -> (x/y=w356:dbl)
                    n263 = local read "Index"() -> (w337:i32)
                    n264 = Subtract(x=w355, y=w363) -> (x-y=w360:dbl[])
                    n265 = Subtract(x=w336, y=w339) -> (x-y=w340:dbl[])
                    n266 = To Double Precision Float(number=w328) -> (double precision float=w329:dbl)
                    n267 = Multiply(x=w356, y=60.0) -> (x*y=w334:dbl)
                    n268 = Multiply(x=w329, y=0.15) -> (x*y=w331:dbl)
                    n269 = call "Ring Buffer Online Near.vi"("Index"=w337, "Profiles to Average"=w334, "Input Array"=w340) -> ("AvgArray"=w341:dbl[])  [unwired: 7 in, 1 out]
                    n270 = call "Ring Buffer Online Far.vi"("Index"=w337, "Profiles to Average"=w334, "Input Array"=w360) -> ("AvgArray"=w359:dbl[])  [unwired: 7 in, 1 out]
                    n271 = Divide(x="Smoothing Range", y=w331) -> (x/y=w326:dbl)
                    "Smoothed Bins" <- w326
                    n272 = call "Smooth Arrray.vi"("smooth size"=w326, "Raw Array"=w359) -> ("Smoothed Array"=→"CH0 (WV on) smoothed":dbl[])  [unwired: 9 in]
                    n273 = call "Smooth Arrray.vi"("smooth size"=w326, "Raw Array"=w341) -> ("Smoothed Array"=→"CH2 (molecular) smoothed":dbl[])  [unwired: 9 in]
                    n274 = disable-structure shown="Disabled" {
                      frame Disabled {
                        n275 = script code="format long;\ncounts=sum(Online);\nif counts >=0.5e6\ntime=time;\nelse\ntime=time\nend"() -> ()  [unwired: 3 in, 2 out]
                      }
                      frame Enabled {
                      }
                    }
                  }
                  frame #4 {
                    # "Toggling the Agiltron switch to the offline DBR seed laser"
                    n276 = disable-structure shown="Disabled" {
                      frame Disabled {
                        n277 = flat-sequence {
                          frame #0 {
                            # "Second one"
                            # "Command the switch to switch to position 2\ncorresponding to the offline DBR"
                            # "Hex string command \ncorrespond to offline"
                            n278 = VISA Write(VISA resource name="Switch Comm Port", write buffer="\u0001\u0012\u0000\u0001") -> ()  [unwired: 1 in, 3 out]
                          }
                        }
                      }
                      frame Enabled {
                      }
                    }
                  }
                  frame #5 {
                    # "Save the recently collected online data if 'Save Data?' is true"
                    n279 = case shown="True" "Save Data?" {
                      frame False {
                        # "'Save Data?' is false, do nothing"
                      }
                      frame True {
                        # "'Save Data?' is true, save onfline data to the Data Disk"
                        # "Write only one copy of data at this time"
                        # "Retrieve Julian Date"
                        n280 = local read "Readings"() -> (w382:T7)
                        n281 = local read "Time Resolution Per Bin(ns)"() -> (w390:u32)
                        n282 = Unbundle By Name(w382) -> ("WV OnLine TEC"=w381:dbl)
                        n283 = local read "Number of Accumulates"() -> (w388:u32)
                        n284 = Unbundle By Name(w382) -> ("HSRL TEC"=w380:dbl)
                        n285 = local read "WV Online Read (nm)"() -> (w383:dbl)
                        n286 = local write "DataOpen"(TRUE ("DataOpen")) -> ()
                        n287 = local read "Number of Bins"() -> (w389:u32)
                        n288 = local read "HSRL Read (nm)"() -> (w384:dbl)
                        n289 = local read "Online Pulse Energy"() -> (w411:dbl)
                        n290 = local read "CH 0 Bin Readings"() -> (w413:dbl[])
                        n291 = To Double Precision Float(number=w390) -> (double precision float=w385:dbl)
                        n292 = To Double Precision Float(number=w389) -> (double precision float=w386:dbl)
                        n293 = To Double Precision Float(number=w388) -> (double precision float=w387:dbl)
                        n294 = local read "CH 2 Bin Readings"() -> (w410:dbl[])
                        n295 = call "Julian_Date_2.vi"() -> ("Julian Date"=w412:dbl)  [unwired: 11 in]
                        n296 = Build Array (concatenate)(w412, w383, w381, w411, w385, w386, w387, w413) -> (w405:dbl[])
                        n297 = Build Array (concatenate)(w412, w384, w380, w411, w385, w386, w387, w410) -> (w395:dbl[])
                        n298 = local read "NF_On_Ref"() -> (w393:refnum<file>)
                        n299 = local read "FF_On_Ref"() -> (w409:refnum<file>)
                        n300 = local read "NF_On_Ptr"() -> (w394:i64)
                        n301 = local read "FF_On_Ptr"() -> (w408:i64)
                        n302 = Set File Position(offset (in bytes) (0)=w408, refnum=w409) -> (refnum out=w406:refnum<file>, error out=w403:errorcluster)  [unwired: 2 in]
                        n303 = Set File Position(offset (in bytes) (0)=w394, refnum=w393) -> (refnum out=w399:refnum<file>, error out=w397:errorcluster)  [unwired: 2 in]
                        n304 = Write to Binary File(file (use dialog)=w399, data=w395, error in=w397, 5:FALSE ("prepend array or string size? (T)")) -> (refnum out=w398:refnum<file>, error out=w396:errorcluster)  [unwired: 2 in, 1 out]
                        n305 = Write to Binary File(file (use dialog)=w406, data=w405, error in=w403, 5:FALSE ("prepend array or string size? (T)")) -> (refnum out=w404:refnum<file>, error out=w402:errorcluster)  [unwired: 2 in, 1 out]
                        n306 = Get File Position(4:w396, 7:w398) -> (2:w392:i64)  [unwired: 2 out]
                        n307 = Get File Position(4:w402, 7:w404) -> (2:w401:i64)  [unwired: 2 out]
                        n308 = local write "NF_On_Ptr"(w392) -> ()
                        n309 = local write "FF_On_Ptr"(w401) -> ()
                      }
                    }
                  }
                }
              }
              frame #3 {
                # "Frame 3: Read offline data, calculate aerosol data, and plot offline and normalized relative backscatter\nFrame 4:\nFrame 5: Save the offline data and related information"
                # "Frame 0: Read the offline wavelength and lock if necessary, Switch to online DBR\nFrame 1: Read the output power from the Newport power meter\nFrame 2: Wait 'Scalar Wait Time' for buffers to clear of online contiminated data"
                # "offline"
                n310 = stacked-sequence {
                  frame #0 {
                    # "Following Locking the Offline wavelength, check and lock the HSRL 780 nm wavelength"
                    # "Every 60 data collection cycles, read the offline DBR wavelength, and if outside of wavelength tolerance, adjust DBR current until within tolerance"
                    n311 = local read "L_Count"() -> (w415:i32)
                    n312 = Quotient & Remainder(x=w415, y=60.0) -> (x-y*floor(x/y)=w416:dbl)  [unwired: 1 out]
                    n313 = Equal To 0?(x=w416) -> (x = 0?=w414:bool)
                    n314 = case shown="True" w414 {
                      frame False {
                      }
                      frame True {
                        n315 = flat-sequence {
                          frame #0 {
                            n316 = while {
                              i -> [w421]
                              stop <- w419 stop-if-true
                              # "If WL difference is within tolerance, stop looping, and illuminate 'Wavelength Lock Offline' indicator"
                              # "Frame 2: Decrement DBR if above tolerance\nFrame 3: Increment DBR if below tolerance"
                              # "Frame 0: Read the wavelength from the wavemeter\nFrame 1: Calculate the difference between desired and actual wavelength"
                              # "Continue reading and adjusting offline DBR until within locking tolerance"
                              n317 = stacked-sequence {
                                tunnel: w421 -> [w423 _ _ _ _]
                                tunnel: [_ _ w437 _ _] -> w418
                                frame #0 {
                                n318 = Equal To 0?(x=w423) -> (x = 0?=w422:bool)
                                n319 = case shown="True" w422 {
                                frame False {
                                }
                                frame True {
                                # "Set the TSOA switch to\namplify the non ABSORBING\nwavelength"
                                n320 = Build Array(TRUE ("Boolean")) -> (w425:bool[])
                                n321 = call-poly <vilib>:"DAQmx Write.vi"("task/channels in"=refnum<k21> "BristolWM", "data"=w425) -> ()  [unwired: 11 in, 3 out]
                                n322 = Wait (ms)(milliseconds to wait=u32 3200) -> ()  [unwired: 1 out]
                                }
                                }
                                }
                                frame #1 {
                                # "Reading the wavelength from the wavemeter"
                                n323 = flat-sequence {
                                tunnel: [w430] -> w429
                                tunnel: w429 -> [w433]
                                tunnel: [w432] -> w428
                                tunnel: w428 -> [w436]
                                frame #0 {
                                n324 = local read "Bristol In"() -> (w431:i32)
                                n325 = dll-call lib="C:/Users/H2ODial/Desktop/Shared Telescope WV DIAL Code/bristol/CLDevIface.dll" fn="CLOpenUSBSerialDevice"("commPort"=w431) -> ("return type"=w430:i32)  [unwired: 4 in, 2 out]
                                }
                                frame #1 {
                                n326 = dll-call lib="C:/Users/H2ODial/Desktop/Shared Telescope WV DIAL Code/bristol/CLDevIface.dll" fn="CLGetLambdaReading"("devHandle"=w433) -> ("return type"=→"WV Offline Read (nm)":dbl, "devHandle"=w432:i32)  [unwired: 3 in, 2 out]
                                }
                                frame #2 {
                                n327 = dll-call lib="C:/Users/H2ODial/Desktop/Shared Telescope WV DIAL Code/bristol/CLDevIface.dll" fn="CLCloseDevice"("commPort"=w436) -> ("return type"=w435:i32)  [unwired: 4 in, 2 out]
                                n328 = local write "Bristol Out"(w435) -> ()
                                }
                                }
                                }
                                frame #2 {
                                # "Calculating the difference between the actual and desired online wavelength"
                                n329 = local read "Offline_Tol"() -> (w439:dbl)
                                n330 = local read "WV Offline Read (nm)"() -> (w445:dbl)
                                n331 = Multiply(x=-1.0, y=w439) -> (x*y=w438:dbl)
                                n332 = Subtract(x=w445, y="WV Offline Set (nm)") -> (x-y=w441:dbl)
                                "Oflline_Diff" <- w441
                                n333 = Greater?(x=w441, y=w438) -> (0:w442:bool)
                                n334 = Less?(x=w441, y=w439) -> (x < y?=w443:bool)
                                n335 = And(x=w442, y=w443) -> (x .and. y?=w437:bool)
                                "WV Oflline Locked" <- w437
                                n336 = case shown="True" w437 {
                                frame False {
                                }
                                frame True {
                                # "Set the Wavemeter switch to\nthe HSRL wavelength"
                                n337 = Build Array(TRUE ("Boolean")) -> (w447:bool[])
                                n338 = call-poly <vilib>:"DAQmx Write.vi"("task/channels in"=refnum<k21> "HSRL_WV_switch", "data"=w447) -> ()  [unwired: 11 in, 3 out]
                                n339 = Wait (ms)(milliseconds to wait=u32 3200) -> ()  [unwired: 1 out]
                                }
                                }
                                }
                                frame #3 {
                                # "If the wavelength difference is greater that 0.0002 nm, decrement the \nDBR current by 0.01 mA"
                                n340 = local read "Oflline_Diff"() -> (w452:dbl)
                                n341 = Greater Or Equal?(x=w452, y="Offline_Tol") -> (x >= y?=w451:bool)
                                n342 = case shown="True" w451 {
                                frame False {
                                # "Wavelength difference is not greater than 0.0002 nm, do nothing"
                                }
                                frame True {
                                # "Generating a command string\nto decrement the current"
                                n343 = local read "Settings"() -> (w459:T6)
                                n344 = Unbundle By Name(w459) -> ("WV Offline TEC"=w457:dbl)
                                n345 = Subtract(x=w457, y="temp step size") -> (x-y=w456:dbl)
                                n346 = local read "Device In"() -> (w454:refnum<visa-resource-name>)
                                n347 = Bundle By Name(cluster=w459, "WV Offline TEC"=w456, "Module"=T12."WV Offline TEC") -> (w460:T6)
                                n348 = call "TL_Driver_v2.vi"("Device In"=w454, "Commands"=T9."SET", "Settings"=w460) -> ("Readings"=w461:T7)  [unwired: 9 in, 3 out]
                                n349 = local write "Settings"(w460) -> ()
                                n350 = local write "Readings"(w461) -> ()
                                }
                                }
                                }
                                frame #4 {
                                # "If WL difference is < 0.0002 nm, increment the DBR temperature"
                                n351 = local read "Oflline_Diff"() -> (w464:dbl)
                                n352 = Less Or Equal?(x=w464, y=-0.0001) -> (x <= y?=w462:bool)
                                n353 = case shown="True" w462 {
                                frame False {
                                # "WL difference is no <= to -0.0002 nm, do nothing"
                                }
                                frame True {
                                # "Generating a command string\nto decrement the current"
                                # "WL difference is less than 0.0002 nm,\nincrement the DBR current by 0.01 mA"
                                n354 = local read "Settings"() -> (w472:T6)
                                n355 = Unbundle By Name(w472) -> ("WV Offline TEC"=w470:dbl)
                                n356 = local read "temp step size"() -> (w466:dbl)
                                n357 = Add(x=w470, y=w466) -> (x+y=w469:dbl)
                                n358 = local read "Device In"() -> (w467:refnum<visa-resource-name>)
                                n359 = Bundle By Name(cluster=w472, "WV Offline TEC"=w469, "Module"=T12."WV Offline TEC") -> (w473:T6)
                                n360 = call "TL_Driver_v2.vi"("Device In"=w467, "Commands"=T9."SET", "Settings"=w473) -> ("Readings"=w471:T7)  [unwired: 9 in, 3 out]
                                n361 = local write "Settings"(w473) -> ()
                                n362 = local write "Readings"(w471) -> ()
                                }
                                }
                                }
                              }
                              n363 = Or(x=w418, y="Cancel Offline") -> (x .or. y?=w419:bool)
                            }
                          }
                          frame #1 {
                            n364 = while {
                              i -> [w477]
                              stop <- w475 stop-if-true
                              # "If WL difference is within tolerance, stop looping, and illuminate 'Wavelength Lock Offline' indicator"
                              # "Frame 2: Decrement DBR if above tolerance\nFrame 3: Increment DBR if below tolerance"
                              # "Frame 0: Read the wavelength from the wavemeter\nFrame 1: Calculate the difference between desired and actual wavelength"
                              # "Continue reading and adjusting offline DBR until within locking tolerance"
                              n365 = stacked-sequence {
                                tunnel: w477 -> [w479 _ _ _ _]
                                tunnel: [_ _ w492 _ _] -> w474
                                frame #0 {
                                n366 = Equal To 0?(x=w479) -> (x = 0?=w478:bool)
                                n367 = case shown="True" w478 {
                                frame False {
                                }
                                frame True {
                                # "Set the Wavemeter to\nthe non HSRL wavelength"
                                n368 = Build Array(TRUE ("Boolean")) -> (w480:bool[])
                                n369 = call-poly <vilib>:"DAQmx Write.vi"("task/channels in"=refnum<k21> "HSRL_WV_switch", "data"=w480) -> ()  [unwired: 11 in, 3 out]
                                }
                                }
                                }
                                frame #1 {
                                # "Reading the wavelength from the wavemeter"
                                n370 = flat-sequence {
                                tunnel: [w485] -> w484
                                tunnel: w484 -> [w488]
                                tunnel: [w487] -> w483
                                tunnel: w483 -> [w491]
                                frame #0 {
                                n371 = local read "Bristol In"() -> (w486:i32)
                                n372 = dll-call lib="C:/Users/H2ODial/Desktop/Shared Telescope WV DIAL Code/bristol/CLDevIface.dll" fn="CLOpenUSBSerialDevice"("commPort"=w486) -> ("return type"=w485:i32)  [unwired: 4 in, 2 out]
                                }
                                frame #1 {
                                n373 = dll-call lib="C:/Users/H2ODial/Desktop/Shared Telescope WV DIAL Code/bristol/CLDevIface.dll" fn="CLGetLambdaReading"("devHandle"=w488) -> ("return type"=→"HSRL Read (nm)":dbl, "devHandle"=w487:i32)  [unwired: 3 in, 2 out]
                                }
                                frame #2 {
                                n374 = dll-call lib="C:/Users/H2ODial/Desktop/Shared Telescope WV DIAL Code/bristol/CLDevIface.dll" fn="CLCloseDevice"("commPort"=w491) -> ("return type"=w490:i32)  [unwired: 4 in, 2 out]
                                n375 = local write "Bristol Out"(w490) -> ()
                                }
                                }
                                }
                                frame #2 {
                                # "Calculating the difference between the actual and desired online wavelength"
                                n376 = local read "HSRL_Tol"() -> (w494:dbl)
                                n377 = local read "HSRL Read (nm)"() -> (w500:dbl)
                                n378 = Multiply(x=-1.0, y=w494) -> (x*y=w493:dbl)
                                n379 = Subtract(x=w500, y="HSRL Set (nm)") -> (x-y=w496:dbl)
                                "HSRL_Diff" <- w496
                                n380 = Greater?(x=w496, y=w493) -> (0:w497:bool)
                                n381 = Less?(x=w496, y=w494) -> (x < y?=w498:bool)
                                n382 = And(x=w497, y=w498) -> (x .and. y?=w492:bool)
                                "HSRL Locked" <- w492
                                n383 = case shown="True" w492 {
                                frame False {
                                }
                                frame True {
                                # "Set the Wavementer switch to WV Online"
                                n384 = Build Array(FALSE ("Boolean")) -> (w501:bool[])
                                n385 = Build Array(FALSE ("Boolean")) -> (w505:bool[])
                                n386 = call-poly <vilib>:"DAQmx Write.vi"("task/channels in"=refnum<k21> "BristolWM", "data"=w505) -> ()  [unwired: 11 in, 3 out]
                                n387 = call-poly <vilib>:"DAQmx Write.vi"("task/channels in"=refnum<k21> "HSRL_WV_switch", "data"=w501) -> ()  [unwired: 11 in, 3 out]
                                n388 = Wait (ms)(milliseconds to wait=u32 3200) -> ()  [unwired: 1 out]
                                }
                                }
                                }
                                frame #3 {
                                # "If the wavelength difference is greater that 0.0002 nm, decrement the \nDBR current by 0.01 mA"
                                n389 = local read "HSRL_Diff"() -> (w510:dbl)
                                n390 = Greater Or Equal?(x=w510, y="HSRL_Tol") -> (x >= y?=w509:bool)
                                n391 = case shown="True" w509 {
                                frame False {
                                # "Wavelength difference is not greater than 0.0002 nm, do nothing"
                                }
                                frame True {
                                # "Generating a command string\nto decrement the current"
                                n392 = local read "Settings"() -> (w517:T6)
                                n393 = local read "temp step size"() -> (w511:dbl)
                                n394 = Unbundle By Name(w517) -> ("HSRL TEC"=w516:dbl)
                                n395 = Subtract(x=w516, y=w511) -> (x-y=w515:dbl)
                                n396 = local read "Device In"() -> (w513:refnum<visa-resource-name>)
                                n397 = Bundle By Name(cluster=w517, "HSRL TEC"=w515, "Module"=T12."HSRL TEC") -> (w518:T6)
                                n398 = call "TL_Driver_v2.vi"("Device In"=w513, "Commands"=T9."SET", "Settings"=w518) -> ("Readings"=w519:T7)  [unwired: 9 in, 3 out]
                                n399 = local write "Settings"(w518) -> ()
                                n400 = local write "Readings"(w519) -> ()
                                }
                                }
                                }
                                frame #4 {
                                # "If WL difference is < 0.0002 nm, increment the DBR temperature"
                                n401 = local read "HSRL_Diff"() -> (w522:dbl)
                                n402 = Less Or Equal?(x=w522, y=-0.0001) -> (x <= y?=w520:bool)
                                n403 = case shown="True" w520 {
                                frame False {
                                # "WL difference is no <= to -0.0002 nm, do nothing"
                                }
                                frame True {
                                # "Generating a command string\nto decrement the current"
                                # "WL difference is less than 0.0002 nm,\nincrement the DBR current by 0.01 mA"
                                n404 = local read "Settings"() -> (w530:T6)
                                n405 = local read "temp step size"() -> (w523:dbl)
                                n406 = Unbundle By Name(w530) -> ("HSRL TEC"=w528:dbl)
                                n407 = Add(x=w528, y=w523) -> (x+y=w527:dbl)
                                n408 = local read "Device In"() -> (w525:refnum<visa-resource-name>)
                                n409 = Bundle By Name(cluster=w530, "HSRL TEC"=w527, "Module"=T12."HSRL TEC") -> (w531:T6)
                                n410 = call "TL_Driver_v2.vi"("Device In"=w525, "Commands"=T9."SET", "Settings"=w531) -> ("Readings"=w529:T7)  [unwired: 9 in, 3 out]
                                n411 = local write "Settings"(w531) -> ()
                                n412 = local write "Readings"(w529) -> ()
                                }
                                }
                                }
                              }
                              n413 = Or(x=w474, y="Cancel HSRL") -> (x .or. y?=w475:bool)
                            }
                          }
                        }
                      }
                    }
                  }
                  frame #1 {
                    # "Reading the power meter"
                    # "Updating the pulse energy plot"
                    # "Converting to pulse energy"
                    # "Reading the offline output power, converting to pulse energy,  and updating the Pulse energy plot"
                    n414 = local read "SampleSize"() -> (w534:i32)
                    n415 = local read "Newport Device Key"() -> (w535:string)
                    n416 = local read "Online Pulse Energy"() -> (w541:dbl)
                    n417 = local read "Offline Pulse Energy"() -> (w540:dbl)
                    n418 = local read "NewportRef"() -> (w532:refnum<k24>)
                    n419 = Number To Decimal String(number=w534) -> (decimal integer string=w536:string)  [unwired: 1 in]
                    n420 = invoke class="PowerMeterCommands" method="PerformDAQ"(reference=w532, "deviceKey"=w535, "interval"="1", "sampleSize"=w536) -> ("PerformDAQ"=w537:dbl[])  [unwired: 2 in, 5 out]
                    n421 = Bundle("Online Pulse Energy"=w541, "Offline Pulse Energy"=w540) -> (w539:T15)  [unwired: 1 in]
                    n422 = local write "Pulse Energy (Micro Joule)"(w539) -> ()
                    n423 = call-poly <vilib>:"Mean.vi"("X"=w537) -> ("mean"=w533:dbl)  [unwired: 1 out]
                    n424 = Multiply(x=w533, y=1000.0) -> (x*y=w546:dbl)
                    n425 = Divide(x=w546, y=0.05) -> (x/y=w544:dbl)
                    n426 = Divide(x=w544, y=7.0) -> (x/y=→"Offline Pulse Energy":dbl)
                  }
                  frame #2 {
                    # "Added in the ability to interactively control the ThorLab  setting (just etalon temp for now)"
                    # "Wait 'Scalar Wait Time' for buffers to clear of online contiminated offline data"
                    n427 = disable-structure shown="Disabled" {
                      frame Disabled {
                        # "Wait 'Scalar Wait Time'"
                        n428 = local read "Scalar Wait Time"() -> (w556:u32)
                        n429 = Wait (ms)(milliseconds to wait=w556) -> ()  [unwired: 1 out]
                      }
                      frame Enabled {
                      }
                    }
                    n430 = event shown="[1] \"Settings.WV Etalon TEC\": Value Change" {
                      selector: _ -> [_ _]
                      dyn-events: _ -> [_ _]
                      timeout: 1 -> [_ _]
                      event Timeout {
                        n431 = event-data() -> ()  [unwired: 1 in, 2 out]
                      }
                      event "Settings.WV Etalon TEC": Value Change {
                        # "Generating a command string\nto update the etalon"
                        n432 = event-data() -> ()  [unwired: 1 in, 5 out]
                        n433 = local read "Settings"() -> (w553:T6)
                        n434 = Unbundle By Name(w553) -> ("WV Etalon TEC"=w555:dbl)
                        n435 = Bundle By Name(cluster=w553, "WV Etalon TEC"=w555, "Module"=T12."WV Etalon TEC") -> (w551:T6)
                        n436 = call "TL_Driver_v2.vi"("Device In"=refnum<visa-resource-name> "Pro8000", "Commands"=T9."SET", "Settings"=w551) -> ("Readings"=w552:T7)  [unwired: 9 in, 3 out]
                        n437 = local write "Readings"(w552) -> ()
                        n438 = local write "Settings"(w551) -> ()
                      }
                    }
                  }
                  frame #3 {
                    w583 = 1 ("dimension size")
                    # "Read in latest scalar card data from \n'Scalar Data' global variable that \nscaler.vi is writing to, then wait 1 sec\nfor next batch of data"
                    # "Calculating/Plotting smoothed data,\ncross sections etc."
                    # "Pick off data with\nout header"
                    # "Calculate mean bin by bin mean"
                    # "Reading in 'Integration Period (Seconds)' of data"
                    # "Read the offline data from the scalar card, perform smoothing, calculate normalized relative backscatter, and plot"
                    # "Collects Data From Card,\nSends It To The Chart,\nAnd Saves A Copy As A\nFile If Option Selected On\nFront Panel"
                    n439 = for {
                      N: "Data Reads (number of loops)" -> [_]
                      tunnel: [w641] -> w572 mode=indexing
                      tunnel: [w640] -> w571 mode=indexing
                      n440 = global read "AMCS_Data.vi" "AMCS_Data"() -> (w642:u16[][])
                      n441 = disable-structure shown="Disabled" {
                        frame Disabled {
                          n442 = global read "Scalar_Data_4.vi" "Scalar Data 4"() -> ()  [unwired: 1 out]
                          n443 = global read "Scalar_Data_2.vi" "Scalar Data 2"() -> ()  [unwired: 1 out]
                        }
                        frame Enabled {
                        }
                      }
                      n444 = Index Array(array=w642, index (row) #1=1 ("index (row)"), index (row) #2=3 ("index (row)")) -> (element #1=w641:u16[], element #2=w640:u16[])  [unwired: 2 in]
                    }
                    n445 = local read "Total DIAL Integration Time (Minutes)"() -> (w603:i32)
                    n446 = Divide(x=w603, y="Data Reads (number of loops)") -> (x/y=w601:dbl)
                    n447 = local read "Total Aerosol Integration Time (Minutes)"() -> (w605:dbl)
                    n448 = Multiply(x=w601, y=60.0) -> (x*y=w589:dbl)
                    n449 = local read "background length"() -> (w576:i32)
                    n450 = local read "background start"() -> (w577:u32)
                    n451 = Transpose 2D Array(2D array=w572) -> (transposed array=w611:u16[][])
                    n452 = Transpose 2D Array(2D array=w571) -> (transposed array=w595:u16[][])
                    n453 = Divide(x=w605, y="Data Reads (number of loops)") -> (x/y=w606:dbl)
                    n454 = for {
                      tunnel: w611 -> [w648] mode=indexing
                      tunnel: [w647] -> w612 mode=indexing
                      tunnel: w595 -> [w646] mode=indexing
                      tunnel: [w645] -> _ mode=indexing
                      tunnel: [w645] -> w592 mode=indexing
                      n455 = call-poly <vilib>:"Mean.vi"("X"=w648) -> ("mean"=w647:dbl)  [unwired: 1 out]
                      n456 = call-poly <vilib>:"Mean.vi"("X"=w646) -> ("mean"=w645:dbl)  [unwired: 1 out]
                    }
                    n457 = local read "bins"() -> (w584:u32)
                    n458 = Multiply(x=w606, y=60.0) -> (x*y=w568:dbl)
                    n459 = Array Subset(array=w592, index=w583, length=w584) -> (w593:dbl[])
                    "CH3 Bin Readings" <- w593
                    n460 = Array Subset(array=w612, index=w583, length=w584) -> (w591:dbl[])
                    "CH1  Bin Readings" <- w591
                    n461 = Array Subset(array=w593, index=w577, length=w576) -> (w594:dbl[])
                    n462 = Array Subset(array=w591, index=w577, length=w576) -> (w610:dbl[])
                    n463 = local read "Smoothed Bins"() -> (w573:dbl)
                    n464 = call-poly <vilib>:"Mean.vi"("X"=w594) -> ("mean"=w558:dbl)  [unwired: 1 out]
                    n465 = call-poly <vilib>:"Mean.vi"("X"=w610) -> ("mean"=w561:dbl)  [unwired: 1 out]
                    n466 = local read "Index"() -> (w569:i32)
                    n467 = Subtract(x=w593, y=w558) -> (x-y=w570:dbl[])
                    n468 = Subtract(x=w591, y=w561) -> (x-y=w587:dbl[])
                    n469 = call "Ring Buffer Offline Far.vi"("Index"=w569, "Profiles to Average"=w589, "Input Array"=w587) -> ("AvgArray"=w608:dbl[], "RingBufferOut"=→"CH1 RingBuffer long":dbl[][])  [unwired: 7 in]
                    n470 = call "Ring Buffer Aerosol Far.vi"("Index"=w569, "Profiles to Average"=w568, "Input Array"=w587) -> ("AvgArray"=w604:dbl[], "RingBufferOut"=→"CH1 RingBuffer short":dbl[][])  [unwired: 7 in]
                    n471 = call "Ring Buffer Offline Near.vi"("Index"=w569, "Profiles to Average"=w589, "Input Array"=w570) -> ("AvgArray"=w590:dbl[], "RingBufferOut"=→"CH3 RingBuffer long":dbl[][])  [unwired: 7 in]
                    n472 = call "Ring Buffer Aerosol Near.vi"("Index"=w569, "Profiles to Average"=w568, "Input Array"=w570) -> ("AvgArray"=w580:dbl[], "RingBufferOut"=→"CH3 RingBuffer short":dbl[][])  [unwired: 7 in]
                    n473 = Reshape Array(w587, w583, w584) -> (→"CH 1 (WV off) counts display":dbl[][])
                    n474 = Reshape Array(w570, w583, w584) -> (→"CH 3 (HSRL comb) counts display":dbl[][])
                    n475 = call "Smooth Arrray.vi"("smooth size"=w573, "Raw Array"=w608) -> ("Smoothed Array"=→"CH1 (WV off) smooth S":dbl[])  [unwired: 9 in]
                    n476 = call "Smooth Arrray.vi"("smooth size"=w573, "Raw Array"=w604) -> ("Smoothed Array"=w582:dbl[])  [unwired: 9 in]
                    "CH1 (WV off) smooth L" <- w582
                    n477 = call "Smooth Arrray.vi"("smooth size"=w573, "Raw Array"=w590) -> ("Smoothed Array"=→"CH3 (HSRL combined) smooth L":dbl[])  [unwired: 9 in]
                    n478 = call "Smooth Arrray.vi"("smooth size"=w573, "Raw Array"=w580) -> ("Smoothed Array"=w575:dbl[])  [unwired: 9 in]
                    "CH3 (HSRL combined) smooth S" <- w575
                    n479 = local read "Time Resolution Per Bin(ns)"() -> (w566:u32)
                    n480 = local read "Number of Accumulates"() -> (w564:u32)
                    n481 = local read "Temperature (C)"() -> (w600:dbl)
                    n482 = local read "Pressure (mb)"() -> (w599:dbl)
                    n483 = Reciprocal(x=w566) -> (1/x=w565:dbl)
                    n484 = disable-structure shown="Disabled" {
                      disable-tunnel: w600 -> [w639 _]
                      disable-tunnel: w599 -> [w638 _]
                      disable-tunnel: w582 -> [w632 _]
                      disable-tunnel: w561 -> [w619 _]
                      disable-tunnel: w558 -> [w618 _]
                      disable-tunnel: w564 -> [w617 _]
                      disable-tunnel: "dead time" -> [w616 _]
                      disable-tunnel: w575 -> [w615 _]
                      disable-tunnel: 6.0 ("Real") -> [w614 _]
                      disable-tunnel: w566 -> [w613 _]
                      frame Disabled {
                        w635 = 1
                        # "Plotting the normalized relative \nbackscatter"
                        # "Calculating the normalized relative backscatter"
                        # "File path in MATLAB script is of old dial is:\nF:\\Micropulse DIAL\\Micropulse DIAL Matlab\\\nFinal Overlap Function.mat')];"
                        n485 = script code="%accum_num=10000;     % scaler card setting number of accumulations\nt_bin = t_bin/1e9                 % scaler card setting time per bin\n%t_d = 37.3e-9;                % APD dead time from spec sheet\n\n% conversion from accumulated counts to count rate  (c/s)\nc_convert = 1./t_bin./accum_num;\nCR_far = p_raw_far.*c_convert;\nCR_near = p_raw_near.*c_convert;\nCR_total_far = (p_raw_far+b_far).*c_convert;\nCR_total_near = (p_raw_near+b_near).*c_convert;\nb_CR_far =b_far.*c_convert;\nb_CR_near =b_near.*c_convert;\n \n% create a range array\nsize_p =  size(p_raw_far,2);\ngate = t_bin*3e8/2;\nr = (gate:gate:size_p*gate)./1e3; \n   \n%APD correction factor\n D_far = 1./(1-(t_d*CR_total_far));\n D_near = 1./(1-(t_d*CR_total_near));\n\n %Calculating normalize relative backscatter profile\n nrb_far = CR_far.*D_far.*r.^2.*1e-6;\n nrb_near = CR_near.*D_near.*r.^2.*1e-6;"("E"=w614, "temp"=w639, "press"=w638, "p_raw_far"=w632, "b_far"=w619, "b_near"=w618, "p_raw_near"=w615, "accum_num"=w617, "t_d"=w616, "t_bin"=w613) -> ("nrb_far"=w627:cdb[], "D_far"=w624:dbl[], "nrb_near"=w626:cdb[], "D_near"=w623:dbl[])  [unwired: 1 in, 1 out]
                        n486 = local read "bins"() -> (w634:u32)
                        n487 = local read "Altitude Array (km)"() -> (w629:dbl[])
                        n488 = Build Array(w627, w626) -> (w631:cdb[][])
                        n489 = Build Array(w624, w623) -> (w622:dbl[][])
                        n490 = Reshape Array(w626, w635, w634) -> (→"NRB 2":cdb[][])
                        n491 = Reshape Array(w627, w635, w634) -> (→"NRB":cdb[][])
                        n492 = Build Array(w629, w629) -> (w628:dbl[][])
                        n493 = call "Convert to Dynamic Data7"("2D Array"=w622) -> ("Dynamic Data Type"=w621:dynamicdata)  [unwired: 3 in]
                        n494 = call "Convert to Dynamic Data3"("2D Array"=w631) -> ("Dynamic Data Type"=w630:dynamicdata)  [unwired: 3 in]
                        n495 = call "Convert to Dynamic Data4"("2D Array"=w628) -> ("Dynamic Data Type"=w625:dynamicdata)  [unwired: 3 in]
                        n496 = call "Build XY Graph2"("Y Input"=w625, "X Input"=w630) -> ("XY Graph"=→"NRB plot":cluster{"Y":dbl[], "Y":dbl[]}[])  [unwired: 3 in, 6 out]
                        n497 = call "Build XY Graph4"("Y Input"=w625, "X Input"=w621) -> ("XY Graph"=→"Correction":cluster{"Y":dbl[], "Y":dbl[]}[])  [unwired: 3 in, 6 out]
                      }
                      frame Enabled {
                      }
                    }
                    n498 = Divide(x=w565, y=w564) -> (x/y=w562:dbl)
                    n499 = Multiply(x=1000000000.0, y=w562) -> (x*y=w559:dbl)
                    n500 = Multiply(x=w559, y=w561) -> (x*y=w560:dbl)
                    n501 = Multiply(x=w559, y=w558) -> (x*y=w557:dbl)
                    n502 = Bundle(w560, w557) -> (→"?":cluster{dbl, dbl})  [unwired: 1 in]
                  }
                  frame #4 {
                    # "REPLACE WITH NEW AGILTRON TASK!"
                    # "Toggle Agiltron switch to online DBR"
                    n503 = disable-structure shown="Disabled" {
                      frame Disabled {
                        # "ABSORBING"
                        n504 = flat-sequence {
                          frame #0 {
                            # "Third one"
                            # "Command the switch to switch to position 1\ncorresponding to the online DBR"
                            # "Hex string command \ncorrespond to online"
                            n505 = local read "Switch Comm Port"() -> (w652:refnum<visa-resource-name>)
                            n506 = VISA Write(VISA resource name=w652, write buffer="\u0001\u0012\u0000\u0002") -> ()  [unwired: 1 in, 3 out]
                          }
                        }
                        n507 = Build Array(FALSE ("Boolean")) -> (w651:bool[])
                        n508 = call-poly <vilib>:"DAQmx Write.vi"("task/channels in"=refnum<k21> "AgiltronSwitch", "data"=w651) -> ()  [unwired: 11 in, 3 out]
                      }
                      frame Enabled {
                      }
                    }
                  }
                  frame #5 {
                    # "If 'Save Data?' is true, save all relavant offline info"
                    n509 = local read "Save Data?"() -> (w654:bool)
                    n510 = case shown="True" w654 {
                      frame False {
                        # "'Save Data?' is false, do nothing"
                      }
                      frame True {
                        # "Write only one data file at this time"
                        # "Retrive Julian Date"
                        # "'Save Data?' is true, save offline data to the Data Disk"
                        n511 = local read "Readings"() -> (w655:T7)
                        n512 = Unbundle By Name(w655) -> ("WV Offline TEC"=w656:dbl)
                        n513 = Unbundle By Name(w655) -> ("HSRL TEC"=w657:dbl)
                        n514 = local read "HSRL Read (nm)"() -> (w658:dbl)
                        n515 = local read "WV Offline Read (nm)"() -> (w679:dbl)
                        n516 = local read "Relative Humdity (%)"() -> (w683:dbl)
                        n517 = local read "CH3 Bin Readings"() -> (w677:dbl[])
                        n518 = local read "CH1  Bin Readings"() -> (w684:dbl[])
                        n519 = local read "Offline Pulse Energy"() -> (w680:dbl)
                        n520 = local read "Temperature (C)"() -> (w681:dbl)
                        n521 = local read "Pressure (mb)"() -> (w682:dbl)
                        n522 = call "Julian_Date_2.vi"() -> ("Julian Date"=w678:dbl)  [unwired: 11 in]
                        n523 = Build Array (concatenate)(w678, w679, w656, w680, w681, w682, w683, w684) -> (w663:dbl[])
                        n524 = Build Array (concatenate)(w678, w658, w657, w680, w681, w682, w683, w677) -> (w660:dbl[])
                        n525 = local read "FF_Off_Ref"() -> (w665:refnum<file>)
                        n526 = local read "NF_Off_Ref"() -> (w662:refnum<file>)
                        n527 = local read "FF_Off_Ptr"() -> (w664:i64)
                        n528 = local read "NF_Off_Ptr"() -> (w661:i64)
                        n529 = Set File Position(offset (in bytes) (0)=w664, refnum=w665) -> (refnum out=w676:refnum<file>, error out=w674:errorcluster)  [unwired: 2 in]
                        n530 = Set File Position(offset (in bytes) (0)=w661, refnum=w662) -> (refnum out=w672:refnum<file>, error out=w670:errorcluster)  [unwired: 2 in]
                        n531 = Write to Binary File(file (use dialog)=w676, data=w663, error in=w674, 5:FALSE ("prepend array or string size? (T)")) -> (refnum out=w675:refnum<file>, error out=w673:errorcluster)  [unwired: 2 in, 1 out]
                        n532 = Write to Binary File(file (use dialog)=w672, data=w660, error in=w670, 5:FALSE ("prepend array or string size? (T)")) -> (refnum out=w671:refnum<file>, error out=w669:errorcluster)  [unwired: 2 in, 1 out]
                        n533 = Get File Position(4:w673, 7:w675) -> (2:w666:i64)  [unwired: 2 out]
                        n534 = Get File Position(4:w669, 7:w671) -> (2:w659:i64)  [unwired: 2 out]
                        n535 = local write "FF_Off_Ptr"(w666) -> ()
                        n536 = local write "NF_Off_Ptr"(w659) -> ()
                      }
                    }
                  }
                }
              }
              frame #4 {
                n537 = First Call?() -> (First Call?: T/F=w687:bool)
                n538 = Or(x="calculate absorption cross sections", y=w687) -> (x .or. y?=w685:bool)
                n539 = case shown="True" w685 {
                  frame False {
                  }
                  frame True {
                    # "calculate absorption cross sections from HITRAN data base"
                  }
                }
              }
              frame #5 {
                # "Data Processing Far Channel"
                # "Calculating the range resolved water vapor number density and plotting"
              }
            }
          }
        }
        "L_Count" <- w132
      }
    }
  }
  n540 = case shown="True" w3 {
    frame False {
    }
    frame True {
      # "close data files"
      n541 = local read "NF_Off_Ref"() -> (w689:refnum<file>)
      n542 = local read "NF_On_Ref"() -> (w690:refnum<file>)
      n543 = local read "FF_Off_Ref"() -> (w691:refnum<file>)
      n544 = local read "FF_On_Ref"() -> (w692:refnum<file>)
      n545 = local read "WS_On/Off"() -> (w688:bool)
      n546 = case shown="True" w688 {
        frame False {
        }
        frame True {
          n547 = local read "WS visa"() -> (w693:refnum<visa-resource-name>)
          n548 = call "T_RH_P.vi"("VISA in"=w693, "WS_Commands"=enum16{"OpenWS", "ReadTRHP", "CloseWS"}."CloseWS") -> ()  [unwired: 11 in, 3 out]
        }
      }
      n549 = Close File(refnum=w692) -> ()  [unwired: 1 in, 2 out]
      n550 = Close File(refnum=w691) -> ()  [unwired: 1 in, 2 out]
      n551 = Close File(refnum=w690) -> ()  [unwired: 1 in, 2 out]
      n552 = Close File(refnum=w689) -> ()  [unwired: 1 in, 2 out]
    }
  }
  "FileHour" <- -1 ("FileHour")
  "DataOpen" <- FALSE
